vi "REPORT XLS PEDROLLO 2.vi"(6 "banco":i32=1, 8 "Report collaudo in corso?":bool, 9 "COLLAUDI DI CONFRONTO":string[](array[string]), 10 "COLLAUDO PRINCIPALE":string) -> ()   [LabVIEW 2019]
uses:
  TypeDef/custom plot legend.ctl
  TypeDef/Grafico report.ctl
  TypeDef/Definizione_Grafico_REPORT.ctl
  TypeDef/Definizione_plot.ctl
  <vilib>/Utility/miscctls.llb/LVRowAndColumnTypeDef.ctl
  Global percorso impostazioni.vi
  <vilib>/Utility/file.llb/Read Delimited Spreadsheet (string).vi
  <vilib>/Utility/file.llb/Read From Spreadsheet File (string).vi
  <vilib>/addons/_office/excel.llb/Excel Easy Table (str).vi
  <vilib>/Utility/file.llb/Write Delimited Spreadsheet (string).vi
  <vilib>/Utility/NIReport.llb/Append Image to Report (path wrap).vi
  <vilib>/addons/database/_DB Variant To Data/Database Variant To Data.xnode
  <vilib>/Utility/NIReport.llb/NI_report.lvclass
  <vilib>/addons/_office/NI_ReportGenerationToolkit.lvlib
  <vilib>/Utility/NIReport.llb/Excel/NI_Excel.lvclass
  <vilib>/addons/database/NI_Database_API.lvlib
panel:
  out "Tipo report":bool
  in  "TABELLA RES FREDDO RES METER":i32(listbox) caption="MISURE RESISTENZE A FREDDO"
  out "state":string
  out "Numeric 2":i32
  out "scelta grafico":u16
  out "modifica":bool
  in  "EXCEL":bool=TRUE
  in  "PDF":bool
  in  "salva impostazioni grafici":bool
  out "ID Colleg confronti":i32[](array[numeric])
  in  "AGGIORNA IMM":bool
  out "Numeric":i32
  in  "Slide":dbl(slide) scale=0.0..100.0
  out "Cartella modello":path
  in  "REPORT C2K":bool caption="C2K"
  out "element":string
  in  "stile punto":u16(ring)
  in  "stile linea":u16(ring)
  in  "Larghezza linea":u16(ring)
  in  "input cluster":T1
  out "ProvaT-DT":cluster{"X":dbl[], "Y":dbl[]}[](graph)
  out "ProvaT-TC":cluster{"X":dbl[], "Y":dbl[]}[](graph)
  out "Legenda 2":T2
  in  "PLOT LEGEND T-TC":T3[](array[typedef]) {"Collegamento" items=["TRIFASE"]}
  in  "PLOT LEGEND T-DT":T3[](array[typedef]) {"Collegamento" items=["TRIFASE"]}
  in  "PLOT LEGEND QH-QH 2":T3[](array[typedef]) {"Collegamento" items=["TRIFASE"]}
  out "ETICHETTE":string[](array[string])
  in  "scelta grafico SCORTA 3":u16(ring)
  in  "scelta grafico SCORTA 2":u16(ring)
  in  "scelta grafico SCORTA 1":u16(ring) items=["Termica RESISTOMAT", "TEST TAB RESISTOMAT"]
  in  "scelta grafico GENERICA":u16(ring)
  in  "scelta grafico A CARICO":u16(ring) items=["Test a Carico"]
  in  "scelta grafico A VUOTO":u16(ring) items=["Test a Vuoto", "CosPhi"]
  in  "scelta grafico TERMICA":u16(ring) items=["Termica RESISTOMAT", "T Cassa", "Potenza", "T Cuscinetti"]
  in  "scelta grafico ROTORE BLOCC":u16(ring)
  in  "scelta grafico CMECC":u16(ring)=1 items=["C-RPM", "Caratt.mecc."]
  out "Plots":T4[](array[typedef]) {"PLOT"."GRANDEZZA Y" items=["Banco", "Anno", "Numero", "N° tabella", "Misura", "Tipo prova", "Progressivo Acq", "tempo[h:m:s]", "tempo acq[min]", "f [Hz]", "Uav [V]", "Iav [A]", "Tq [Nm]", "n [rpm]", "P1 [kW]", "P1 n[kW]", "Q [m3/h]", "Q n[m3/h]", "Q [l/min]", "Q n[l/min]", "H1 [m]", "Dislivello [m]", "Hdinamica [m]", "HvAsp [m]", "HvMand [m]", "HvTot [m]", "H2 [m]", "Htot [m]", "Htot n[m]", "P3 (Phyd) [kW]", "P3 (Phyd) n[kW]", "P2 [kW]", "P2 n[kW]", "P2 n ps[kW]", "eta motore [%]", "eta pompa [%]", "eta pompa n[%]", "eta gruppo [%]", "eta gruppo n[%]", "T acqua [°C]", "Densità liquido [kg/m3]", "P barometrica [mbar]", "pf", "Uch1 [V]", "Uch2 [V]", "Uch3 [V]", "Ich1 [A]", "Ich2 [A]", "Ich3 [A]", "Temp.amb[°C]", "Ru-w [ohm]", "DTavvolg. [°C]", "Tamb Freddo [°C]", "Ru-w Freddo [ohm]", "Tc1[°C]", "Tc2[°C]", "Tc3[°C]", "Tc4[°C]", "Tc5", "Tc6", "Tc7", "Tc8", "H1[Bar]", "H2[bar]", "P premist.[Bar]", "Pserb[bar]", "n°NPSH", "NPSH", "Htot Ref[m]", "NPSH_%caduta", "%caduta", "Qref [m3/h]", "MEI"]; "PLOT"."GRANDEZZA X" items=["Banco", "Anno", "Numero", "N° tabella", "Misura", "Tipo prova", "Progressivo Acq", "tempo[h:m:s]", "tempo acq[min]", "f [Hz]", "Uav [V]", "Iav [A]", "Tq [Nm]", "n [rpm]", "P1 [kW]", "P1 n[kW]", "Q [m3/h]", "Q n[m3/h]", "Q [l/min]", "Q n[l/min]", "H1 [m]", "Dislivello [m]", "Hdinamica [m]", "HvAsp [m]", "HvMand [m]", "HvTot [m]", "H2 [m]", "Htot [m]", "Htot n[m]", "P3 (Phyd) [kW]", "P3 (Phyd) n[kW]", "P2 [kW]", "P2 n[kW]", "P2 n ps[kW]", "eta motore [%]", "eta pompa [%]", "eta pompa n[%]", "eta gruppo [%]", "eta gruppo n[%]", "T acqua [°C]", "Densità liquido [kg/m3]", "P barometrica [mbar]", "pf", "Uch1 [V]", "Uch2 [V]", "Uch3 [V]", "Ich1 [A]", "Ich2 [A]", "Ich3 [A]", "Temp.amb[°C]", "Ru-w [ohm]", "DTavvolg. [°C]", "Tamb Freddo [°C]", "Ru-w Freddo [ohm]", "Tc1[°C]", "Tc2[°C]", "Tc3[°C]", "Tc4[°C]", "Tc5", "Tc6", "Tc7", "Tc8", "H1[Bar]", "H2[bar]", "P premist.[Bar]", "Pserb[bar]", "n°NPSH", "NPSH", "Htot Ref[m]", "NPSH_%caduta", "%caduta", "Qref [m3/h]", "MEI"]; "Assi grafico"."ASSE X" items=["X 1", "X 2"]; "Assi grafico"."ASSE Y" items=["Y 1", "Y 2", "Y 3", "Y 4"]}
  out "Grafici":T5[](array[typedef]) {"ASSE Y 5"."Decimali" min=0 max=6; "ASSE Y 4"."Decimali" min=0 max=6; "ASSE Y 3"."Decimali" min=0 max=6; "ASSE Y 2"."Decimali" min=0 max=6; "ASSE Y 1"."Decimali" min=0 max=6; "ASSE X 2"."Decimali" min=0 max=6; "ASSE X 1"."Decimali" min=0 max=6}
  in  "toll Q":dbl format="+/- %#_g %"
  in  "toll H":dbl format="+/- %#_g %"
  in  "toll P2":dbl format="+ %#_g %"
  in  "PLOT LEGEND QH-QH":T3[](array[typedef]) {"Collegamento" items=["TRIFASE"]}
  in  "PLOT LEGEND QH-QRPM":T3[](array[typedef]) {"Collegamento" items=["TRIFASE"]}
  in  "PLOT LEGEND QH-QP2":T3[](array[typedef]) {"Collegamento" items=["TRIFASE"]}
  out "ProvaQH-QH":cluster{"X":dbl[], "Y":dbl[]}[](graph)
  out "Legenda":T2
  out "Array 3":picture[](array[picture])
  in  "TABELLA SCORTA 2":i32(listbox)
  in  "TABELLA SCORTA 3":i32(listbox)
  out "ID COLLEGAMENTO":i32
  out "cambia taratura":bool=TRUE
  in  "VISUALIZZA TABELLA":i8=1 caption="VISUALIZZA TABELLA:" min=1 max=10
  in  "REPORT EXCEL":bool caption="REPORT"
  in  "Percorso report di DEFAULT":path=path "C:/Lavori_in_corso_Tecnico4/C2017010 Pedrollo sala prove/Codice/Report"
  in  "grafica tutte":bool
  in  "TABELLA 2NPSH":i32(listbox)
  in  "TABELLA 3 NPSH":i32(listbox)
  out "carica grafici":bool=TRUE
  out "Case carica grafici":string
  out "Legenda dt":T2
  out "picture T tc":picture
  out "picture T Dt":picture
  out "picture QH QP2Etap":picture
  out "picture QH Qrpm":picture
  out "picture QH QH":picture
  out "picture legenda":picture
  in  "VISUALIZZA TABELLA 0":T6(radio) caption="VISUALIZZA TABELLA"
  out "tipo prova":string
  out "trifase?":bool
  out "update annotation":bool=TRUE
  out "Nomi colonne":string[](array[string])
  in  "GRAFICA":bool
  in  "exit":bool
  in  "carica collaudi di confronto":bool
  in  "Tab Control":T7(tab)
  in  "Descrizione princ":string caption="Descrizione"
  in  "Descrizione":string[](array[string])
  out "Dati collaudo principale":i32[](listbox)
  in  "CERCA COLLAUDO DI CONFRONTO":bool
  in  "CERCA COLLAUDO":bool
  in  "CARICA COLLAUDI":bool
  in  "SCELTA MODELLO XLS":i32(listbox)
  out "Boolean":bool=TRUE
  in  "TABELLA A VUOTO":i16=1 min=1 max=10
  in  "TABELLA A VUOTO":i32(listbox)
  in  "Res FINE prova VUOTO":i32(listbox)
  in  "Res INIZIO prova VUOTO":i32(listbox)
  in  "Array Grafici A VUOTO":T8[](array[typedef]) {"Esporta xls"."Zoom" min=0 max=1; "scelta grafico A VUOTO 2" items=["Test a Vuoto", "CosPhi"]}
  in  "Array Grafici A CARICO":T8[](array[typedef]) {"Esporta xls"."Zoom" min=0 max=1; "scelta grafico A VUOTO 2" items=["Test a Carico"]}
  in  "TABELLA A CARICO":i16=1 min=1 max=10
  in  "TABELLA A CARICO":i32(listbox)
  in  "Res FINE prova CARICO":i32(listbox)
  in  "Res INIZIO prova CARICO":i32(listbox)
  in  "TABELLA TERMICA":i16=1 min=1 max=10
  in  "TABELLA TERMICA":i32(listbox) caption="ACQUISIZIONI RISCALDAMENTO"
  in  "TABELLA EQ TERMICO":i32(listbox) caption="MISURE RESISTENZE A FREDDO"
  in  "TABELLA RES FREDDO RESISTOMAT":i32(listbox) caption="MISURE RESISTENZE A FREDDO"
  in  "Array Grafici TERMICA":T8[](array[typedef]) {"Esporta xls"."Zoom" min=0 max=1; "scelta grafico A VUOTO 2" items=["Termica RESISTOMAT", "T Cassa", "Potenza", "T Cuscinetti"]}
  in  "TABELLA RES TERMICA":i32(listbox) caption="TABELLA RESISTENZE TERMICA"
  in  "TABELLA CMECC":i16=1 min=1 max=10
  in  "TABELLA C MECC":i32(listbox) caption="TABELLA CARATTERISTICA MECCANICA"
  in  "Array Grafici CMECC":T8[](array[typedef]) {"Esporta xls"."Zoom" min=0 max=1; "scelta grafico A VUOTO 2" items=["C-RPM", "Caratt.mecc."]}
  in  "TABELLA COPPIA MAX":i32(listbox)
  in  "TABELLA A ROT BLOCC":i16=1 min=1 max=10
  in  "TABELLA ROT BLOCC":i32(listbox) caption="TABELLA ROTORE BLOCCATO"
  in  "TABELLA I SPUNTO":i32(listbox)
  in  "Array Grafici ROTBLOCC":T8[](array[typedef]) {"Esporta xls"."Zoom" min=0 max=1; "scelta grafico A VUOTO 2" items=["Termocoppie", "DeltaT", "Time-Power", "Time-Power-current"]}
  in  "TABELLA GENERICA":i16=1 min=1 max=10
  in  "TABELLA GENERICA":i32(listbox)
  in  "Array Grafici GENERICA":T8[](array[typedef]) {"Esporta xls"."Zoom" min=0 max=1; "scelta grafico A VUOTO 2" items=["PROVA A VUOTO"]}
  out "Coefficiente di correlazione":dbl
  out "DETERMINAZIONE DEL RENDIMENTO":i32[](listbox)=[1] caption="DETERMINAZIONE DEL RENDIMENTO secondo IEC EN 60034-1"
  in  "Tab Control 2":T9(tab)
  in  "Foglio attivo pdf eng":i16
  in  "Foglio attivo pdf ita":i16
  in  "Foglio attivo xls":i16
  in  "PDF INGL 2":bool
  in  "PDF ITA 2":bool
  in  "EXCEL 2":bool
  in  "Modifica percorso default":bool
  in  "Percorso e nome di DEFAULT":i32(listbox)
  in  "Elimina criterio":bool
  in  "Aggiungi criterio":bool
  in  "Criteri di salvataggio report":i32(listbox)
  in  "Percorso modelli xls":path=path "C:/Lavori_in_corso_Tecnico4/C2017010 Pedrollo sala prove/Codice/Report"
  in  "sep. decimale numeri esportati":enum16{"Virgola", "Punto"}(ring)=enum."Punto"
  in  "SALVA COME DEFAULT":bool
  in  "IMPOSTAZIONI GRAFICI":bool
  in  "Stili grafico":T10={"Stile grafici Tabella 1"={"Larghezza linea"=2, "stile linea"=0, "stile punto"=2}, "Stile grafici Tabella 2"={"Larghezza linea"=2, "stile linea"=0, "stile punto"=5}, "Stile grafici Tabella 3"={"Larghezza linea"=2, "stile linea"=0, "stile punto"=13}, "Colore collaudo report"=0, "Colore collaudo confronto 1"=16860, "Colore collaudo confronto 2"=1985280, "Colore collaudo confronto 3"=16730368, "Colore collaudo confronto 4"=6062714, "Colore collaudo confronto 5"=13107389, "Stile croci"={"Larghezza linea"=3, "stile linea"=0, "stile punto"=0, "colore"=16711680}}
  in  "colori grafici":T11={"Griglie maggiori"=13224393, "Griglie minori"=13816530, "sfondo"=16448250}
  in  "Carica impostazioni modello":bool
  in  "SCEGLI MODELLO":string(combo)
  in  "Nome fogli GENERICHE":T12(array[cluster])
  in  "Nome fogli":T13(array[cluster])=[{"Nome prova"=enum."DATI BOLLETTINO", "Nome foglio nascosto xls"="DT_Res_RB", "Cella iniziale"={"row"=0, "column"=0}}, {"Nome prova"=enum."RESISTENZE FREDDO", "Nome foglio nascosto xls"="DT_Res_RB", "Cella iniziale"={"row"=6, "column"=0}}, {"Nome prova"=enum."RIGA DATI I SPUNTO", "Nome foglio nascosto xls"="DT_Res_RB", "Cella iniziale"={"row"=10, "column"=0}}, {"Nome prova"=enum."DATI ROTORE BLOCCATO", "Nome foglio nascosto xls"="DT_Res_RB", "Cella iniziale"={"row"=15, "column"=0}}, {"Nome prova"=enum."RES INIZIO PROVA VUOTO", "Nome foglio nascosto xls"="Vuoto", "Cella iniziale"={"row"=0, "column"=0}}, {"Nome prova"=enum."RES FINE PROVA VUOTO", "Nome foglio nascosto xls"="Vuoto", "Cella iniziale"={"row"=6, "column"=0}}, {"Nome prova"=enum."DATI PROVA A VUOTO", "Nome foglio nascosto xls"="Vuoto", "Cella iniziale"={"row"=11, "column"=0}}, {"Nome prova"=enum."RES INIZIO PROVA A CARICO", "Nome foglio nascosto xls"="Carico", "Cella iniziale"={"row"=0, "column"=0}}, {"Nome prova"=enum."RES FINE PROVA A CARICO", "Nome foglio nascosto xls"="Carico", "Cella iniziale"={"row"=6, "column"=0}}, {"Nome prova"=enum."DATI PROVA A CARICO", "Nome foglio nascosto xls"="Carico", "Cella iniziale"={"row"=11, "column"=0}}, {"Nome prova"=enum."RIGA DATI I SPUNTO", "Nome foglio nascosto xls"="CMecc", "Cella iniziale"={"row"=0, "column"=0}}, {"Nome prova"=enum."RIGA DATI CMAX", "Nome foglio nascosto xls"="CMecc", "Cella iniziale"={"row"=6, "column"=0}}] caption="CRITERI DI ESPORTAZIONE PROVE"
  in  "SALVA IMPOSTAZIONI ESP MODELLO":bool
  in  "carica collaudo in corso":bool
  # "CONTROLLI IMMAGINI DI SUPPORTO"
  # "TOLLERANZE CROCI"
  # "CREAZIONE\nREPORT IN\nCORSO..."
  # "Stile linea"
  # "Stile punto"
  # "PLOT"
  # "GESTIONE PLOT"
  # "COLLEGAMENTO"
  # "ASSI GRAFICO"
  # "PLOT"
  # "GESTIONE PLOT"
  # "COLLEGAMENTO"
  # "ASSI GRAFICO"
  # "PLOT"
  # "GESTIONE PLOT"
  # "COLLEGAMENTO"
  # "ASSI GRAFICO"
  # "PLOT"
  # "GESTIONE PLOT"
  # "COLLEGAMENTO"
  # "ASSI GRAFICO"
  # "PLOT"
  # "GESTIONE PLOT"
  # "COLLEGAMENTO"
  # "ASSI GRAFICO"
  # "PLOT"
  # "GESTIONE PLOT"
  # "COLLEGAMENTO"
  # "ASSI GRAFICO"
  # "Stile linea"
  # "Stile punto"
  # "Stile linea"
  # "Stile punto"
  # "*NOTA: i modelli che contengono\nnel proprio nome la stringa\n\"GESTIONALE\" esportano il report\nnella cartella di condivisione con\nil gestionale"
  # "ESPORTAZIONE DI DEFAULT"
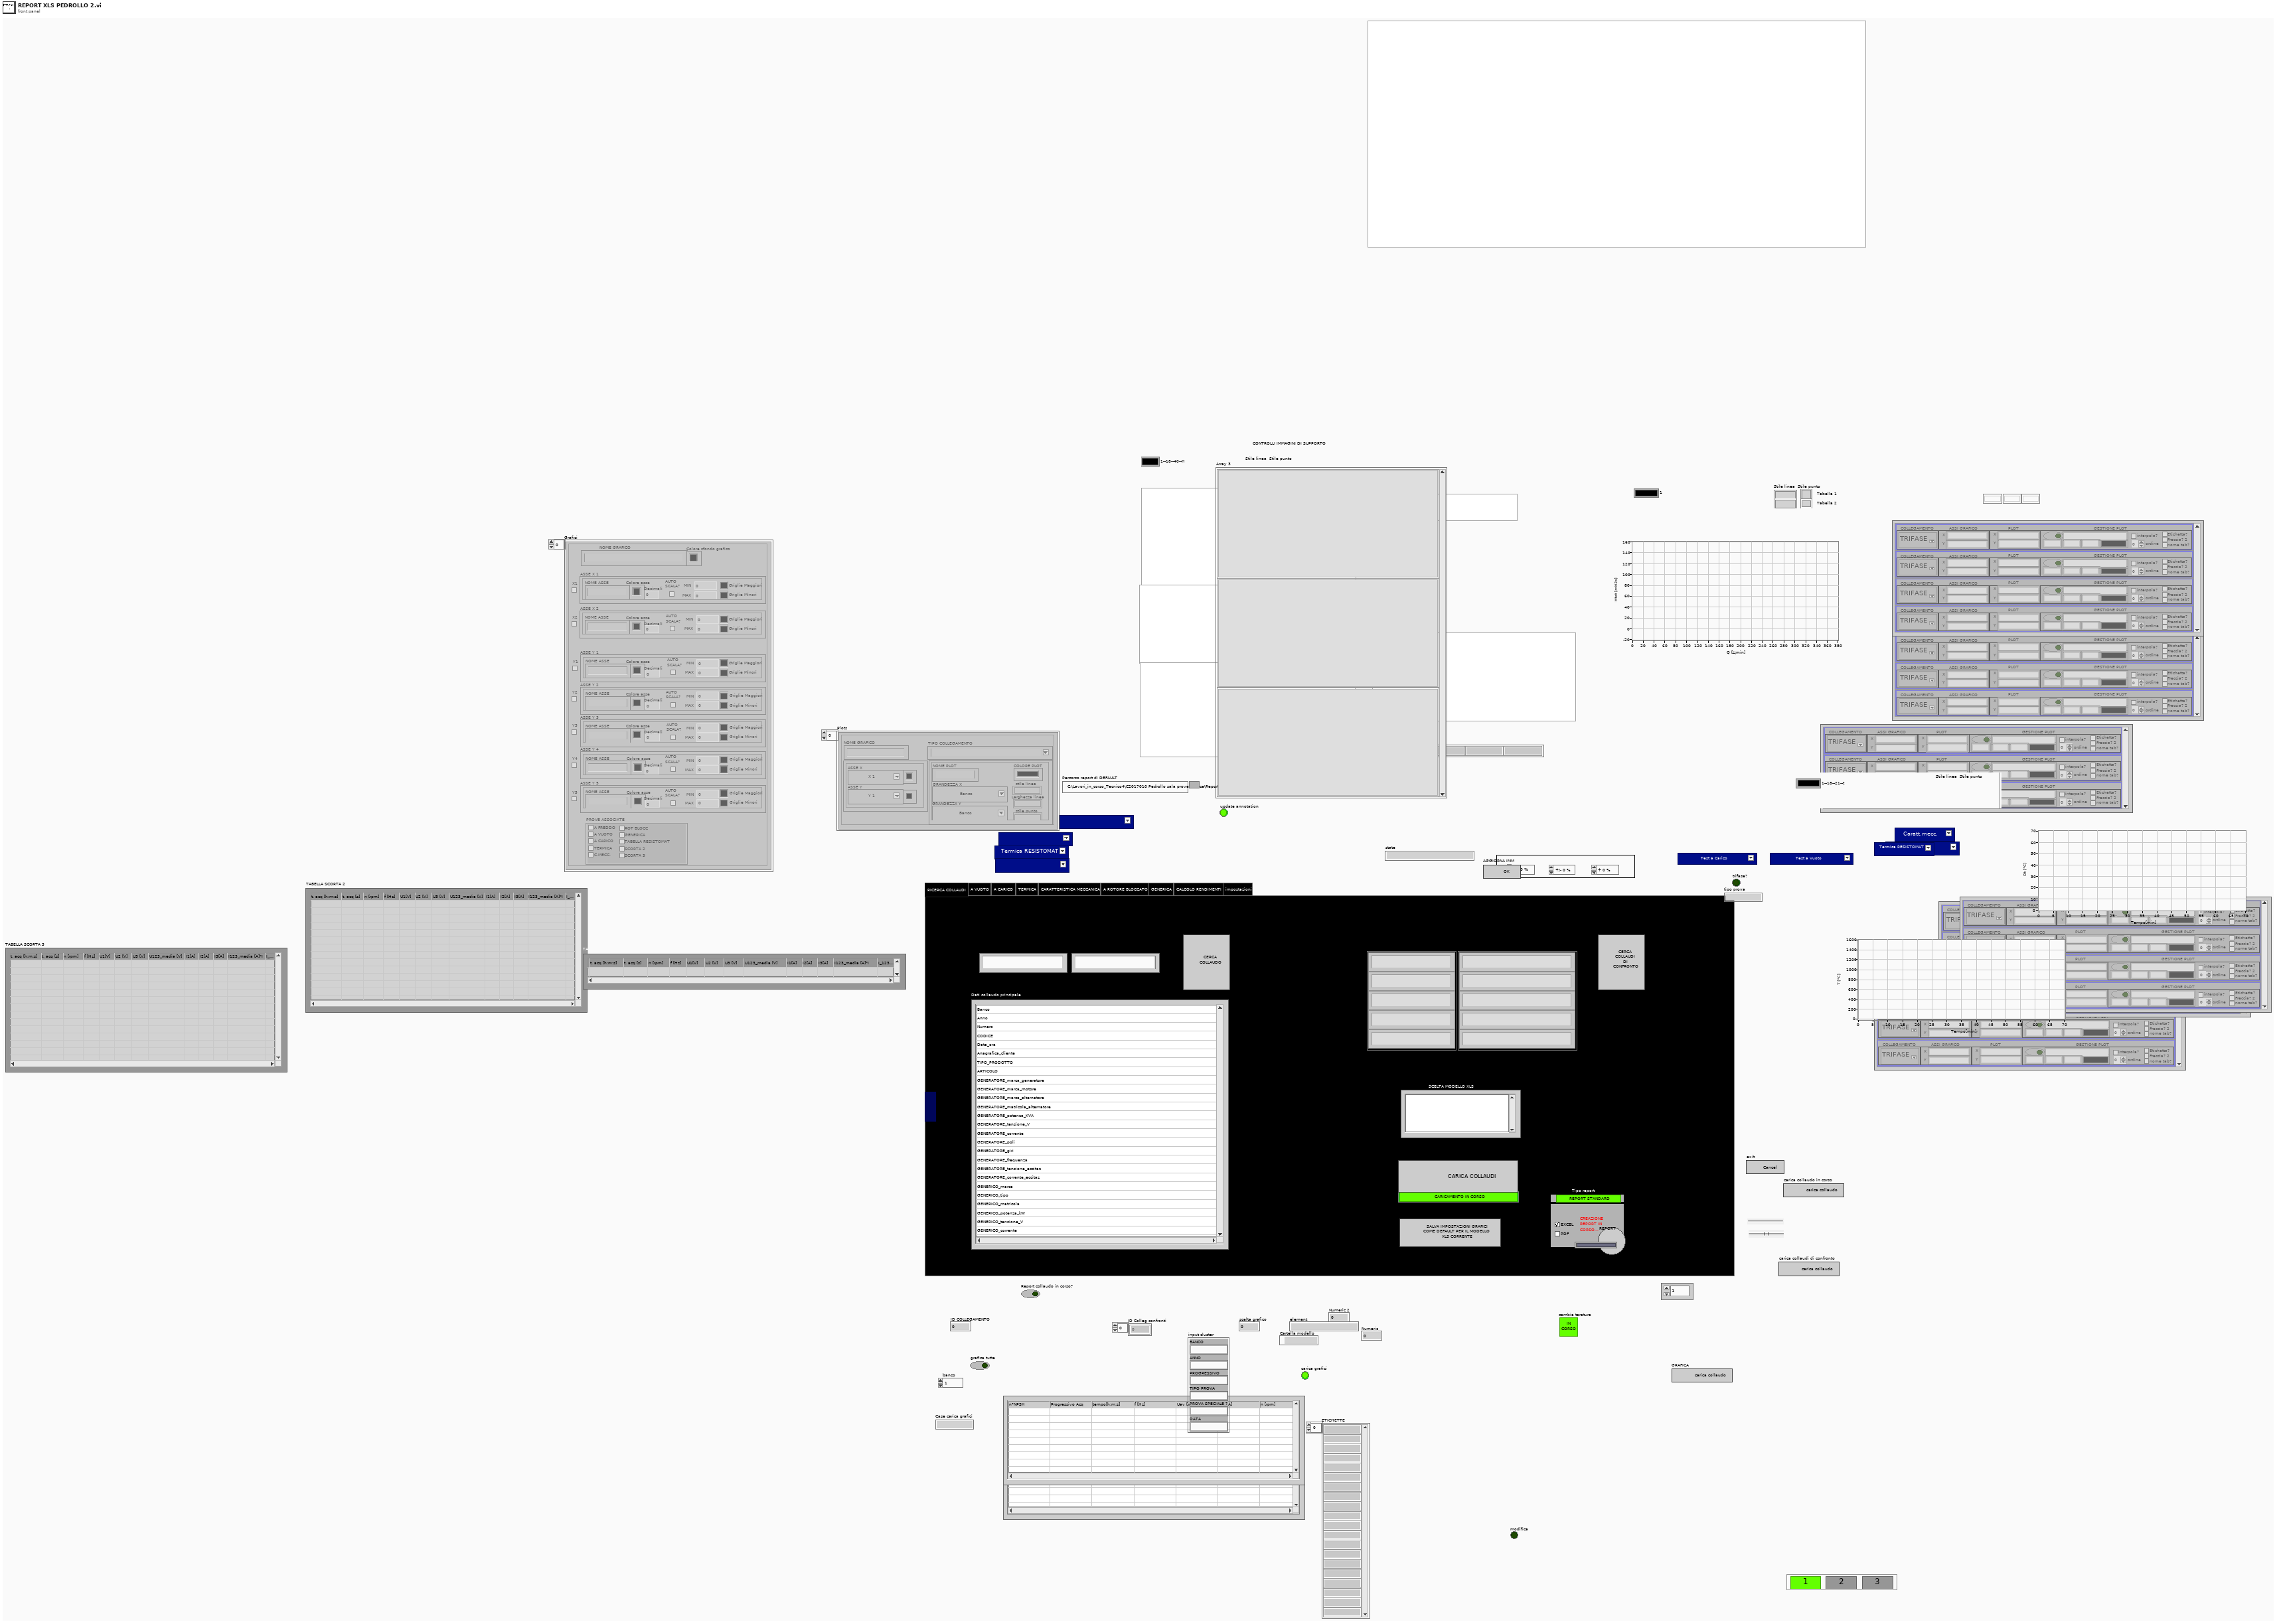
[diagram p1: front panel]
types:
  T1 = cluster{"BANCO":string, "ANNO":string, "PROGRESSIVO":string, "TIPO PROVA":string, "PROVA SPECIALE ?":string, "DATA":string}
  T2 = cluster{"Colore collaudo report 6":u32, "Colore collaudo report":u32, "Colore collaudo report 2":u32, "Colore collaudo report 3":u32, "Colore collaudo report 4":u32, "Colore collaudo report 5":u32, "Tabella 1":cluster{"stile linea":u16, "stile punto":u16}, "Tabella 2":cluster{"stile linea":u16, "stile punto":u16}, "Tabella 3":cluster{"stile linea":u16, "stile punto":u16}}
  T3 = typedef "custom plot legend.ctl" = cluster{"nome plot":string, "colore":u32, "Larghezza linea":u16, "stile linea":u16, "stile punto":u16, "Visibile?":bool, "interpola?":bool, "ordine":dbl, "ScalaY":dbl, "Etichetta?":bool, "Freccia? 2":bool, "nome tab?":bool, "Asse Y grafico":string, "Asse X grafico":string, "Grandezza X":string, "Grandezza Y":string, "Collegamento":u16}
  T4 = typedef "Definizione_plot.ctl" = cluster{"Assi grafico":cluster{"ASSE Y":u16, "ASSE X":u16, "Colore x":u32, "Colore y":u32}, "TIPO COLLEGAMENTO":string, "PLOT":cluster{"GRANDEZZA X":u16, "GRANDEZZA Y":u16, "COLORE PLOT":u32, "NOME PLOT":string, "Larghezza linea":u16, "stile linea":u16, "stile punto":u16}, "NOME GRAFICO":string}
  T5 = typedef "Definizione_Grafico_REPORT.ctl" = cluster{"ASSE X 1":cluster{"NOME ASSE":string, "AUTO\nSCALA?":bool, "MIN":dbl, "MAX":dbl, "Colore asse":u32, "Griglie Maggiori":u32, "Griglie Minori":u32, "Decimali":i8}, "ASSE X 2":cluster{"NOME ASSE":string, "AUTO\nSCALA?":bool, "MIN":dbl, "MAX":dbl, "Colore asse":u32, "Griglie Maggiori":u32, "Griglie Minori":u32, "Decimali":i8}, "ASSE Y 1":cluster{"NOME ASSE":string, "AUTO\nSCALA?":bool, "MIN":dbl, "MAX":dbl, "Colore asse":u32, "Griglie Maggiori":u32, "Griglie Minori":u32, "Decimali":i8}, "ASSE Y 2":cluster{"NOME ASSE":string, "AUTO\nSCALA?":bool, "MIN":dbl, "MAX":dbl, "Colore asse":u32, "Griglie Maggiori":u32, "Griglie Minori":u32, "Decimali":i8}, "ASSE Y 3":cluster{"NOME ASSE":string, "AUTO\nSCALA?":bool, "MIN":dbl, "MAX":dbl, "Colore asse":u32, "Griglie Maggiori":u32, "Griglie Minori":u32, "Decimali":i8}, "ASSE Y 4":cluster{"NOME ASSE":string, "AUTO\nSCALA?":bool, "MIN":dbl, "MAX":dbl, "Colore asse":u32, "Griglie Maggiori":u32, "Griglie Minori":u32, "Decimali":i8}, "X1":bool, "X2":bool, "Y1":bool, "Y2":bool, "Y3":bool, "Y4":bool, "NOME GRAFICO":string, "PROVE ASSOCIATE":cluster{"A FREDDO":bool, "A VUOTO":bool, "A CARICO":bool, "TERMICA":bool, "C.MECC.":bool, "ROT BLOCC":bool, "GENERICA":bool, "TABELLA RESISTOMAT":bool, "SCORTA 2":bool, "SCORTA 3":bool}, "ASSE Y 5":cluster{"NOME ASSE":string, "AUTO\nSCALA?":bool, "MIN":dbl, "MAX":dbl, "Colore asse":u32, "Griglie Maggiori":u32, "Griglie Minori":u32, "Decimali":i8}, "Y5":bool, "Colore sfondo grafico":u32}
  T6 = enum32{"Radio Selection 1", "Radio Selection 2", "Radio Selection 3"}
  T7 = enum32{"RICERCA COLLAUDI", "A VUOTO", "A CARICO", "TERMICA", "CARATTERISTICA MECCANICA", "A ROTORE BLOCCATO", "GENERICA", "CALCOLO RENDIMENTI", "impostazioni"}
  T8 = typedef "Grafico report.ctl" = cluster{"2D Picture":picture, "Aggiungi grafico":bool, "Settings grafico":bool, "Elimina grafico":bool, "scelta grafico A VUOTO 2":u16, "Esporta xls":cluster{"Esporta?":bool, "Impostazioni esport.":cluster{"position (Excel)":cluster{"row":i32, "column":i32}, "Nome foglio (Excel)":string, "bookmark (Word)":string}, "Zoom ":sgl, "Ruota immagine":enum16{"miror", "rotate 0°", "rotate 90°", "rotate 180°", "rotate 270°"}}}
  T9 = enum32{"GENERALI", "GRAFICI ", "CRITERI DI ESPORTAZIONE NEI FOGLI NASCOSTI"}
  T10 = cluster{"Stile grafici Tabella 1":cluster{"Larghezza linea":u16, "stile linea":u16, "stile punto":u16}, "Stile grafici Tabella 2":cluster{"Larghezza linea":u16, "stile linea":u16, "stile punto":u16}, "Stile grafici Tabella 3":cluster{"Larghezza linea":u16, "stile linea":u16, "stile punto":u16}, "Colore collaudo report":u32, "Colore collaudo confronto 1":u32, "Colore collaudo confronto 2":u32, "Colore collaudo confronto 3":u32, "Colore collaudo confronto 4":u32, "Colore collaudo confronto 5":u32, "Stile croci":cluster{"Larghezza linea":u16, "stile linea":u16, "stile punto":u16, "colore":u32}}
  T11 = cluster{"Griglie maggiori":u32, "Griglie minori":u32, "sfondo":u32}
  T12 = cluster{"Nome prova":string, "Nome foglio nascosto xls":string, "Cella iniziale":cluster{"row":i32, "column":i32}}[]
  T13 = cluster{"Nome prova":enum16{"DATI BOLLETTINO", "RESISTENZE FREDDO", "RIGA DATI I SPUNTO", "DATI ROTORE BLOCCATO", "RES INIZIO PROVA VUOTO", "RES FINE PROVA VUOTO", "DATI PROVA A VUOTO", "RES INIZIO PROVA A CARICO", "RES FINE PROVA A CARICO", "DATI PROVA A CARICO", "DATI EQUILIBRIO TERMICO", "DATI PROVA TERMICA", "RESISTENZE PROVA TERMICA", "RIGA DATI CMAX", "DATI CMECCANICA", "LEGENDA COLLAUDI CONFRONTO", "CALCOLI RENDIMENTO"}, "Nome foglio nascosto xls":string, "Cella iniziale":cluster{"row":i32, "column":i32}}[]
  T14 = enum16{"open", "replace", "create", "open or create", "replace or create", "replace or create with confirmation"}
  T15 = cluster{"NPSH-H":cluster{"X":dbl[], "Y":dbl[]}[], "Q-NPSH":cluster{"X":dbl[], "Y":dbl[]}[]}
  T16 = cluster{"DT":cluster{"X":dbl[], "Y":dbl[]}[], "TC":cluster{"X":dbl[], "Y":dbl[]}[]}
  T17 = cluster{"QH":cluster{"X":dbl[], "Y":dbl[]}[], "QRPM":cluster{"X":dbl[], "Y":dbl[]}[], "QP2":cluster{"X":dbl[], "Y":dbl[]}[]}
  T18 = enum32{"Invalid", "Standard", "Closed", "Hidden", "Minimized", "Maximized"}
  T19 = typedef "Indici.ctl" = cluster{"Q":i32, "Htot":i32, "NPSH":i32, "P3":i32, "etap":i32, "temperature":cluster{"DT":i32, "DTmarcia":i32, "DTaux":i32, "TC1":i32, "TC2":i32, "TC3":i32, "TC4":i32}, "tempo":i32, "P2":i32, "P1":i32, "etaGr":i32, "RPM":i32}
  T20 = cluster{"Nome fogli":cluster{"Nome prova":enum16{"DATI BOLLETTINO", "RESISTENZE FREDDO", "RIGA DATI I SPUNTO", "DATI ROTORE BLOCCATO", "RES INIZIO PROVA VUOTO", "RES FINE PROVA VUOTO", "DATI PROVA A VUOTO", "RES INIZIO PROVA A CARICO", "RES FINE PROVA A CARICO", "DATI PROVA A CARICO", "DATI EQUILIBRIO TERMICO", "DATI PROVA TERMICA", "RESISTENZE PROVA TERMICA", "RIGA DATI CMAX", "DATI CMECCANICA", "LEGENDA COLLAUDI CONFRONTO", "CALCOLI RENDIMENTO"}, "Nome foglio nascosto xls":string, "Cella iniziale":cluster{"row":i32, "column":i32}}[], "Nome fogli GENERICHE":cluster{"Nome prova":string, "Nome foglio nascosto xls":string, "Cella iniziale":cluster{"row":i32, "column":i32}}[]}
  T21 = cluster{"Array Grafici A VUOTO":T8[], "Array Grafici A CARICO":T8[], "Array Grafici TERMICA":T8[], "Array Grafici CMECC":T8[], "Array Grafici ROTBLOCC":T8[], "Array Grafici GENERICA":T8[]}
  T22 = typedef "LVRowAndColumnTypeDef.ctl" = cluster{"Row":i32, "Column":i32}
  T23 = enum16{"maximized", "minimized", "normal", "no change"}
  T24 = enum16{"Standard Report", "HTML", "Word", "Excel"}
  T25 = cluster{"position (Excel)":cluster{"row":i32, "column":i32}, "name (Excel)":string, "bookmark (Word)":string}
  T26 = typedef "NI_Database_API.lvlib/Conn ObjectReference.ctl" = refnum<k1>
  T27 = typedef "Dati collaudo.ctl" = cluster{"nome collaudo":string, "Res freddo res meter":string[][], "Res freddo resistomat":string[][], "A vuoto":string[][], "A carico":string[][], "Termica":string[][], "Cmecc":string[][], "Rbloccato":string[][], "Generica":string[][], "Resistenze termica":string[][], "Scorta2":string[][], "Scorta3":string[][], "Riga eq termico":string[][], "Riga Cmax":string[][], "Riga Ispunto":string[][], "Res ini vuoto":string[][], "Res fin vuoto":string[][], "Res ini carico":string[][], "Res fin carico":string[][], "scorta tipizz 1":string[][], "scorta tipizz 2":string[][], "scorta tipizz 3":string[][]}
  T28 = typedef "imagedata.ctl" = cluster{"image type":i32, "image depth":i32, "image":u8[], "mask":u8[], "colors":u32[], "Rectangle":cluster{"left":i16, "top":i16, "right":i16, "bottom":i16}}
  T29 = typedef "LVBoundsTypeDef.ctl" = cluster{"Width":u32, "Height":u32}
  T30 = cluster{"Larghezza linea":u16, "stile linea":u16, "stile punto":u16}
  T31 = cluster{"Larghezza linea":u16, "stile linea":u16, "stile punto":u16, "colore":u32}
  T32 = cluster{"nomi plot":string[], "plot":cluster{"X":dbl[], "Y":dbl[]}[], "#collaudo":i32}
  T33 = cluster{"Larghezza linea":u16, "stile linea":u16, "stile punto":u16}[]
  T34 = cluster{"nomi plot":string[], "plot":cluster{"X":dbl[], "Y":dbl[]}[], "#collaudo":i32}[]
  T35 = enum16{"miror", "rotate 0°", "rotate 90°", "rotate 180°", "rotate 270°"}
  T36 = cluster{"position (Excel)":cluster{"row":i32, "column":i32}, "Nome foglio (Excel)":string, "bookmark (Word)":string}
  T37 = cluster{"path":path, "Impostazioni esport.":cluster{"position (Excel)":cluster{"row":i32, "column":i32}, "Nome foglio (Excel)":string, "bookmark (Word)":string}}
  T38 = enum16{"DATI BOLLETTINO", "RESISTENZE FREDDO", "RIGA DATI I SPUNTO", "DATI ROTORE BLOCCATO", "RES INIZIO PROVA VUOTO", "RES FINE PROVA VUOTO", "DATI PROVA A VUOTO", "RES INIZIO PROVA A CARICO", "RES FINE PROVA A CARICO", "DATI PROVA A CARICO", "DATI EQUILIBRIO TERMICO", "DATI PROVA TERMICA", "RESISTENZE PROVA TERMICA", "RIGA DATI CMAX", "DATI CMECCANICA", "LEGENDA COLLAUDI CONFRONTO", "CALCOLI RENDIMENTO"}
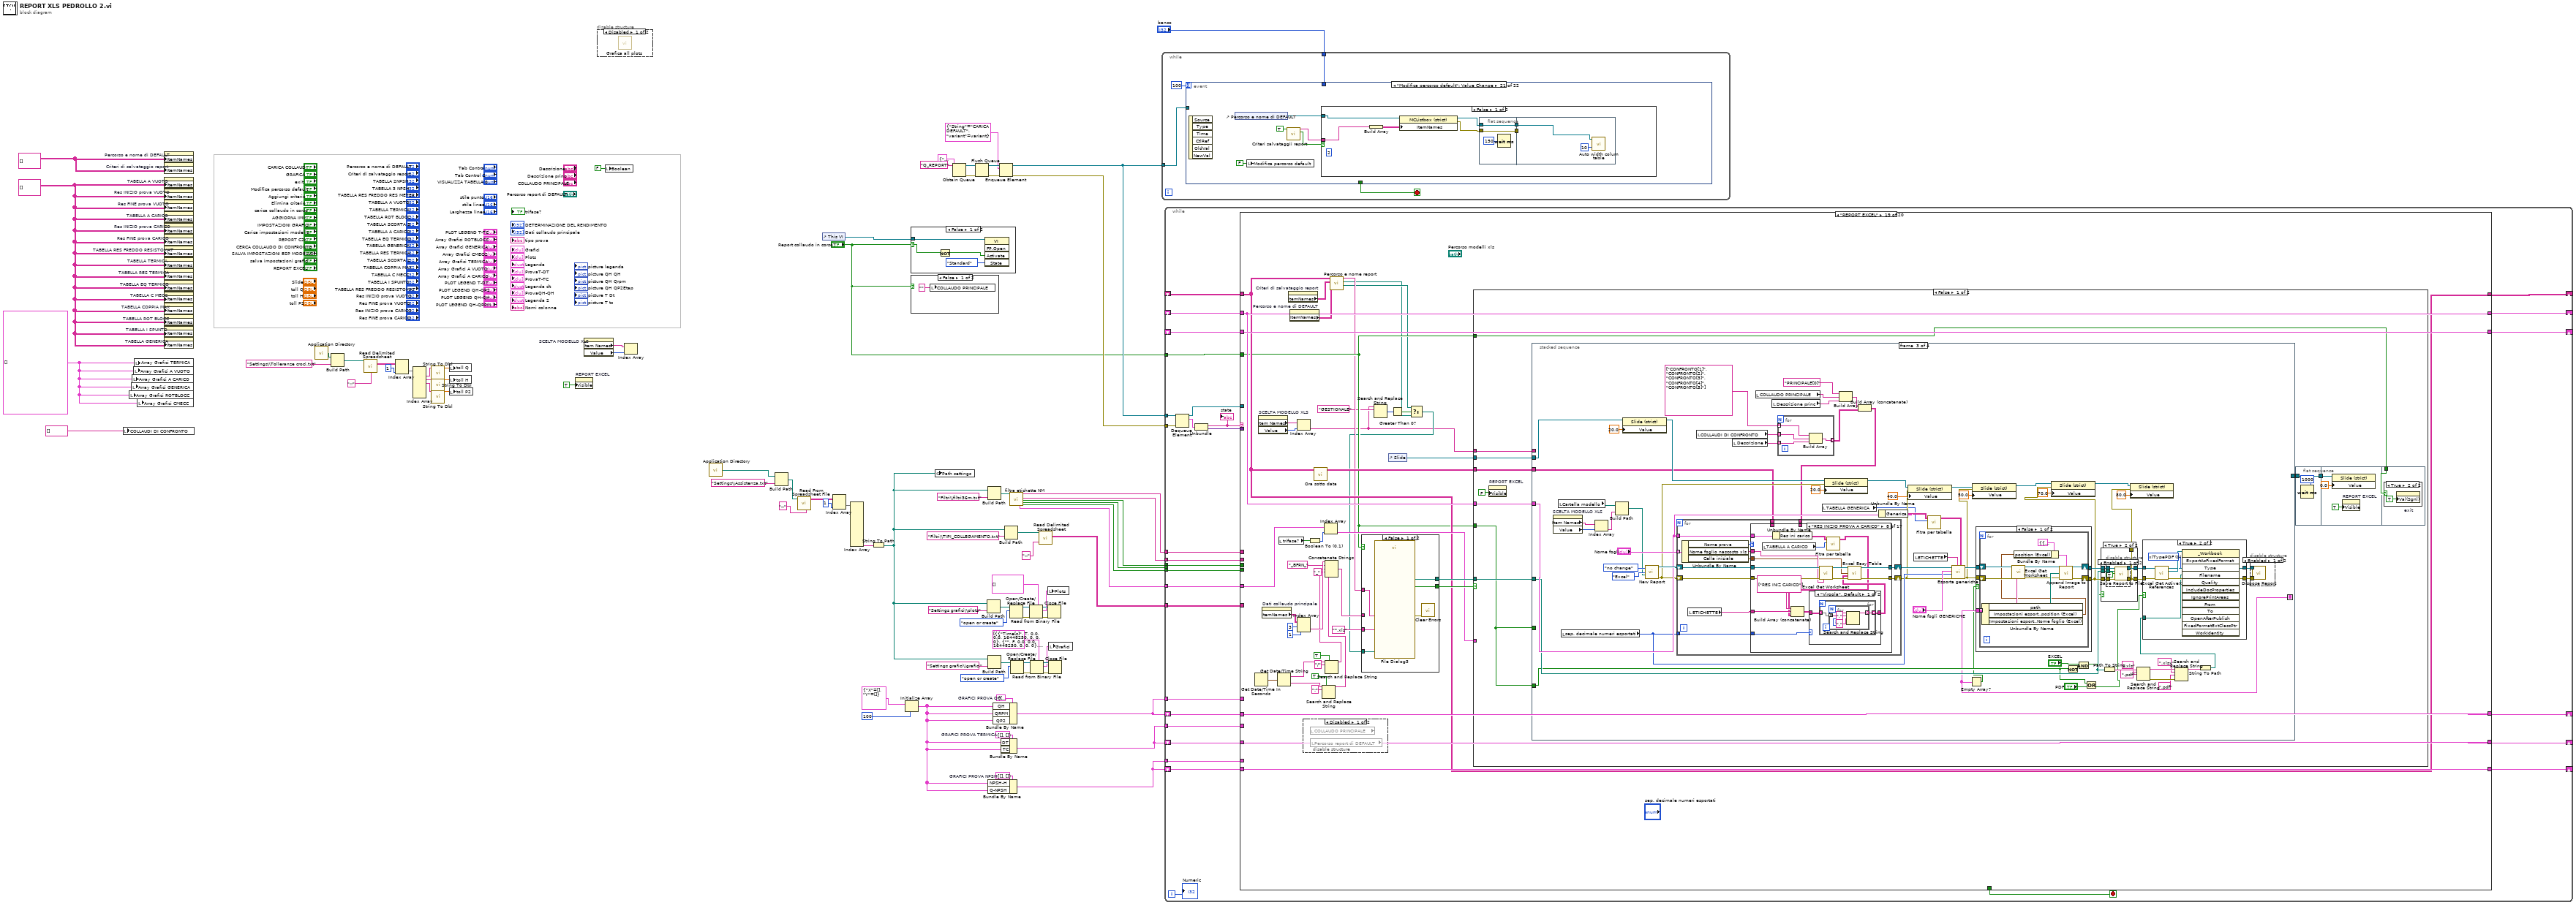
[diagram p0: block diagram]
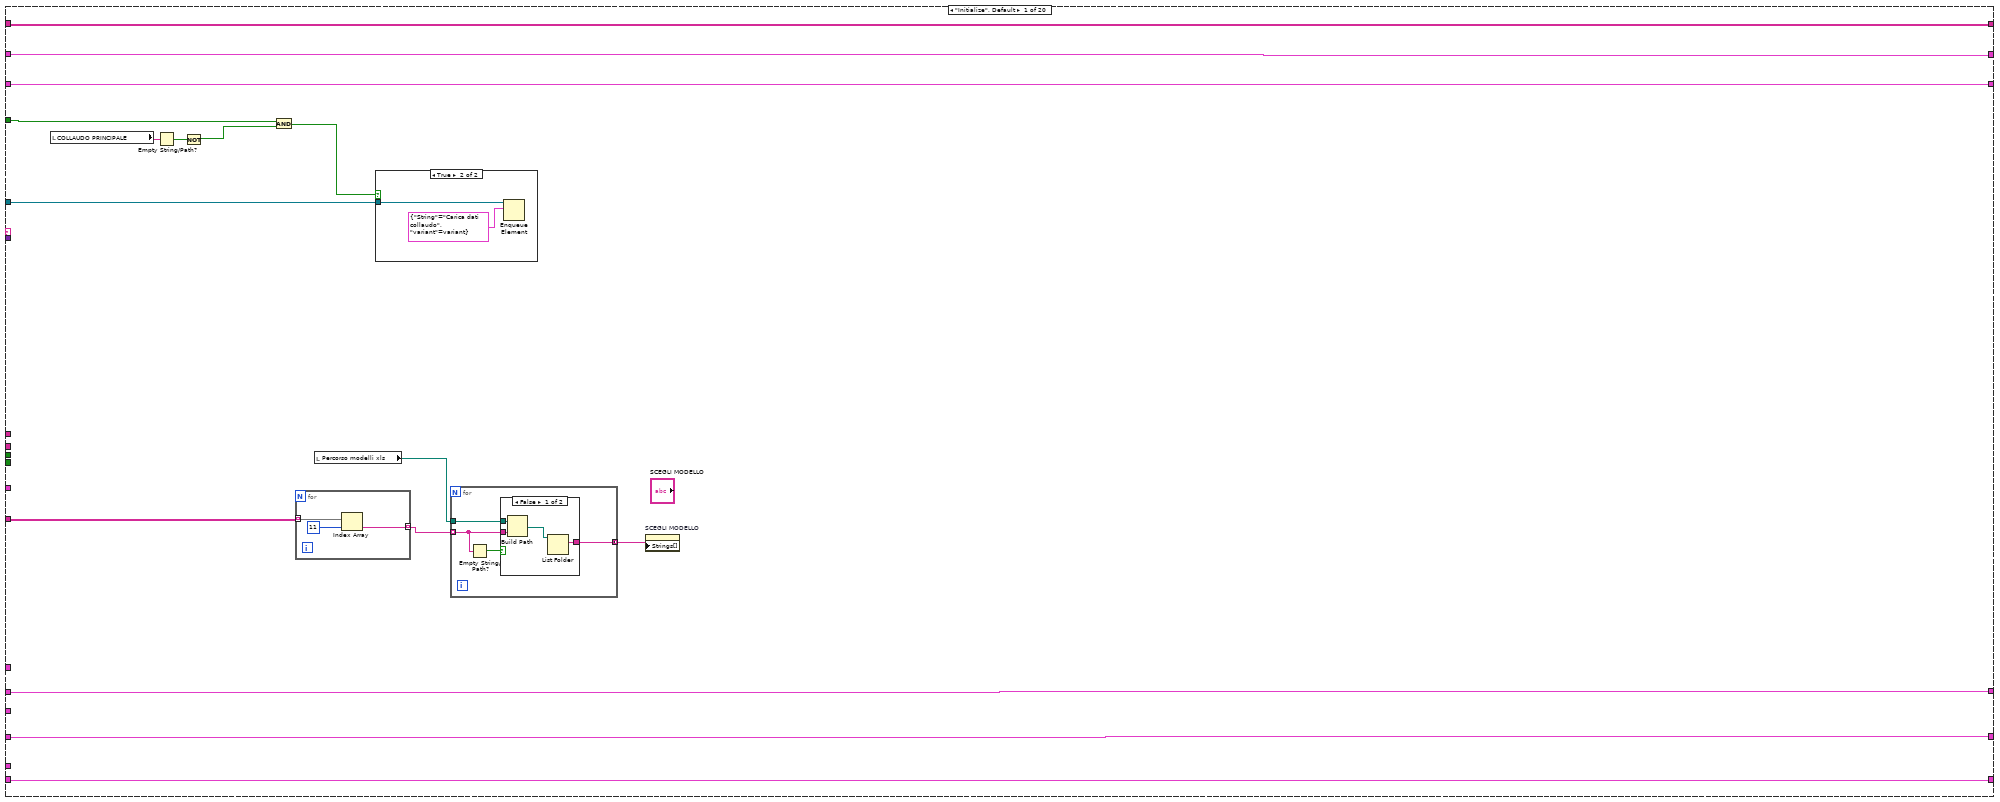
[diagram p5: hidden frame]
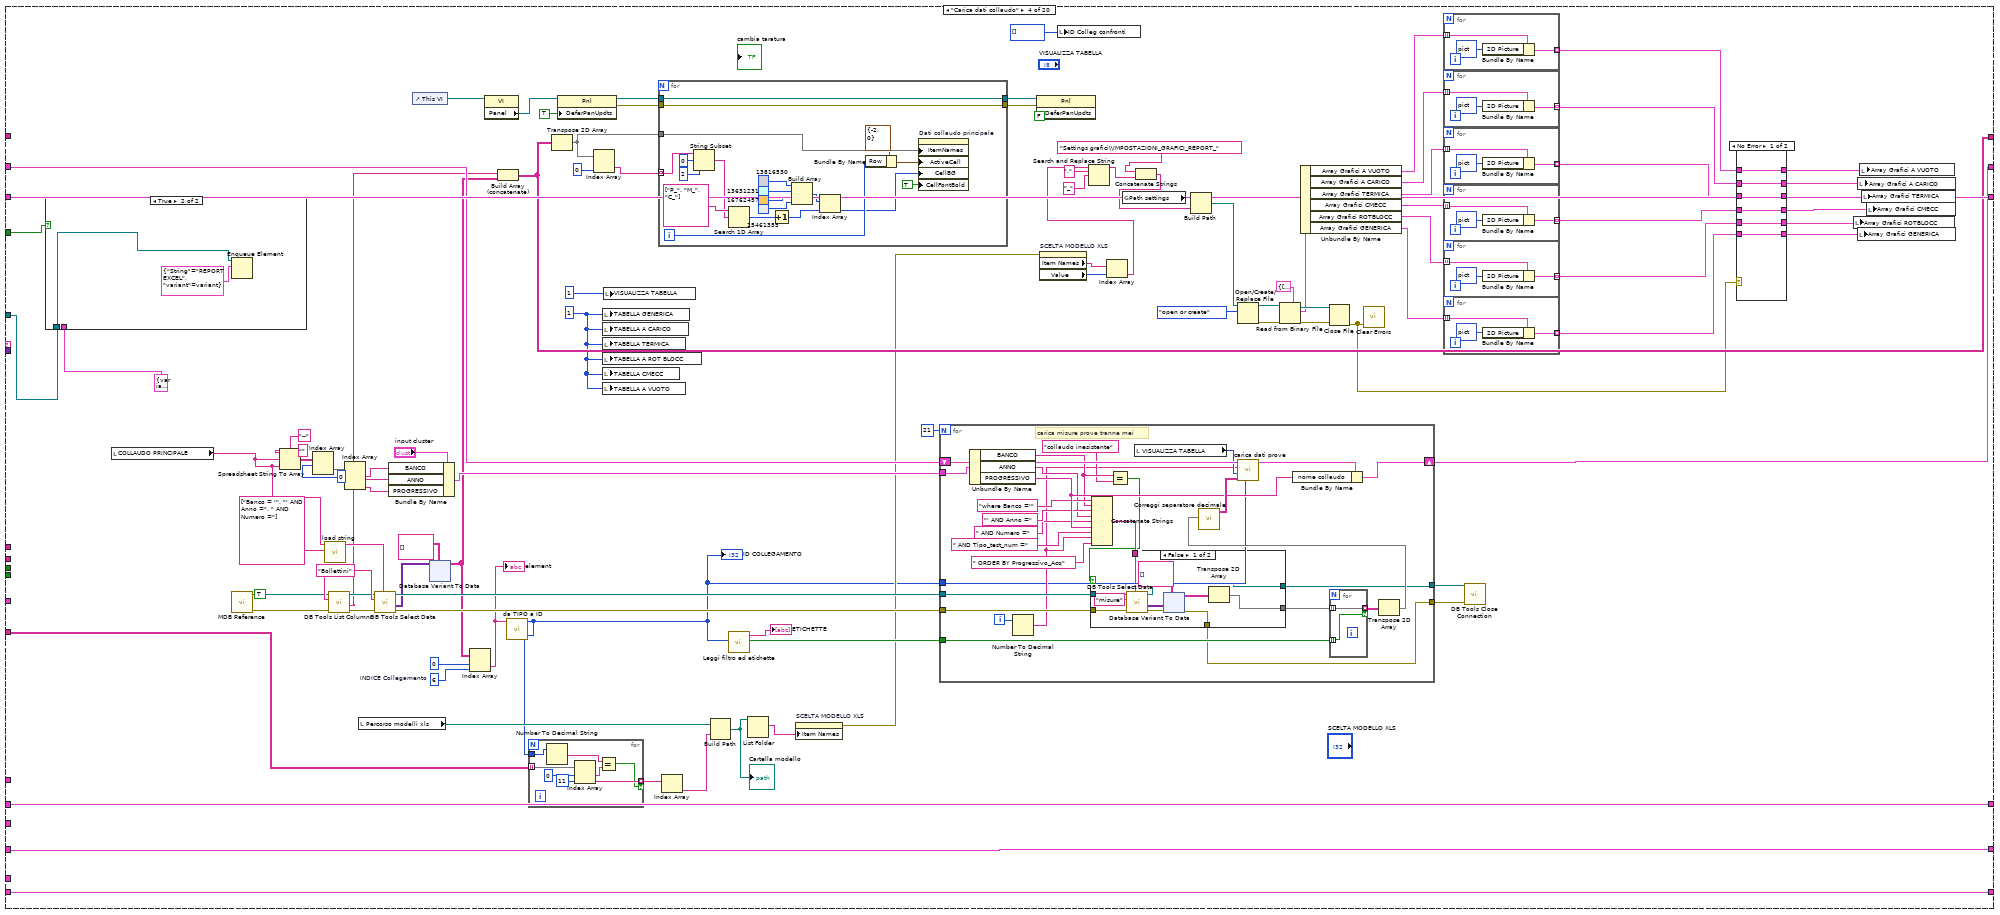
[diagram p10: hidden frame]
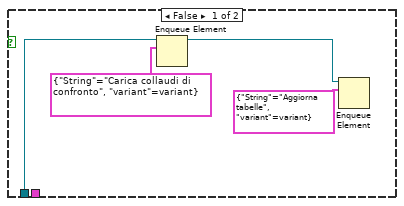
[diagram p11: hidden frame]
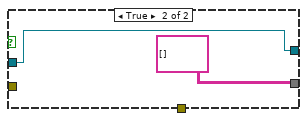
[diagram p13: hidden frame]
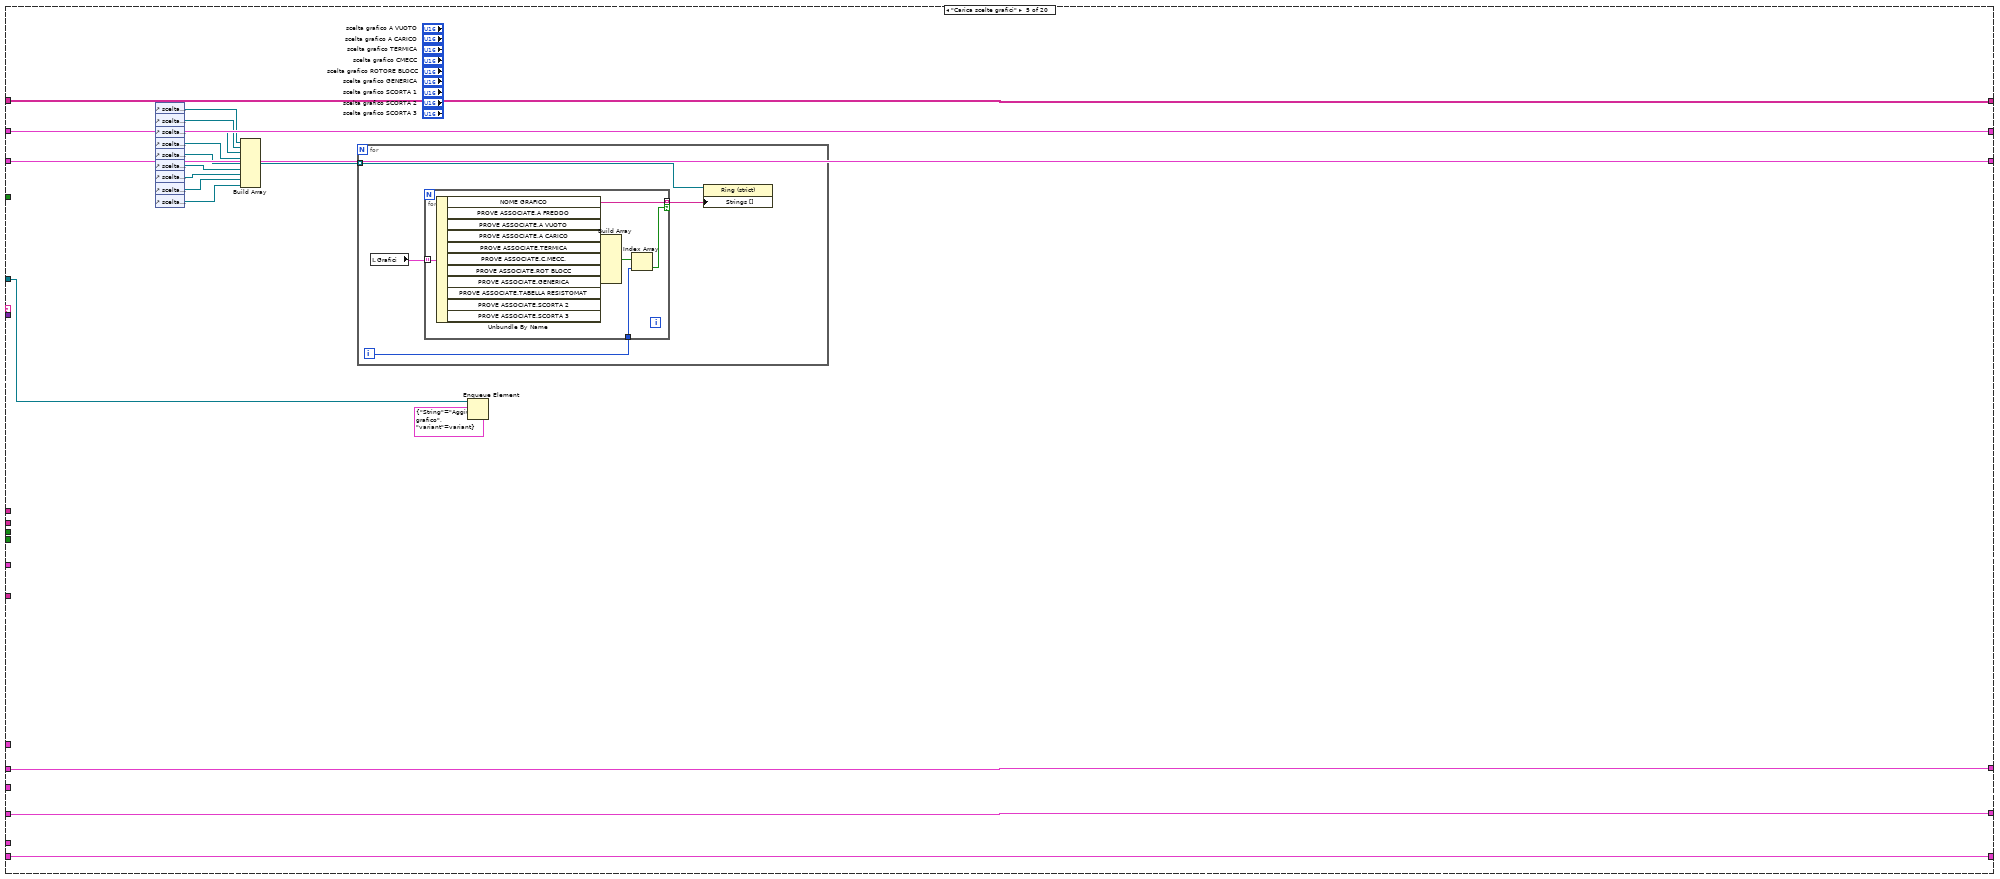
[diagram p14: hidden frame]
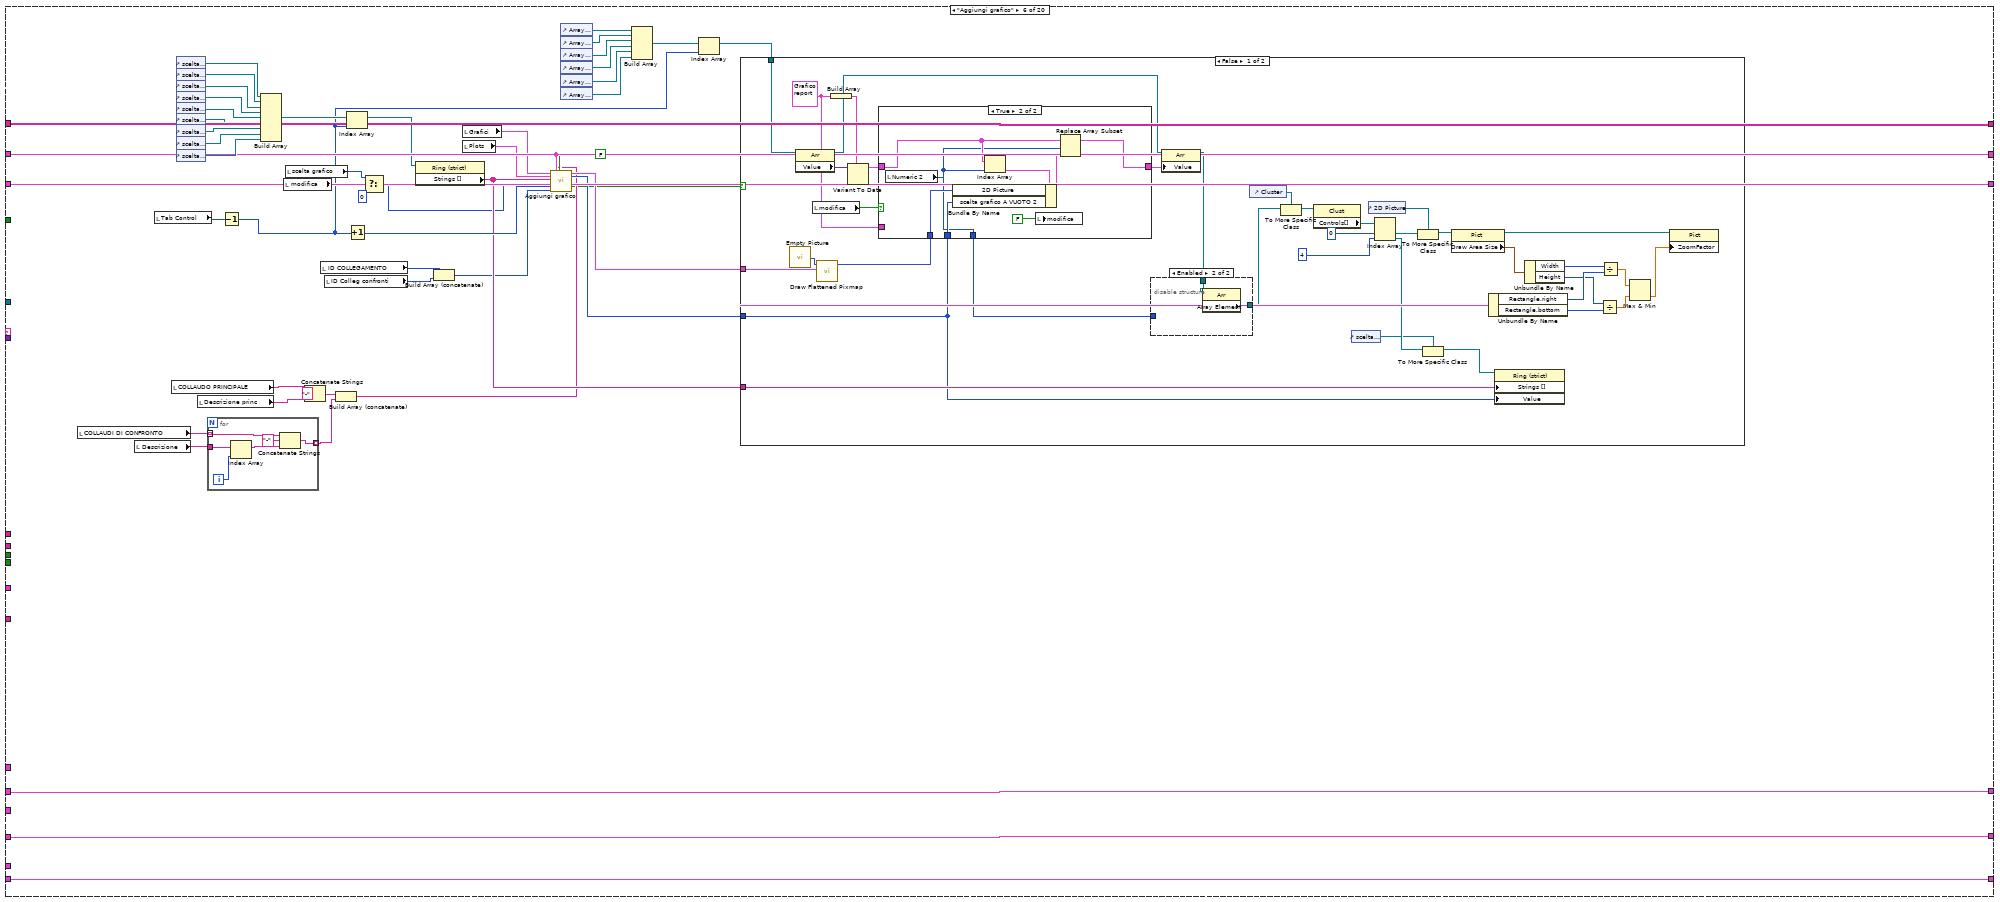
[diagram p15: hidden frame]
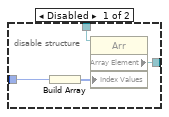
[diagram p16: hidden frame]
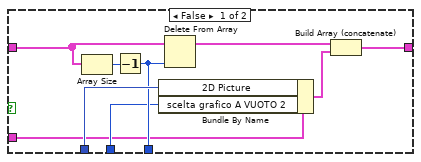
[diagram p17: hidden frame]
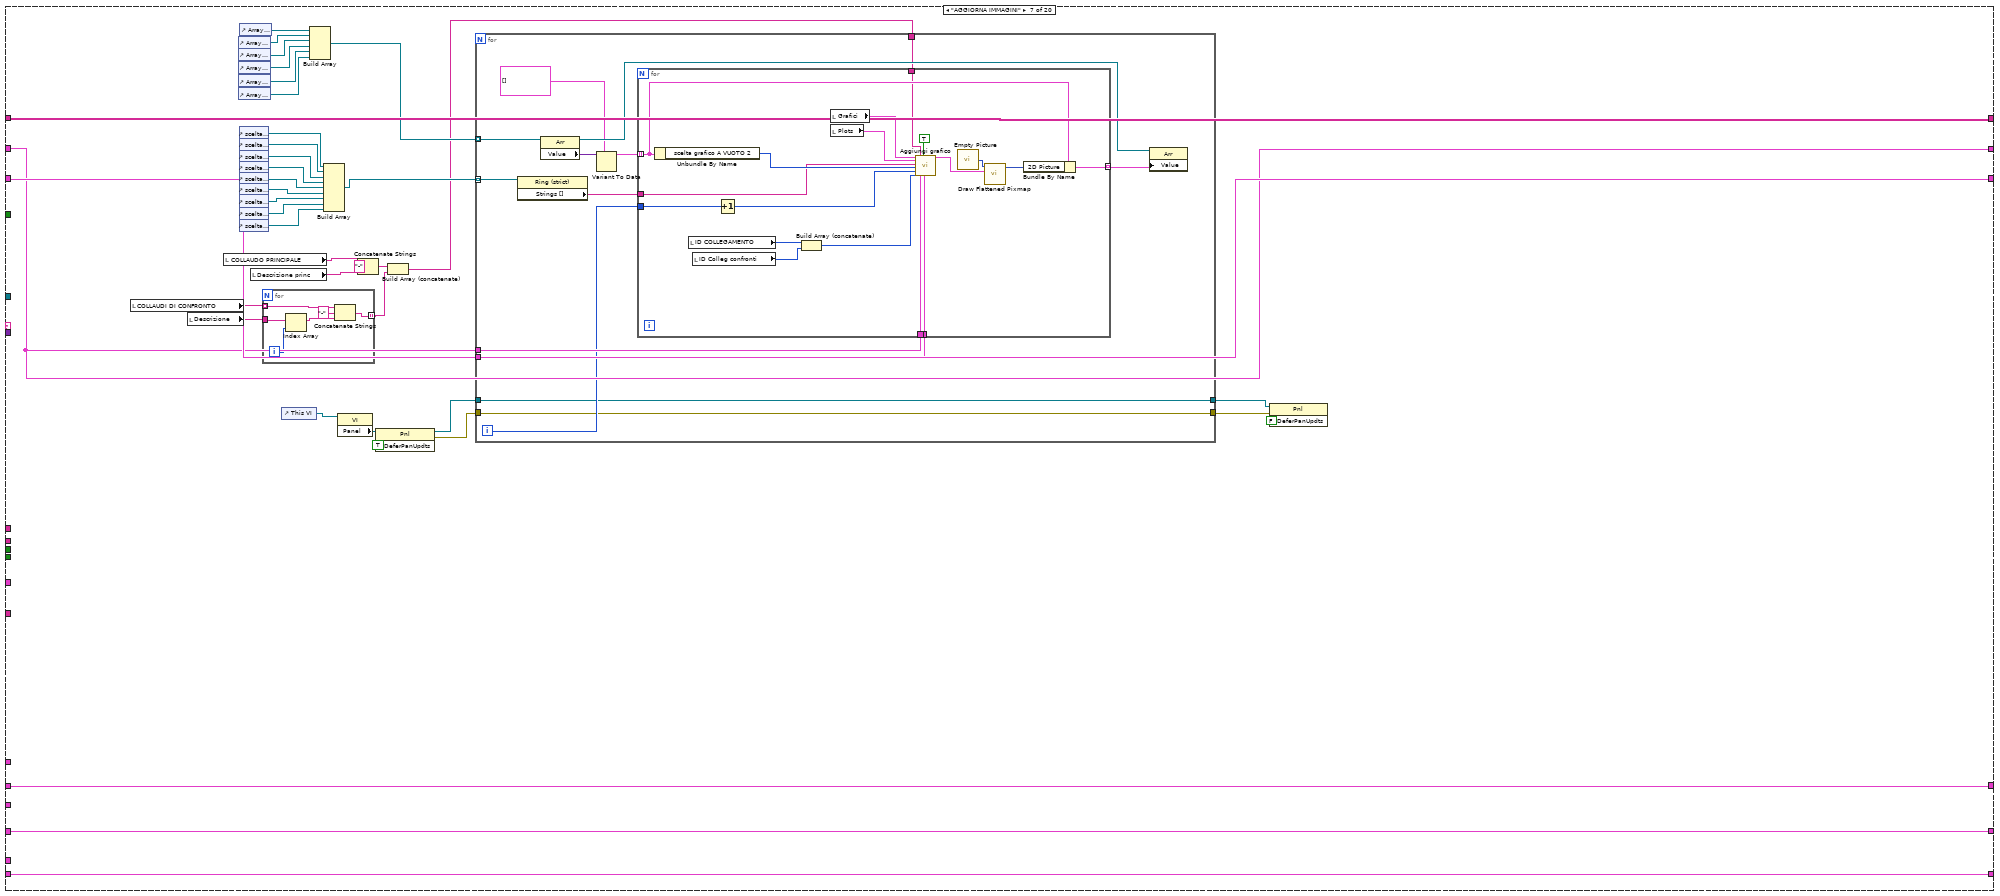
[diagram p19: hidden frame]
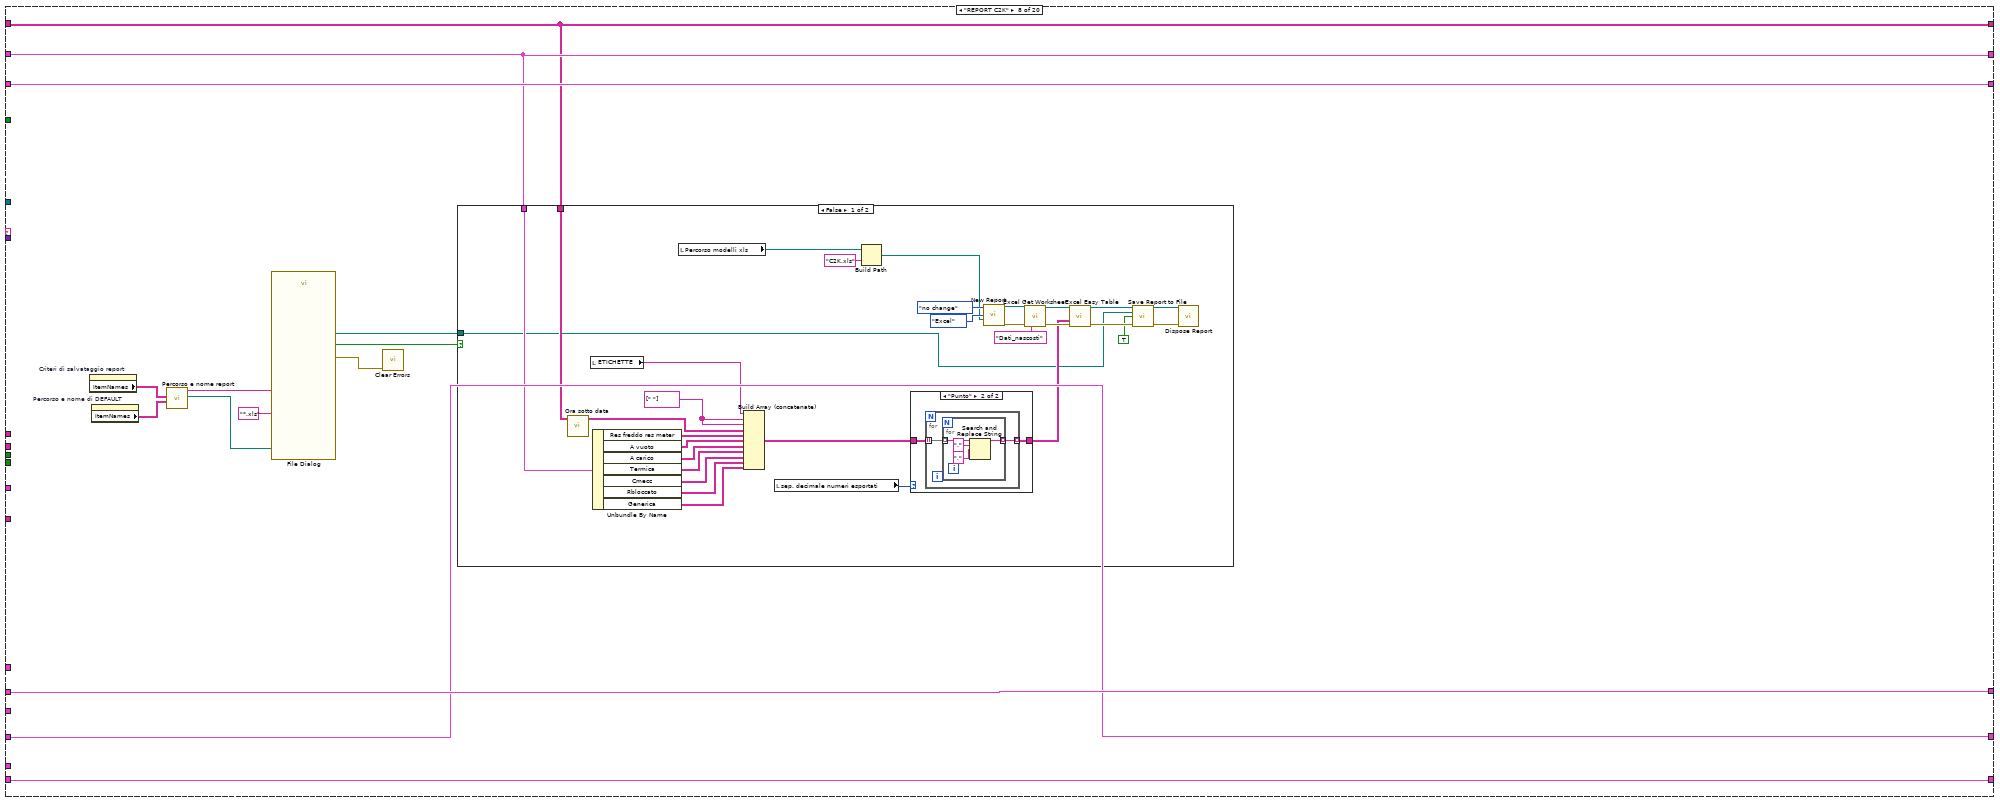
[diagram p20: hidden frame]
diagram:
  w1 = string[][] [] ("Item Names")
  w2 = T8[] [] ("Array Grafici TERMICA")
  w39 = string[][] [] ("Item Names")
  w42 = T15 {"NPSH-H"=[], "Q-NPSH"=[]}  # GRAFICI PROVA NPSH
  w51 = T16 {"DT"=[], "TC"=[]}  # GRAFICI PROVA TERMICA
  w72 = T17 {"QH"=[], "QRPM"=[], "QP2"=[]}  # GRAFICI PROVA QH
  n1 = local write "COLLAUDI DI CONFRONTO"(string[] [] ("COLLAUDI DI CONFRONTO")) -> ()
  n2 = local write "Array Grafici ROTBLOCC"(w2) -> ()
  n3 = local write "Array Grafici GENERICA"(w2) -> ()
  n4 = local write "Array Grafici A CARICO"(w2) -> ()
  n5 = local write "Array Grafici A VUOTO"(w2) -> ()
  n6 = local write "Array Grafici TERMICA"(w2) -> ()
  n7 = local write "Array Grafici CMECC"(w2) -> ()
  n8 = property on="Percorso e nome di DEFAULT" class="MCListbox (strict)"("ItemNames"=w39) -> ()  [unwired: 2 in, 2 out]
  n9 = property on="Criteri di salvataggio report" class="MCListbox (strict)"("ItemNames"=w39) -> ()  [unwired: 2 in, 2 out]
  n10 = property on="TABELLA A VUOTO" class="MCListbox (strict)"("ItemNames"=w1) -> ()  [unwired: 2 in, 2 out]
  n11 = property on="Res INIZIO prova VUOTO" class="MCListbox (strict)"("ItemNames"=w1) -> ()  [unwired: 2 in, 2 out]
  n12 = property on="Res FINE prova VUOTO" class="MCListbox (strict)"("ItemNames"=w1) -> ()  [unwired: 2 in, 2 out]
  n13 = property on="TABELLA A CARICO" class="MCListbox (strict)"("ItemNames"=w1) -> ()  [unwired: 2 in, 2 out]
  n14 = property on="Res INIZIO prova CARICO" class="MCListbox (strict)"("ItemNames"=w1) -> ()  [unwired: 2 in, 2 out]
  n15 = property on="Res FINE prova CARICO" class="MCListbox (strict)"("ItemNames"=w1) -> ()  [unwired: 2 in, 2 out]
  n16 = property on="TABELLA RES FREDDO RESISTOMAT" class="MCListbox (strict)"("ItemNames"=w1) -> ()  [unwired: 2 in, 2 out]
  n17 = property on="TABELLA TERMICA" class="MCListbox (strict)"("ItemNames"=w1) -> ()  [unwired: 2 in, 2 out]
  n18 = property on="TABELLA RES TERMICA" class="MCListbox (strict)"("ItemNames"=w1) -> ()  [unwired: 2 in, 2 out]
  n19 = property on="TABELLA EQ TERMICO" class="MCListbox (strict)"("ItemNames"=w1) -> ()  [unwired: 2 in, 2 out]
  n20 = property on="TABELLA C MECC" class="MCListbox (strict)"("ItemNames"=w1) -> ()  [unwired: 2 in, 2 out]
  n21 = property on="TABELLA COPPIA MAX" class="MCListbox (strict)"("ItemNames"=w1) -> ()  [unwired: 2 in, 2 out]
  n22 = property on="TABELLA ROT BLOCC" class="MCListbox (strict)"("ItemNames"=w1) -> ()  [unwired: 2 in, 2 out]
  n23 = property on="TABELLA I SPUNTO" class="MCListbox (strict)"("ItemNames"=w1) -> ()  [unwired: 2 in, 2 out]
  n24 = property on="TABELLA GENERICA" class="MCListbox (strict)"("ItemNames"=w1) -> ()  [unwired: 2 in, 2 out]
  n25 = call <vilib>:"Application Directory.vi"() -> ("Application Directory"=w61:path)
  n26 = Build Path(base path=w61, name or relative path="Settings\\Tolleranze croci.txt") -> (appended path=w59:path)
  n27 = call-poly <vilib>:"Read Delimited Spreadsheet.vi"("file path (dialog if empty)"=w59, "delimiter (\\t)"="::" ("delimiter (\\t)")) -> ("all rows"=w57:string[][])  [unwired: 8 in, 5 out]
  n28 = Index Array(array=w57, index (col)=1 ("disabled index (col)")) -> (element=w55:string[])  [unwired: 1 in]
  n29 = Index Array(array=w55) -> (element #1=w54:string, element #2=w53:string, element #3=w52:string)  [unwired: 7 in, 4 out]
  n30 = call "String To Dbl.vi"("String"=w54) -> ("Numeric"=w44:dbl)  [unwired: 10 in]
  n31 = call "String To Dbl.vi"("String"=w53) -> ("Numeric"=w45:dbl)  [unwired: 10 in]
  n32 = call "String To Dbl.vi"("String"=w52) -> ("Numeric"=w46:dbl)  [unwired: 10 in]
  n33 = local write "toll Q"(w44) -> ()
  n34 = local write "toll H"(w45) -> ()
  n35 = local write "toll P2"(w46) -> ()
  n36 = property on="REPORT EXCEL" class="Bool (strict)"("Visible"=TRUE) -> ()  [unwired: 2 in, 2 out]
  n37 = property on="SCELTA MODELLO XLS" class="LstBox (strict)"() -> ("Item Names"=w12:string[], "Value"=w11:i32)  [unwired: 2 in, 2 out]
  n38 = disable-structure shown="Disabled" {
    frame Disabled {
      n39 = call "Grafica all plots.vi"() -> ()  [unwired: 20 in]
    }
    frame Enabled {
    }
  }
  n40 = local write "Boolean"(FALSE ("Boolean")) -> ()
  n41 = Index Array(array=w12, index=w11) -> ()  [unwired: 1 out]
  n42 = call <vilib>:"Application Directory.vi"() -> ("Application Directory"=w38:path)
  n43 = Build Path(base path=w38, name or relative path="Settings\\Assistenza.txt") -> (appended path=w36:path)
  n44 = call-poly <vilib>:"Read From Spreadsheet File.vi"("delimiter (\\t)"="::" ("delimiter (\\t)"), "file path (dialog if empty)"=w36) -> ("all rows"=w35:string[][])  [unwired: 5 in, 4 out]
  n45 = control-ref of="This VI"() -> (w9:refnum<vi>)
  n46 = Index Array(array=w35, index (col)=1 ("disabled index (col)")) -> (element=w33:string[])  [unwired: 1 in]
  n47 = Index Array(array=w33) -> (element #11=w31:string)  [unwired: 11 in, 10 out]
  n48 = String To Path(string=w31) -> (path=w4:path)
  n49 = Initialize Array(cluster{"X":dbl[], "Y":dbl[]} {"X"=[], "Y"=[]} ("QP"), 100 ("dimension size")) -> (w41:cluster{"X":dbl[], "Y":dbl[]}[])
  n50 = case shown="False" "Report collaudo in corso?" {
    selector: "Report collaudo in corso?" -> [w82 _]
    tunnel: w9 -> [w85 _]
    frame False {
      n51 = Not(x=w82) -> (.not. x?=w84:bool)
      n52 = invoke class="VI" method="FP.Open"(reference=w85, "Activate"=w84, "State"=T18."Standard") -> ()  [unwired: 2 in, 5 out]
    }
    frame True {
    }
  }
  n53 = case shown="False" "Report collaudo in corso?" {
    frame False {
      n54 = local write "COLLAUDO PRINCIPALE"("" ("COLLAUDO PRINCIPALE")) -> ()
    }
    frame True {
    }
  }
  n55 = global write "Global percorso impostazioni.vi" "Path settings"(w4) -> ()
  n56 = Obtain Queue(name (unnamed)="Q_REPORT", element data type=cluster{"String":string, "variant":variant} {"String"="", "variant"=variant} ("element")) -> (queue out=w78:refnum<queue>, error out=w79:errorcluster)  [unwired: 3 in, 1 out]
  n57 = Flush Queue(queue=w78, error in (no error)=w79) -> (queue out=w80:refnum<queue>, error out=w81:errorcluster)  [unwired: 1 out]
  n58 = Build Path(base path=w4, name or relative path="Settings grafici\\plots") -> (appended path=w15:path)
  n59 = Build Path(base path=w4, name or relative path="Filtri\\filtri36m.txt") -> (appended path=w69:path)
  n60 = Build Path(base path=w4, name or relative path="Settings grafici\\grafici") -> (appended path=w14:path)
  n61 = Bundle By Name(cluster=w42, "NPSH-H"=w41, "Q-NPSH"=w41) -> (w40:T15)
  n62 = Bundle By Name(cluster=w72, "QH"=w41, "QRPM"=w41, "QP2"=w41) -> (w48:T17)
  n63 = Enqueue Element(queue=w80, element=cluster{"String":string, "variant":variant} {"String"="CARICA DEFAULT", "variant"=variant}, error in (no error)=w81) -> (queue out=w73:refnum<queue>, error out=w76:errorcluster)  [unwired: 1 in, 1 out]
  n64 = Bundle By Name(cluster=w51, "DT"=w41, "TC"=w41) -> (w47:T16)
  n65 = Build Path(base path=w4, name or relative path="Filtri\\TIPI_COLLEGAMENTO.txt") -> (appended path=w5:path)
  n66 = call "filtra etichette NM.vi"("File filtri path"=w69) -> ("indici grafici m,3,6"=w67:T19[], "Array 3ph3ch"=w63:string[], "Array 1ph"=w62:string[], "Filtro 3ph3ch"=w66:bool[], "Filtro 3ph6ch"=w65:bool[], "Filtro 1ph"=w64:bool[])  [unwired: 11 in, 2 out]
  n67 = Open/Create/Replace File(file path (use dialog)=w15, operation (0:open)=T14."open or create") -> (refnum out=w19:refnum<file>, error out=w18:errorcluster)  [unwired: 4 in, 1 out]
  n68 = Open/Create/Replace File(file path (use dialog)=w14, operation (0:open)=T14."open or create") -> (refnum out=w26:refnum<file>, error out=w27:errorcluster)  [unwired: 4 in, 1 out]
  n69 = Read from Binary File(5:T4[] [], 8:w18, 11:w19) -> (0:w28:errorcluster, 2:w16:T4[], 3:w29:refnum<file>)  [unwired: 3 in, 1 out]
  n70 = Read from Binary File(5:T5[] [{"ASSE X 1"={"NOME ASSE"="Time[s]", "AUTO\nSCALA?"=TRUE, "MIN"=0.0, "MAX"=0.0, "Colore asse"=16448250, "Griglie Maggiori"=0, "Griglie Minori"=0, "Decimali"=0}, "ASSE X 2"={"NOME ASSE"="", "AUTO\nSCALA?"=FALSE, "MIN"=0.0, "MAX"=0.0, "Colore asse"=16448250, "Griglie Maggiori"=0, "Griglie Minori"=0, "Decimali"=0}, "ASSE Y 1"={"NOME ASSE"="Voltage[V]", "AUTO\nSCALA?"=TRUE, "MIN"=0.0, "MAX"=0.0, "Colore asse"=16448250, "Griglie Maggiori"=0, "Griglie Minori"=0, "Decimali"=0}, "ASSE Y 2"={"NOME ASSE"="C[Nm]", "AUTO\nSCALA?"=FALSE, "MIN"=0.0, "MAX"=1.0, "Colore asse"=16448250, "Griglie Maggiori"=0, "Griglie Minori"=0, "Decimali"=0}, "ASSE Y 3"={"NOME ASSE"="Pot[kW]", "AUTO\nSCALA?"=FALSE, "MIN"=0.0, "MAX"=0.0, "Colore asse"=16448250, "Griglie Maggiori"=0, "Griglie Minori"=0, "Decimali"=0}, "ASSE Y 4"={"NOME ASSE"="eff[%]", "AUTO\nSCALA?"=FALSE, "MIN"=0.0, "MAX"=0.0, "Colore asse"=16448250, "Griglie Maggiori"=0, "Griglie Minori"=0, "Decimali"=0}, "X1"=TRUE, "X2"=FALSE, "Y1"=TRUE, "Y2"=FALSE, "Y3"=FALSE, "Y4"=FALSE, "NOME GRAFICO"="Voltage-Time", "PROVE ASSOCIATE"={"A FREDDO"=FALSE, "A VUOTO"=TRUE, "A CARICO"=FALSE, "TERMICA"=FALSE, "C.MECC."=FALSE, "ROT BLOCC"=FALSE, "GENERICA"=FALSE, "TABELLA RESISTOMAT"=FALSE, "SCORTA 2"=FALSE, "SCORTA 3"=FALSE}, "ASSE Y 5"={"NOME ASSE"="", "AUTO\nSCALA?"=FALSE, "MIN"=0.0, "MAX"=0.0, "Colore asse"=16448250, "Griglie Maggiori"=0, "Griglie Minori"=0, "Decimali"=0}, "Y5"=FALSE, "Colore sfondo grafico"=0}, {"ASSE X 1"={"NOME ASSE"="Voltage[V]", "AUTO\nSCALA?"=TRUE, "MIN"=0.0, "MAX"=0.0, "Colore asse"=16448250, "Griglie Maggiori"=0, "Griglie Minori"=0, "Decimali"=0}, "ASSE X 2"={"NOME ASSE"="", "AUTO\nSCALA?"=FALSE, "MIN"=0.0, "MAX"=0.0, "Colore asse"=16448250, "Griglie Maggiori"=0, "Griglie Minori"=0, "Decimali"=0}, "ASSE Y 1"={"NOME ASSE"="Current[A]", "AUTO\nSCALA?"=TRUE, "MIN"=0.0, "MAX"=0.0, "Colore asse"=16448250, "Griglie Maggiori"=0, "Griglie Minori"=0, "Decimali"=0}, "ASSE Y 2"={"NOME ASSE"="CosFi", "AUTO\nSCALA?"=FALSE, "MIN"=0.0, "MAX"=1.0, "Colore asse"=16860, "Griglie Maggiori"=0, "Griglie Minori"=0, "Decimali"=0}, "ASSE Y 3"={"NOME ASSE"="Pot[kW]", "AUTO\nSCALA?"=FALSE, "MIN"=0.0, "MAX"=0.0, "Colore asse"=16448250, "Griglie Maggiori"=0, "Griglie Minori"=0, "Decimali"=0}, "ASSE Y 4"={"NOME ASSE"="eff[%]", "AUTO\nSCALA?"=FALSE, "MIN"=0.0, "MAX"=0.0, "Colore asse"=16448250, "Griglie Maggiori"=0, "Griglie Minori"=0, "Decimali"=0}, "X1"=TRUE, "X2"=FALSE, "Y1"=TRUE, "Y2"=TRUE, "Y3"=FALSE, "Y4"=FALSE, "NOME GRAFICO"="I[A]-CosFi-Voltage", "PROVE ASSOCIATE"={"A FREDDO"=FALSE, "A VUOTO"=TRUE, "A CARICO"=FALSE, "TERMICA"=FALSE, "C.MECC."=FALSE, "ROT BLOCC"=FALSE, "GENERICA"=FALSE, "TABELLA RESISTOMAT"=FALSE, "SCORTA 2"=FALSE, "SCORTA 3"=FALSE}, "ASSE Y 5"={"NOME ASSE"="", "AUTO\nSCALA?"=FALSE, "MIN"=0.0, "MAX"=0.0, "Colore asse"=16448250, "Griglie Maggiori"=0, "Griglie Minori"=0, "Decimali"=0}, "Y5"=FALSE, "Colore sfondo grafico"=0}, {"ASSE X 1"={"NOME ASSE"="RPM", "AUTO\nSCALA?"=TRUE, "MIN"=0.0, "MAX"=0.0, "Colore asse"=16448250, "Griglie Maggiori"=0, "Griglie Minori"=0, "Decimali"=0}, "ASSE X 2"={"NOME ASSE"="", "AUTO\nSCALA?"=FALSE, "MIN"=0.0, "MAX"=0.0, "Colore asse"=0, "Griglie Maggiori"=0, "Griglie Minori"=0, "Decimali"=0}, "ASSE Y 1"={"NOME ASSE"="Coppia[Nm]", "AUTO\nSCALA?"=TRUE, "MIN"=0.0, "MAX"=0.0, "Colore asse"=16448250, "Griglie Maggiori"=0, "Griglie Minori"=0, "Decimali"=0}, "ASSE Y 2"={"NOME ASSE"="", "AUTO\nSCALA?"=FALSE, "MIN"=0.0, "MAX"=0.0, "Colore asse"=0, "Griglie Maggiori"=0, "Griglie Minori"=0, "Decimali"=0}, "ASSE Y 3"={"NOME ASSE"="", "AUTO\nSCALA?"=FALSE, "MIN"=0.0, "MAX"=0.0, "Colore asse"=0, "Griglie Maggiori"=0, "Griglie Minori"=0, "Decimali"=0}, "ASSE Y 4"={"NOME ASSE"="", "AUTO\nSCALA?"=FALSE, "MIN"=0.0, "MAX"=0.0, "Colore asse"=0, "Griglie Maggiori"=0, "Griglie Minori"=0, "Decimali"=0}, "X1"=TRUE, "X2"=FALSE, "Y1"=TRUE, "Y2"=FALSE, "Y3"=FALSE, "Y4"=FALSE, "NOME GRAFICO"="C-RPM", "PROVE ASSOCIATE"={"A FREDDO"=FALSE, "A VUOTO"=FALSE, "A CARICO"=FALSE, "TERMICA"=FALSE, "C.MECC."=TRUE, "ROT BLOCC"=FALSE, "GENERICA"=FALSE, "TABELLA RESISTOMAT"=FALSE, "SCORTA 2"=FALSE, "SCORTA 3"=FALSE}, "ASSE Y 5"={"NOME ASSE"="", "AUTO\nSCALA?"=FALSE, "MIN"=0.0, "MAX"=0.0, "Colore asse"=0, "Griglie Maggiori"=0, "Griglie Minori"=0, "Decimali"=0}, "Y5"=FALSE, "Colore sfondo grafico"=0}, {"ASSE X 1"={"NOME ASSE"="RPM", "AUTO\nSCALA?"=TRUE, "MIN"=0.0, "MAX"=0.0, "Colore asse"=16448250, "Griglie Maggiori"=0, "Griglie Minori"=0, "Decimali"=0}, "ASSE X 2"={"NOME ASSE"="", "AUTO\nSCALA?"=FALSE, "MIN"=0.0, "MAX"=0.0, "Colore asse"=0, "Griglie Maggiori"=0, "Griglie Minori"=0, "Decimali"=0}, "ASSE Y 1"={"NOME ASSE"="Coppia[Nm]", "AUTO\nSCALA?"=TRUE, "MIN"=0.0, "MAX"=0.0, "Colore asse"=16448250, "Griglie Maggiori"=0, "Griglie Minori"=0, "Decimali"=0}, "ASSE Y 2"={"NOME ASSE"="Corrente[A]", "AUTO\nSCALA?"=TRUE, "MIN"=0.0, "MAX"=0.0, "Colore asse"=16711680, "Griglie Maggiori"=0, "Griglie Minori"=0, "Decimali"=0}, "ASSE Y 3"={"NOME ASSE"="Potenza[kW]", "AUTO\nSCALA?"=TRUE, "MIN"=0.0, "MAX"=0.0, "Colore asse"=6618880, "Griglie Maggiori"=0, "Griglie Minori"=0, "Decimali"=0}, "ASSE Y 4"={"NOME ASSE"="eff[%]", "AUTO\nSCALA?"=TRUE, "MIN"=0.0, "MAX"=0.0, "Colore asse"=9567230, "Griglie Maggiori"=0, "Griglie Minori"=0, "Decimali"=0}, "X1"=TRUE, "X2"=FALSE, "Y1"=TRUE, "Y2"=TRUE, "Y3"=TRUE, "Y4"=TRUE, "NOME GRAFICO"="Cmecc", "PROVE ASSOCIATE"={"A FREDDO"=FALSE, "A VUOTO"=FALSE, "A CARICO"=FALSE, "TERMICA"=FALSE, "C.MECC."=TRUE, "ROT BLOCC"=FALSE, "GENERICA"=FALSE, "TABELLA RESISTOMAT"=FALSE, "SCORTA 2"=FALSE, "SCORTA 3"=FALSE}, "ASSE Y 5"={"NOME ASSE"="", "AUTO\nSCALA?"=FALSE, "MIN"=0.0, "MAX"=0.0, "Colore asse"=0, "Griglie Maggiori"=0, "Griglie Minori"=0, "Decimali"=0}, "Y5"=FALSE, "Colore sfondo grafico"=0}, {"ASSE X 1"={"NOME ASSE"="Tempo[s]", "AUTO\nSCALA?"=TRUE, "MIN"=0.0, "MAX"=0.0, "Colore asse"=16448250, "Griglie Maggiori"=0, "Griglie Minori"=0, "Decimali"=0}, "ASSE X 2"={"NOME ASSE"="", "AUTO\nSCALA?"=FALSE, "MIN"=0.0, "MAX"=0.0, "Colore asse"=0, "Griglie Maggiori"=0, "Griglie Minori"=0, "Decimali"=0}, "ASSE Y 1"={"NOME ASSE"="Temperatura[°C]", "AUTO\nSCALA?"=TRUE, "MIN"=0.0, "MAX"=0.0, "Colore asse"=16448250, "Griglie Maggiori"=0, "Griglie Minori"=0, "Decimali"=0}, "ASSE Y 2"={"NOME ASSE"="Corrente[A]", "AUTO\nSCALA?"=TRUE, "MIN"=0.0, "MAX"=0.0, "Colore asse"=16711680, "Griglie Maggiori"=0, "Griglie Minori"=0, "Decimali"=0}, "ASSE Y 3"={"NOME ASSE"="Potenza[kW]", "AUTO\nSCALA?"=TRUE, "MIN"=0.0, "MAX"=0.0, "Colore asse"=6618880, "Griglie Maggiori"=0, "Griglie Minori"=0, "Decimali"=0}, "ASSE Y 4"={"NOME ASSE"="eff[%]", "AUTO\nSCALA?"=TRUE, "MIN"=0.0, "MAX"=0.0, "Colore asse"=9567230, "Griglie Maggiori"=0, "Griglie Minori"=0, "Decimali"=0}, "X1"=TRUE, "X2"=FALSE, "Y1"=TRUE, "Y2"=FALSE, "Y3"=FALSE, "Y4"=FALSE, "NOME GRAFICO"="Temperature", "PROVE ASSOCIATE"={"A FREDDO"=FALSE, "A VUOTO"=FALSE, "A CARICO"=FALSE, "TERMICA"=TRUE, "C.MECC."=FALSE, "ROT BLOCC"=FALSE, "GENERICA"=FALSE, "TABELLA RESISTOMAT"=FALSE, "SCORTA 2"=FALSE, "SCORTA 3"=FALSE}, "ASSE Y 5"={"NOME ASSE"="", "AUTO\nSCALA?"=FALSE, "MIN"=0.0, "MAX"=0.0, "Colore asse"=0, "Griglie Maggiori"=0, "Griglie Minori"=0, "Decimali"=0}, "Y5"=FALSE, "Colore sfondo grafico"=0}, {"ASSE X 1"={"NOME ASSE"="Tempo[s]", "AUTO\nSCALA?"=TRUE, "MIN"=0.0, "MAX"=0.0, "Colore asse"=16448250, "Griglie Maggiori"=0, "Griglie Minori"=0, "Decimali"=0}, "ASSE X 2"={"NOME ASSE"="", "AUTO\nSCALA?"=FALSE, "MIN"=0.0, "MAX"=0.0, "Colore asse"=0, "Griglie Maggiori"=0, "Griglie Minori"=0, "Decimali"=0}, "ASSE Y 1"={"NOME ASSE"="Potenza[W]", "AUTO\nSCALA?"=TRUE, "MIN"=0.0, "MAX"=0.0, "Colore asse"=16448250, "Griglie Maggiori"=0, "Griglie Minori"=0, "Decimali"=0}, "ASSE Y 2"={"NOME ASSE"="Corrente[A]", "AUTO\nSCALA?"=TRUE, "MIN"=0.0, "MAX"=0.0, "Colore asse"=16711680, "Griglie Maggiori"=0, "Griglie Minori"=0, "Decimali"=0}, "ASSE Y 3"={"NOME ASSE"="Potenza[kW]", "AUTO\nSCALA?"=TRUE, "MIN"=0.0, "MAX"=0.0, "Colore asse"=6618880, "Griglie Maggiori"=0, "Griglie Minori"=0, "Decimali"=0}, "ASSE Y 4"={"NOME ASSE"="eff[%]", "AUTO\nSCALA?"=TRUE, "MIN"=0.0, "MAX"=0.0, "Colore asse"=9567230, "Griglie Maggiori"=0, "Griglie Minori"=0, "Decimali"=0}, "X1"=TRUE, "X2"=FALSE, "Y1"=TRUE, "Y2"=TRUE, "Y3"=FALSE, "Y4"=FALSE, "NOME GRAFICO"="Power-Time", "PROVE ASSOCIATE"={"A FREDDO"=FALSE, "A VUOTO"=FALSE, "A CARICO"=TRUE, "TERMICA"=TRUE, "C.MECC."=FALSE, "ROT BLOCC"=FALSE, "GENERICA"=FALSE, "TABELLA RESISTOMAT"=FALSE, "SCORTA 2"=FALSE, "SCORTA 3"=FALSE}, "ASSE Y 5"={"NOME ASSE"="", "AUTO\nSCALA?"=FALSE, "MIN"=0.0, "MAX"=0.0, "Colore asse"=0, "Griglie Maggiori"=0, "Griglie Minori"=0, "Decimali"=0}, "Y5"=FALSE, "Colore sfondo grafico"=0}] ("Grafici"), 8:w27, 11:w26) -> (0:w24:errorcluster, 2:w17:T5[], 3:w23:refnum<file>)  [unwired: 3 in, 1 out]
  n71 = call-poly <vilib>:"Read Delimited Spreadsheet.vi"("file path (dialog if empty)"=w5, "delimiter (\\t)"="::") -> ("all rows"=w3:string[][])  [unwired: 8 in, 5 out]
  n72 = local write "Plots"(w16) -> ()
  n73 = Close File(refnum=w29, error in=w28) -> ()  [unwired: 2 out]
  n74 = local write "Grafici"(w17) -> ()
  n75 = Close File(refnum=w23, error in=w24) -> ()  [unwired: 2 out]
  n76 = while {
    tunnel: w73 -> [w90]
    tunnel: "banco" -> [w88]
    stop <- w89 stop-if-true
    n77 = event shown="[20] \"Modifica percorso default\": Value Change" {
      selector: _ -> [_ _ _ _ _ _ _ _ _ _ _ _ _ _ _ _ _ _ _ _ _ _]
      dyn-events: _ -> [_ _ _ _ _ _ _ _ _ _ _ _ _ _ _ _ _ _ _ _ _ _]
      timeout: 100 -> [_ _ _ _ _ _ _ _ _ _ _ _ _ _ _ _ _ _ _ _ _ _]
      tunnel: w90 -> [_ w101 w103 w111 w113 w116 w130 _ _ w200 w202 _ w223 _ w245 w249 w255 _ _ _ _ w321]
      tunnel: [_ _ _ _ _ _ _ _ _ _ _ _ _ _ _ _ _ _ _ _ _ TRUE] -> w89
      tunnel: w88 -> [_ _ _ _ _ _ _ _ _ _ _ w204 _ w228 _ _ _ _ _ _ _ _]
      event Timeout {
        n78 = event-data() -> ()  [unwired: 1 in, 3 out]
        n79 = property on="SCELTA MODELLO XLS" class="LstBox (strict)"() -> ("Item Names"=w95:string[], "Value"=w94:i32)  [unwired: 2 in, 2 out]
        n80 = Index Array(array=w95, index=w94) -> (element=w98:string)
        n81 = Search and Replace String(input string=w98, search string="GESTIONALE") -> (number of replacements=w97:i32)  [unwired: 6 in, 3 out]
        n82 = Greater Than 0?(x=w97) -> (x > 0?=w91:bool)
        "Tipo report" <- w91
        n83 = feedback-in #1(w91) -> ()
        n84 = feedback #1() -> (w93:bool)  [unwired: 1 in]
        n85 = Not Equal?(x=w91, y=w93) -> (x != y?=w92:bool)
        n86 = case shown="True" w92 {
          tunnel: w91 -> [_ w100]
          frame False {
          }
          frame True {
            n87 = Not(x=w100) -> (.not. x?=w99:bool)
            n88 = local write "EXCEL"(w99) -> ()
            n89 = local write "PDF"(w100) -> ()
          }
        }
      }
      event "carica collaudo in corso": Value Change {
        n90 = event-data() -> ()  [unwired: 1 in, 6 out]
        n91 = Enqueue Element(queue=w101, element=cluster{"String":string, "variant":variant} {"String"="Carica collaudo in corso", "variant"=variant}) -> ()  [unwired: 2 in, 3 out]
      }
      event "carica collaudi di confronto": Value Change {
        n92 = event-data() -> ()  [unwired: 1 in, 6 out]
        n93 = Enqueue Element(queue=w103, element=cluster{"String":string, "variant":variant} {"String"="Carica collaudi di confronto", "variant"=variant}) -> ()  [unwired: 2 in, 3 out]
      }
      event "GRAFICA": Value Change {
        w110 = cluster{"String":string, "variant":variant} {"String"="Carica grafici", "variant"=variant} ("element")
        n94 = event-data() -> ()  [unwired: 1 in, 6 out]
        n95 = local read "tipo prova"() -> (w108:string)
        n96 = Unbundle By Name(w110) -> ("String"=w109:string)
        n97 = Concatenate Strings(w109, " " ("string"), w108) -> (w107:string)
        n98 = Bundle By Name(cluster=w110, "String"=w107) -> (w106:cluster{"String":string, "variant":variant})
        n99 = Enqueue Element(queue=w111, element=w106) -> ()  [unwired: 2 in, 3 out]
      }
      event "TABELLA A CARICO", "TABELLA A CARICO", "TABELLA A ROT BLOCC", "TABELLA CMECC", "TABELLA GENERICA", "TABELLA TERMICA", "TABELLA A VUOTO": Value Change {
        n100 = event-data() -> ()  [unwired: 1 in, 6 out]
        n101 = local write "CARICA COLLAUDI"(FALSE ("CARICA COLLAUDI")) -> ()
        n102 = Enqueue Element(queue=w113, element=cluster{"String":string, "variant":variant} {"String"="Aggiorna tabelle", "variant"=variant}) -> ()  [unwired: 2 in, 3 out]
      }
      event "CARICA COLLAUDI": Value Change {
        n103 = event-data() -> ()  [unwired: 1 in, 6 out]
        n104 = local write "CARICA COLLAUDI"(FALSE ("CARICA COLLAUDI")) -> ()
        n105 = Enqueue Element(queue=w116, element=cluster{"String":string, "variant":variant} {"String"="Carica dati collaudo", "variant"=variant}) -> ()  [unwired: 2 in, 3 out]
      }
      event "Array Grafici A VUOTO", "Array Grafici A CARICO", "Array Grafici TERMICA", "Array Grafici CMECC", "Array Grafici ROTBLOCC", "Array Grafici GENERICA": Value Change {
        n106 = event-data() -> ("CtlRef"=w128:refnum<vi>, "OldVal"=w118:T8[], "NewVal"=w119:T8[])  [unwired: 1 in, 3 out]
        n107 = Array Size(array=w118) -> (size(s)=w120:i32)
        n108 = Array Size(array=w119) -> (size(s)=w121:i32)
        n109 = for {
          tunnel: w119 -> [w151] mode=indexing
          tunnel: [w148] -> w127
          tunnel: [w146] -> w129
          tunnel: [w145] -> w126
          i -> [w148]
          stop <- w149 stop-if-true
          n110 = Unbundle By Name(w151) -> ("Aggiungi grafico"=w145:bool, "Settings grafico"=w150:bool, "Elimina grafico"=w146:bool, "scelta grafico A VUOTO 2"=→"scelta grafico":u16)
          n111 = Build Array(w145, w150, w146) -> (w147:bool[])
          n112 = Or Array Elements(Boolean array=w147) -> (logical OR=w149:bool)
        }
        "Numeric 2" <- w127
        n113 = Equal?(x=w120, y=w121) -> (x = y?=→"modifica":bool)
        n114 = case shown="True" w126 {
          tunnel: w130 -> [_ w143]
          frame False {
          }
          frame True {
            n115 = Enqueue Element(queue=w143, element=cluster{"String":string, "variant":variant} {"String"="Carica scelte grafici", "variant"=variant}) -> ()  [unwired: 2 in, 3 out]
          }
        }
        n116 = case shown="True" w129 {
          tunnel: w119 -> [w134 w141]
          tunnel: w128 -> [w135 w140]
          tunnel: w127 -> [_ w139]
          tunnel: [w135 w137] -> w123
          tunnel: [w134 w136] -> w125
          frame False {
          }
          frame True {
            n117 = Delete From Array(array=w141, length=1, index=w139) -> (array with subset deleted=w136:T8[])  [unwired: 1 out]
            n118 = property class="Arr"(reference=w140, "Value"=w136) -> (reference out=w137:refnum<vi>)  [unwired: 1 in, 1 out]
          }
        }
        n119 = for {
          tunnel: w125 -> [w133] mode=indexing
          tunnel: [w131] -> w124 mode=indexing
          w132 = FALSE ("Aggiungi grafico")
          n120 = Bundle By Name(cluster=w133, "Aggiungi grafico"=w132, "Settings grafico"=w132, "Elimina grafico"=w132) -> (w131:T8)
        }
        n121 = property class="Arr"(reference=w123, "Value"=w124) -> ()  [unwired: 1 in, 2 out]
      }
      event "salva impostazioni grafici": Value Change {
        n122 = event-data() -> ()  [unwired: 1 in, 6 out]
        n123 = property on="SCELTA MODELLO XLS" class="LstBox (strict)"() -> ("Item Names"=w158:string[], "Value"=w157:i32)  [unwired: 2 in, 2 out]
        n124 = Index Array(array=w158, index=w157) -> (element=w152:string)
        n125 = Concatenate Strings("Salvare la configurazione dei\ngrafici per il modello \"" ("string"), w152, "\" ?" ("string")) -> (w154:string)
        n126 = Two Button Dialog(message=w154) -> (T button?=w153:bool)  [unwired: 2 in]
        n127 = case shown="True" w153 {
          tunnel: w152 -> [_ w163]
          frame False {
          }
          frame True {
            n128 = Search and Replace String(input string=w163, search string=".", replace string="_" ("replace string (\"\")")) -> (result string=w160:string)  [unwired: 5 in, 3 out]
            n129 = global read "Global percorso impostazioni.vi" "Path settings"() -> (w177:path)
            n130 = Concatenate Strings("Settings grafici\\IMPOSTAZIONI_GRAFICI_REPORT_" ("name or relative path"), w160) -> (w164:string)
            n131 = Build Path(base path=w177, name or relative path=w164) -> (appended path=w178:path)
            n132 = Open/Create/Replace File(file path (use dialog)=w178, operation (0:open)=T14."replace or create with confirmation") -> (refnum out=w170:refnum<file>, error out=w168:errorcluster)  [unwired: 4 in, 1 out]
            n133 = local read "Array Grafici ROTBLOCC"() -> (w172:T8[])
            n134 = local read "Array Grafici GENERICA"() -> (w171:T8[])
            n135 = local read "Array Grafici A CARICO"() -> (w175:T8[])
            n136 = local read "Array Grafici A VUOTO"() -> (w176:T8[])
            n137 = local read "Array Grafici TERMICA"() -> (w174:T8[])
            n138 = local read "Array Grafici CMECC"() -> (w173:T8[])
            n139 = Bundle("Array Grafici A VUOTO"=w176, "Array Grafici A CARICO"=w175, "Array Grafici TERMICA"=w174, "Array Grafici CMECC"=w173, "Array Grafici ROTBLOCC"=w172, "Array Grafici GENERICA"=w171) -> (w169:T21)  [unwired: 1 in]
            n140 = Write to Binary File(file (use dialog)=w170, data=w169, error in=w168) -> (refnum out=w166:refnum<file>, error out=w167:errorcluster)  [unwired: 3 in, 1 out]
            n141 = Close File(refnum=w166, error in=w167) -> ()  [unwired: 2 out]
          }
        }
        n142 = local write "salva impostazioni grafici"(FALSE ("salva impostazioni grafici")) -> ()
      }
      event "IMPOSTAZIONI GRAFICI": Value Change {
        n143 = event-data() -> ()  [unwired: 1 in, 6 out]
        n144 = flat-sequence {
          frame #0 {
            n145 = disable-structure shown="Enabled" {
              frame Disabled {
                n146 = call "Grafici MANAGER REPORT.vi"() -> ()  [unwired: 12 in]
              }
              frame Enabled {
                n147 = call "Grafici MANAGER.vi"() -> ()  [unwired: 12 in]
              }
            }
          }
          frame #1 {
            n148 = global read "Global percorso impostazioni.vi" "Path settings"() -> (w190:path)
            n149 = global read "Global percorso impostazioni.vi" "Path settings"() -> (w183:path)
            n150 = Build Path(base path=w190, name or relative path="Settings grafici\\plots") -> (appended path=w184:path)
            n151 = Build Path(base path=w183, name or relative path="Settings grafici\\grafici") -> (appended path=w181:path)
            n152 = Open/Create/Replace File(file path (use dialog)=w184, operation (0:open)=T14."open or create") -> (refnum out=w188:refnum<file>, error out=w187:errorcluster)  [unwired: 4 in, 1 out]
            n153 = Open/Create/Replace File(file path (use dialog)=w181, operation (0:open)=T14."open or create") -> (refnum out=w195:refnum<file>, error out=w196:errorcluster)  [unwired: 4 in, 1 out]
            n154 = Read from Binary File(5:T5[] [{"ASSE X 1"={"NOME ASSE"="Time[s]", "AUTO\nSCALA?"=TRUE, "MIN"=0.0, "MAX"=0.0, "Colore asse"=16448250, "Griglie Maggiori"=0, "Griglie Minori"=0, "Decimali"=0}, "ASSE X 2"={"NOME ASSE"="", "AUTO\nSCALA?"=FALSE, "MIN"=0.0, "MAX"=0.0, "Colore asse"=16448250, "Griglie Maggiori"=0, "Griglie Minori"=0, "Decimali"=0}, "ASSE Y 1"={"NOME ASSE"="Voltage[V]", "AUTO\nSCALA?"=TRUE, "MIN"=0.0, "MAX"=0.0, "Colore asse"=16448250, "Griglie Maggiori"=0, "Griglie Minori"=0, "Decimali"=0}, "ASSE Y 2"={"NOME ASSE"="C[Nm]", "AUTO\nSCALA?"=FALSE, "MIN"=0.0, "MAX"=1.0, "Colore asse"=16448250, "Griglie Maggiori"=0, "Griglie Minori"=0, "Decimali"=0}, "ASSE Y 3"={"NOME ASSE"="Pot[kW]", "AUTO\nSCALA?"=FALSE, "MIN"=0.0, "MAX"=0.0, "Colore asse"=16448250, "Griglie Maggiori"=0, "Griglie Minori"=0, "Decimali"=0}, "ASSE Y 4"={"NOME ASSE"="eff[%]", "AUTO\nSCALA?"=FALSE, "MIN"=0.0, "MAX"=0.0, "Colore asse"=16448250, "Griglie Maggiori"=0, "Griglie Minori"=0, "Decimali"=0}, "X1"=TRUE, "X2"=FALSE, "Y1"=TRUE, "Y2"=FALSE, "Y3"=FALSE, "Y4"=FALSE, "NOME GRAFICO"="Voltage-Time", "PROVE ASSOCIATE"={"A FREDDO"=FALSE, "A VUOTO"=TRUE, "A CARICO"=FALSE, "TERMICA"=FALSE, "C.MECC."=FALSE, "ROT BLOCC"=FALSE, "GENERICA"=FALSE, "TABELLA RESISTOMAT"=FALSE, "SCORTA 2"=FALSE, "SCORTA 3"=FALSE}, "ASSE Y 5"={"NOME ASSE"="", "AUTO\nSCALA?"=FALSE, "MIN"=0.0, "MAX"=0.0, "Colore asse"=16448250, "Griglie Maggiori"=0, "Griglie Minori"=0, "Decimali"=0}, "Y5"=FALSE, "Colore sfondo grafico"=0}, {"ASSE X 1"={"NOME ASSE"="Voltage[V]", "AUTO\nSCALA?"=TRUE, "MIN"=0.0, "MAX"=0.0, "Colore asse"=16448250, "Griglie Maggiori"=0, "Griglie Minori"=0, "Decimali"=0}, "ASSE X 2"={"NOME ASSE"="", "AUTO\nSCALA?"=FALSE, "MIN"=0.0, "MAX"=0.0, "Colore asse"=16448250, "Griglie Maggiori"=0, "Griglie Minori"=0, "Decimali"=0}, "ASSE Y 1"={"NOME ASSE"="Current[A]", "AUTO\nSCALA?"=TRUE, "MIN"=0.0, "MAX"=0.0, "Colore asse"=16448250, "Griglie Maggiori"=0, "Griglie Minori"=0, "Decimali"=0}, "ASSE Y 2"={"NOME ASSE"="CosFi", "AUTO\nSCALA?"=FALSE, "MIN"=0.0, "MAX"=1.0, "Colore asse"=16860, "Griglie Maggiori"=0, "Griglie Minori"=0, "Decimali"=0}, "ASSE Y 3"={"NOME ASSE"="Pot[kW]", "AUTO\nSCALA?"=FALSE, "MIN"=0.0, "MAX"=0.0, "Colore asse"=16448250, "Griglie Maggiori"=0, "Griglie Minori"=0, "Decimali"=0}, "ASSE Y 4"={"NOME ASSE"="eff[%]", "AUTO\nSCALA?"=FALSE, "MIN"=0.0, "MAX"=0.0, "Colore asse"=16448250, "Griglie Maggiori"=0, "Griglie Minori"=0, "Decimali"=0}, "X1"=TRUE, "X2"=FALSE, "Y1"=TRUE, "Y2"=TRUE, "Y3"=FALSE, "Y4"=FALSE, "NOME GRAFICO"="I[A]-CosFi-Voltage", "PROVE ASSOCIATE"={"A FREDDO"=FALSE, "A VUOTO"=TRUE, "A CARICO"=FALSE, "TERMICA"=FALSE, "C.MECC."=FALSE, "ROT BLOCC"=FALSE, "GENERICA"=FALSE, "TABELLA RESISTOMAT"=FALSE, "SCORTA 2"=FALSE, "SCORTA 3"=FALSE}, "ASSE Y 5"={"NOME ASSE"="", "AUTO\nSCALA?"=FALSE, "MIN"=0.0, "MAX"=0.0, "Colore asse"=16448250, "Griglie Maggiori"=0, "Griglie Minori"=0, "Decimali"=0}, "Y5"=FALSE, "Colore sfondo grafico"=0}, {"ASSE X 1"={"NOME ASSE"="RPM", "AUTO\nSCALA?"=TRUE, "MIN"=0.0, "MAX"=0.0, "Colore asse"=16448250, "Griglie Maggiori"=0, "Griglie Minori"=0, "Decimali"=0}, "ASSE X 2"={"NOME ASSE"="", "AUTO\nSCALA?"=FALSE, "MIN"=0.0, "MAX"=0.0, "Colore asse"=0, "Griglie Maggiori"=0, "Griglie Minori"=0, "Decimali"=0}, "ASSE Y 1"={"NOME ASSE"="Coppia[Nm]", "AUTO\nSCALA?"=TRUE, "MIN"=0.0, "MAX"=0.0, "Colore asse"=16448250, "Griglie Maggiori"=0, "Griglie Minori"=0, "Decimali"=0}, "ASSE Y 2"={"NOME ASSE"="", "AUTO\nSCALA?"=FALSE, "MIN"=0.0, "MAX"=0.0, "Colore asse"=0, "Griglie Maggiori"=0, "Griglie Minori"=0, "Decimali"=0}, "ASSE Y 3"={"NOME ASSE"="", "AUTO\nSCALA?"=FALSE, "MIN"=0.0, "MAX"=0.0, "Colore asse"=0, "Griglie Maggiori"=0, "Griglie Minori"=0, "Decimali"=0}, "ASSE Y 4"={"NOME ASSE"="", "AUTO\nSCALA?"=FALSE, "MIN"=0.0, "MAX"=0.0, "Colore asse"=0, "Griglie Maggiori"=0, "Griglie Minori"=0, "Decimali"=0}, "X1"=TRUE, "X2"=FALSE, "Y1"=TRUE, "Y2"=FALSE, "Y3"=FALSE, "Y4"=FALSE, "NOME GRAFICO"="C-RPM", "PROVE ASSOCIATE"={"A FREDDO"=FALSE, "A VUOTO"=FALSE, "A CARICO"=FALSE, "TERMICA"=FALSE, "C.MECC."=TRUE, "ROT BLOCC"=FALSE, "GENERICA"=FALSE, "TABELLA RESISTOMAT"=FALSE, "SCORTA 2"=FALSE, "SCORTA 3"=FALSE}, "ASSE Y 5"={"NOME ASSE"="", "AUTO\nSCALA?"=FALSE, "MIN"=0.0, "MAX"=0.0, "Colore asse"=0, "Griglie Maggiori"=0, "Griglie Minori"=0, "Decimali"=0}, "Y5"=FALSE, "Colore sfondo grafico"=0}, {"ASSE X 1"={"NOME ASSE"="RPM", "AUTO\nSCALA?"=TRUE, "MIN"=0.0, "MAX"=0.0, "Colore asse"=16448250, "Griglie Maggiori"=0, "Griglie Minori"=0, "Decimali"=0}, "ASSE X 2"={"NOME ASSE"="", "AUTO\nSCALA?"=FALSE, "MIN"=0.0, "MAX"=0.0, "Colore asse"=0, "Griglie Maggiori"=0, "Griglie Minori"=0, "Decimali"=0}, "ASSE Y 1"={"NOME ASSE"="Coppia[Nm]", "AUTO\nSCALA?"=TRUE, "MIN"=0.0, "MAX"=0.0, "Colore asse"=16448250, "Griglie Maggiori"=0, "Griglie Minori"=0, "Decimali"=0}, "ASSE Y 2"={"NOME ASSE"="Corrente[A]", "AUTO\nSCALA?"=TRUE, "MIN"=0.0, "MAX"=0.0, "Colore asse"=16711680, "Griglie Maggiori"=0, "Griglie Minori"=0, "Decimali"=0}, "ASSE Y 3"={"NOME ASSE"="Potenza[kW]", "AUTO\nSCALA?"=TRUE, "MIN"=0.0, "MAX"=0.0, "Colore asse"=6618880, "Griglie Maggiori"=0, "Griglie Minori"=0, "Decimali"=0}, "ASSE Y 4"={"NOME ASSE"="eff[%]", "AUTO\nSCALA?"=TRUE, "MIN"=0.0, "MAX"=0.0, "Colore asse"=9567230, "Griglie Maggiori"=0, "Griglie Minori"=0, "Decimali"=0}, "X1"=TRUE, "X2"=FALSE, "Y1"=TRUE, "Y2"=TRUE, "Y3"=TRUE, "Y4"=TRUE, "NOME GRAFICO"="Cmecc", "PROVE ASSOCIATE"={"A FREDDO"=FALSE, "A VUOTO"=FALSE, "A CARICO"=FALSE, "TERMICA"=FALSE, "C.MECC."=TRUE, "ROT BLOCC"=FALSE, "GENERICA"=FALSE, "TABELLA RESISTOMAT"=FALSE, "SCORTA 2"=FALSE, "SCORTA 3"=FALSE}, "ASSE Y 5"={"NOME ASSE"="", "AUTO\nSCALA?"=FALSE, "MIN"=0.0, "MAX"=0.0, "Colore asse"=0, "Griglie Maggiori"=0, "Griglie Minori"=0, "Decimali"=0}, "Y5"=FALSE, "Colore sfondo grafico"=0}, {"ASSE X 1"={"NOME ASSE"="Tempo[s]", "AUTO\nSCALA?"=TRUE, "MIN"=0.0, "MAX"=0.0, "Colore asse"=16448250, "Griglie Maggiori"=0, "Griglie Minori"=0, "Decimali"=0}, "ASSE X 2"={"NOME ASSE"="", "AUTO\nSCALA?"=FALSE, "MIN"=0.0, "MAX"=0.0, "Colore asse"=0, "Griglie Maggiori"=0, "Griglie Minori"=0, "Decimali"=0}, "ASSE Y 1"={"NOME ASSE"="Temperatura[°C]", "AUTO\nSCALA?"=TRUE, "MIN"=0.0, "MAX"=0.0, "Colore asse"=16448250, "Griglie Maggiori"=0, "Griglie Minori"=0, "Decimali"=0}, "ASSE Y 2"={"NOME ASSE"="Corrente[A]", "AUTO\nSCALA?"=TRUE, "MIN"=0.0, "MAX"=0.0, "Colore asse"=16711680, "Griglie Maggiori"=0, "Griglie Minori"=0, "Decimali"=0}, "ASSE Y 3"={"NOME ASSE"="Potenza[kW]", "AUTO\nSCALA?"=TRUE, "MIN"=0.0, "MAX"=0.0, "Colore asse"=6618880, "Griglie Maggiori"=0, "Griglie Minori"=0, "Decimali"=0}, "ASSE Y 4"={"NOME ASSE"="eff[%]", "AUTO\nSCALA?"=TRUE, "MIN"=0.0, "MAX"=0.0, "Colore asse"=9567230, "Griglie Maggiori"=0, "Griglie Minori"=0, "Decimali"=0}, "X1"=TRUE, "X2"=FALSE, "Y1"=TRUE, "Y2"=FALSE, "Y3"=FALSE, "Y4"=FALSE, "NOME GRAFICO"="Temperature", "PROVE ASSOCIATE"={"A FREDDO"=FALSE, "A VUOTO"=FALSE, "A CARICO"=FALSE, "TERMICA"=TRUE, "C.MECC."=FALSE, "ROT BLOCC"=FALSE, "GENERICA"=FALSE, "TABELLA RESISTOMAT"=FALSE, "SCORTA 2"=FALSE, "SCORTA 3"=FALSE}, "ASSE Y 5"={"NOME ASSE"="", "AUTO\nSCALA?"=FALSE, "MIN"=0.0, "MAX"=0.0, "Colore asse"=0, "Griglie Maggiori"=0, "Griglie Minori"=0, "Decimali"=0}, "Y5"=FALSE, "Colore sfondo grafico"=0}, {"ASSE X 1"={"NOME ASSE"="Tempo[s]", "AUTO\nSCALA?"=TRUE, "MIN"=0.0, "MAX"=0.0, "Colore asse"=16448250, "Griglie Maggiori"=0, "Griglie Minori"=0, "Decimali"=0}, "ASSE X 2"={"NOME ASSE"="", "AUTO\nSCALA?"=FALSE, "MIN"=0.0, "MAX"=0.0, "Colore asse"=0, "Griglie Maggiori"=0, "Griglie Minori"=0, "Decimali"=0}, "ASSE Y 1"={"NOME ASSE"="Potenza[W]", "AUTO\nSCALA?"=TRUE, "MIN"=0.0, "MAX"=0.0, "Colore asse"=16448250, "Griglie Maggiori"=0, "Griglie Minori"=0, "Decimali"=0}, "ASSE Y 2"={"NOME ASSE"="Corrente[A]", "AUTO\nSCALA?"=TRUE, "MIN"=0.0, "MAX"=0.0, "Colore asse"=16711680, "Griglie Maggiori"=0, "Griglie Minori"=0, "Decimali"=0}, "ASSE Y 3"={"NOME ASSE"="Potenza[kW]", "AUTO\nSCALA?"=TRUE, "MIN"=0.0, "MAX"=0.0, "Colore asse"=6618880, "Griglie Maggiori"=0, "Griglie Minori"=0, "Decimali"=0}, "ASSE Y 4"={"NOME ASSE"="eff[%]", "AUTO\nSCALA?"=TRUE, "MIN"=0.0, "MAX"=0.0, "Colore asse"=9567230, "Griglie Maggiori"=0, "Griglie Minori"=0, "Decimali"=0}, "X1"=TRUE, "X2"=FALSE, "Y1"=TRUE, "Y2"=TRUE, "Y3"=FALSE, "Y4"=FALSE, "NOME GRAFICO"="Power-Time", "PROVE ASSOCIATE"={"A FREDDO"=FALSE, "A VUOTO"=FALSE, "A CARICO"=TRUE, "TERMICA"=TRUE, "C.MECC."=FALSE, "ROT BLOCC"=FALSE, "GENERICA"=FALSE, "TABELLA RESISTOMAT"=FALSE, "SCORTA 2"=FALSE, "SCORTA 3"=FALSE}, "ASSE Y 5"={"NOME ASSE"="", "AUTO\nSCALA?"=FALSE, "MIN"=0.0, "MAX"=0.0, "Colore asse"=0, "Griglie Maggiori"=0, "Griglie Minori"=0, "Decimali"=0}, "Y5"=FALSE, "Colore sfondo grafico"=0}] ("Grafici"), 8:w196, 11:w195) -> (0:w193:errorcluster, 2:w186:T5[], 3:w192:refnum<file>)  [unwired: 3 in, 1 out]
            n155 = Read from Binary File(5:T4[] [], 8:w187, 11:w188) -> (0:w197:errorcluster, 2:w185:T4[], 3:w198:refnum<file>)  [unwired: 3 in, 1 out]
            n156 = Close File(refnum=w192, error in=w193) -> ()  [unwired: 2 out]
            n157 = Close File(refnum=w198, error in=w197) -> ()  [unwired: 2 out]
            n158 = local write "Plots"(w185) -> ()
            n159 = local write "Grafici"(w186) -> ()
          }
        }
      }
      event "AGGIORNA IMM": Value Change {
        n160 = event-data() -> ()  [unwired: 1 in, 6 out]
        n161 = Enqueue Element(queue=w200, element=cluster{"String":string, "variant":variant} {"String"="AGGIORNA IMMAGINI", "variant"=variant}) -> ()  [unwired: 2 in, 3 out]
      }
      event "REPORT C2K": Value Change {
        n162 = event-data() -> ()  [unwired: 1 in, 6 out]
        n163 = Enqueue Element(queue=w202, element=cluster{"String":string, "variant":variant} {"String"="REPORT C2K", "variant"=variant}) -> ()  [unwired: 2 in, 3 out]
      }
      event "CERCA COLLAUDO": Value Change {
        n164 = event-data() -> ("NewVal"=w206:bool)  [unwired: 1 in, 5 out]
        n165 = case shown="True" w206 {
          tunnel: w204 -> [_ w207]
          frame False {
          }
          frame True {
            n166 = flat-sequence {
              tunnel: [w212] -> w209
              tunnel: w207 -> [w211]
              tunnel: w209 -> [w217]
              tunnel: [w217] -> w208
              tunnel: w208 -> [w218]
              frame #0 {
                n167 = call "CRITERI RICERCA.vi"("banco"=w211, "String 2"="RICERCA COLLAUDI", "Confronti?"=FALSE) -> ("ANNULLA"=w212:bool, "Collaudo selezionato"=w213:string, "Campo descrittivo collaudo"=w210:string)  [unwired: 2 in, 4 out]
                n168 = local write "COLLAUDO PRINCIPALE"(w213) -> ()
                n169 = local write "Descrizione princ"(w210) -> ()
              }
              frame #1 {
                n170 = Wait (ms)(milliseconds to wait=u32 200) -> ()  [unwired: 1 out]
              }
              frame #2 {
                n171 = case shown="False" w218 {
                  frame False {
                    n172 = property on="CARICA COLLAUDI" class="Bool (strict)"("Val(Sgnl)"=TRUE ("Value (Signaling)")) -> ()  [unwired: 2 in, 2 out]
                  }
                  frame True {
                  }
                }
              }
            }
          }
        }
        n173 = local write "CERCA COLLAUDO"(FALSE ("CERCA COLLAUDO")) -> ()
      }
      event "toll Q", "toll H", "toll P2": Value Change {
        n174 = event-data() -> ()  [unwired: 1 in, 6 out]
        n175 = local read "Case carica grafici"() -> (w220:string)
        n176 = Bundle By Name(cluster=cluster{"String":string, "variant":variant} {"String"="Grafica", "variant"=variant} ("element"), "String"=w220) -> (w221:cluster{"String":string, "variant":variant})
        n177 = Enqueue Element(queue=w223, element=w221) -> ()  [unwired: 2 in, 3 out]
      }
      event "CERCA COLLAUDO DI CONFRONTO": Value Change {
        n178 = event-data() -> ("NewVal"=w225:bool)  [unwired: 1 in, 5 out]
        n179 = local read "COLLAUDO PRINCIPALE"() -> (w227:string)
        n180 = Not Equal?(x=w227, y="") -> (x != y?=w224:bool)
        n181 = case shown="True" w224 {
          tunnel: w228 -> [_ w232]
          tunnel: w225 -> [_ w231]
          frame False {
            n182 = One Button Dialog(message="Caricare prima il collaudo principale") -> ()  [unwired: 1 in, 1 out]
          }
          frame True {
            n183 = case shown="True" w231 {
              tunnel: w232 -> [_ w233]
              frame False {
              }
              frame True {
                n184 = flat-sequence {
                  tunnel: [w238] -> w234
                  tunnel: w233 -> [w237]
                  tunnel: w234 -> [w242]
                  frame #0 {
                    n185 = local read "COLLAUDI DI CONFRONTO"() -> (w236:string[])
                    n186 = call "CRITERI RICERCA.vi"("banco"=w237, "collaudi di confronto in"=w236, "String 2"="COLLAUDI DI CONFRONTO", "Confronti?"=TRUE) -> ("ANNULLA"=w238:bool, "collaudi di confronto"=w239:string[], "Campi descrittivi confronto"=w235:string[])  [unwired: 1 in, 4 out]
                    n187 = local write "COLLAUDI DI CONFRONTO"(w239) -> ()
                    n188 = local write "Descrizione"(w235) -> ()
                  }
                  frame #1 {
                    n189 = case shown="False" w242 {
                      frame False {
                        n190 = property on="CARICA COLLAUDI" class="Bool (strict)"("Val(Sgnl)"=TRUE ("Value (Signaling)")) -> ()  [unwired: 2 in, 2 out]
                      }
                      frame True {
                      }
                    }
                  }
                }
              }
            }
          }
        }
        n191 = local write "CERCA COLLAUDO DI CONFRONTO"(FALSE ("CERCA COLLAUDO")) -> ()
      }
      event "REPORT EXCEL": Value Change {
        n192 = event-data() -> ("NewVal"=w244:bool)  [unwired: 1 in, 5 out]
        n193 = case shown="True" w244 {
          tunnel: w245 -> [_ w246]
          frame False {
          }
          frame True {
            n194 = Enqueue Element(queue=w246, element=cluster{"String":string, "variant":variant} {"String"="REPORT EXCEL", "variant"=variant}) -> ()  [unwired: 2 in, 3 out]
          }
        }
      }
      event "SALVA COME DEFAULT": Value Change {
        n195 = event-data() -> ("NewVal"=w250:bool)  [unwired: 1 in, 5 out]
        n196 = case shown="True" w250 {
          tunnel: w249 -> [_ w251]
          frame False {
          }
          frame True {
            n197 = Enqueue Element(queue=w251, element=cluster{"String":string, "variant":variant} {"String"="SALVA COME DEFAULT", "variant"=variant}) -> ()  [unwired: 2 in, 3 out]
          }
        }
        n198 = local write "SALVA COME DEFAULT"(FALSE ("SALVA COME DEFAULT")) -> ()
      }
      event "SALVA IMPOSTAZIONI ESP MODELLO": Value Change {
        n199 = event-data() -> ("NewVal"=w254:bool)  [unwired: 1 in, 5 out]
        n200 = case shown="True" w254 {
          tunnel: w255 -> [_ w256]
          frame False {
          }
          frame True {
            n201 = Enqueue Element(queue=w256, element=cluster{"String":string, "variant":variant} {"String"="SALVA IMP ESPORTAZIONE", "variant"=variant}) -> ()  [unwired: 2 in, 3 out]
          }
        }
        n202 = local write "SALVA IMPOSTAZIONI ESP MODELLO"(FALSE ("SALVA IMPOSTAZIONI ESP MODELLO")) -> ()
      }
      event "Carica impostazioni modello": Value Change {
        n203 = event-data() -> ()  [unwired: 1 in, 6 out]
        n204 = global read "Global percorso impostazioni.vi" "Path settings"() -> (w260:path)
        n205 = property on="SCEGLI MODELLO" class="CmbBox"() -> ("Text.Text"=w264:string)  [unwired: 2 in, 2 out]
        n206 = Search and Replace String(input string=w264, search string=".", replace string="_" ("replace string (\"\")")) -> (result string=w263:string)  [unwired: 5 in, 3 out]
        n207 = Build Path(base path=w260, name or relative path="Settings grafici") -> (appended path=w268:path)
        n208 = Concatenate Strings("IMPOSTAZIONI_ESPORTAZIONE_", w263) -> (w262:string)
        n209 = Build Path(base path=w268, name or relative path=w262) -> (appended path=w261:path)
        n210 = Open/Create/Replace File(file path (use dialog)=w261, operation (0:open)=T14."open") -> (refnum out=w276:refnum<file>, error out=w274:errorcluster)  [unwired: 4 in, 1 out]
        n211 = Read from Binary File(5:T20 {"Nome fogli"=[], "Nome fogli GENERICHE"=[]} ("output cluster"), 8:w274, 11:w276) -> (0:w273:errorcluster, 2:w272:T20, 3:w275:refnum<file>)  [unwired: 3 in, 1 out]
        n212 = Unbundle By Name(w272) -> ("Nome fogli"=w270:T13, "Nome fogli GENERICHE"=w271:T12)
        n213 = Close File(refnum=w275, error in=w273) -> (error out=w259:errorcluster)  [unwired: 1 out]
        n214 = call <vilib>:"Clear Errors.vi"("error in (no error)"=w259) -> ()  [unwired: 5 in, 2 out]
        n215 = local write "Nome fogli GENERICHE"(w271) -> ()
        n216 = local write "Nome fogli"(w270) -> ()
      }
      event "Aggiungi criterio": Value Change {
        n217 = event-data() -> ()  [unwired: 1 in, 6 out]
        n218 = control-ref of="Criteri di salvataggio report"() -> (w279:refnum<vi>)
        n219 = local write "Aggiungi criterio"(FALSE ("Aggiungi criterio")) -> ()
        n220 = call "Criteri salvataggii report.vi"("Default?"=FALSE) -> ("ANNULLA?"=w281:bool, "OUT"=w282:string[])  [unwired: 9 in]
        n221 = case shown="False" w281 {
          tunnel: w282 -> [w291 _]
          tunnel: w279 -> [w290 _]
          frame False {
            (unwired) 2 ("index")
            n222 = property class="MCListbox (strict)"(reference=w290) -> (reference out=w289:refnum<vi>, "ItemNames"=w288:string[][])  [unwired: 1 in, 1 out]
            n223 = Build Array (concatenate)(w288, w291) -> (w287:string[][])
            n224 = property class="MCListbox (strict)"(reference=w289, "ItemNames"=w287) -> (reference out=w284:refnum<vi>, error out=w283:errorcluster)  [unwired: 1 in]
            n225 = flat-sequence {
              tunnel: [w293] -> w286
              tunnel: w283 -> [w293]
              tunnel: [w292] -> w285
              tunnel: w284 -> [w292]
              tunnel: w286 -> [_]
              tunnel: w285 -> [w295]
              frame #0 {
                n226 = Wait (ms)(milliseconds to wait=u32 150) -> ()  [unwired: 1 out]
              }
              frame #1 {
                n227 = call "Auto width colum table.vi"("spazi"=i16 10, "Real Time tabella"=w295) -> ()  [unwired: 9 in, 1 out]
              }
            }
          }
          frame True {
          }
        }
      }
      event "Elimina criterio": Value Change {
        n228 = event-data() -> ()  [unwired: 1 in, 6 out]
        n229 = control-ref of="Criteri di salvataggio report"() -> (w301:refnum<vi>)
        n230 = property class="MCListbox (strict)"(reference=w301) -> (reference out=w302:refnum<vi>, "ItemNames"=w300:string[][], "Value"=w299:i32)  [unwired: 1 in, 1 out]
        n231 = Delete From Array(array=w300, length=1, index (row)=w299) -> (array with subset deleted=w297:string[][])  [unwired: 1 in, 1 out]
        n232 = property class="MCListbox (strict)"(reference=w302, "ItemNames"=w297) -> ()  [unwired: 1 in, 2 out]
      }
      event "Modifica percorso default": Value Change {
        n233 = event-data() -> ()  [unwired: 1 in, 6 out]
        n234 = control-ref of="Percorso e nome di DEFAULT"() -> (w304:refnum<vi>)
        n235 = local write "Modifica percorso default"(FALSE ("Modifica percorso default")) -> ()
        n236 = call "Criteri salvataggii report.vi"("Default?"=TRUE) -> ("ANNULLA?"=w306:bool, "OUT"=w307:string[])  [unwired: 9 in]
        n237 = case shown="False" w306 {
          tunnel: w307 -> [w313 _]
          tunnel: w304 -> [w314 _]
          frame False {
            (unwired) 2 ("index")
            n238 = Build Array(w313) -> (w312:string[][])
            n239 = property class="MCListbox (strict)"(reference=w314, "ItemNames"=w312) -> (reference out=w309:refnum<vi>, error out=w308:errorcluster)  [unwired: 1 in]
            n240 = flat-sequence {
              tunnel: [w316] -> w311
              tunnel: w308 -> [w316]
              tunnel: [w315] -> w310
              tunnel: w309 -> [w315]
              tunnel: w311 -> [_]
              tunnel: w310 -> [w318]
              frame #0 {
                n241 = Wait (ms)(milliseconds to wait=u32 150) -> ()  [unwired: 1 out]
              }
              frame #1 {
                n242 = call "Auto width colum table.vi"("spazi"=i16 10, "Real Time tabella"=w318) -> ()  [unwired: 9 in, 1 out]
              }
            }
          }
          frame True {
          }
        }
      }
      event "exit": Value Change; Panel Close {
        n243 = event-data() -> ()  [unwired: 1 in, 3 out]
        n244 = property on="REPORT EXCEL" class="Bool (strict)"() -> ("Visible"=w320:bool)  [unwired: 2 in, 2 out]
        n245 = case shown="True" w320 {
          tunnel: w321 -> [_ w324]
          frame False {
            n246 = One Button Dialog(message="Attendere la fine della\ncreazione del report excel") -> ()  [unwired: 1 in, 1 out]
          }
          frame True {
            n247 = Enqueue Element(queue=w324, element=cluster{"String":string, "variant":variant} {"String"="exit", "variant"=variant}) -> ()  [unwired: 2 in, 3 out]
          }
        }
      }
    }
  }
  n248 = while {
    tunnel: w73 -> [w355]
    tunnel: w76 -> [w354]
    shift-right: [w349] -> _
    shift-left: _ -> [w348]
    shift-right: [w347] -> _
    shift-left: _ -> [w346]
    shift-right: [w345] -> _
    shift-left: _ -> [w344]
    shift-right: [w342] -> _
    shift-left: w48 -> [w343]
    tunnel: w67 -> [w341]
    tunnel: w66 -> [w339]
    tunnel: w65 -> [_]
    tunnel: w64 -> [w340]
    tunnel: w63 -> [w337]
    tunnel: w62 -> [w336]
    shift-right: [w334] -> _
    shift-left: w47 -> [w335]
    tunnel: "Report collaudo in corso?" -> [w333]
    tunnel: w48 -> [w332]
    tunnel: w47 -> [w331]
    shift-right: [w328] -> _
    shift-left: w40 -> [w329]
    tunnel: w40 -> [w330]
    tunnel: w3 -> [w326]
    i -> [w327]
    stop <- w351 stop-if-true
    n249 = Dequeue Element(queue=w355, error in (no error)=w354) -> (queue out=w338:refnum<queue>, element=w353:cluster{"String":string, "variant":variant})  [unwired: 1 in, 2 out]
    n250 = Unbundle(w353) -> ("String"=w352:string, "variant"=w350:variant)
    "state" <- w352
    n251 = case shown="\"REPORT EXCEL\"" w352 {
      selector: w352 -> [_ _ _ _ _ _ _ _ _ _ _ _ _ w1259 w1557 w1771 _ _ _ _]
      tunnel: [_ _ _ _ _ _ _ _ _ _ _ _ _ _ _ _ _ _ _ TRUE] -> w351
      tunnel: w350 -> [_ _ _ _ _ _ _ _ _ _ _ _ _ _ _ _ _ _ _ _]
      tunnel: [w368 w386 w392 w451 w704 w772 w876 w923 w988 w1099 w1121 w1163 w1180 w1265 w1563 w1775 w1993 w2142 w2172 w2993] -> w349
      tunnel: w348 -> [w368 w386 w392 _ w704 w772 w876 w923 w988 w1099 w1121 w1163 w1180 w1265 w1563 w1775 w1993 w2142 w2172 w2993]
      tunnel: [w370 w389 w395 w497 w703 w758 w872 w928 w987 w1098 w1120 w1162 w1183 w1267 w1565 w1777 w1992 w2141 w2186 w2991] -> w347
      tunnel: w346 -> [w370 w389 w395 w497 w703 w758 w872 w928 w987 w1098 w1120 w1162 _ w1267 w1565 w1777 w1992 w2141 w2186 w2991]
      tunnel: [w369 w385 w391 w399 w702 w759 w871 w925 w982 w1097 w1119 w1161 w1181 w1266 w1564 w1776 w1991 w2140 w2184 w2992] -> w345
      tunnel: w344 -> [w369 w385 w391 w491 w702 w759 w871 w925 w983 w1097 w1119 w1161 w1181 w1266 w1564 w1776 w1991 w2140 w2184 w2992]
      tunnel: w343 -> [w371 w390 w396 w496 w701 w771 w875 w927 w986 w1096 w1118 w1160 w1182 _ w1559 w1772 w1988 w2139 w2185 w2990]
      tunnel: [w371 w390 w396 w496 w701 w771 w875 w927 w986 w1096 w1118 w1160 w1182 w1264 w1559 w1772 w1988 w2139 w2185 w2990] -> w342
      tunnel: w341 -> [_ _ _ _ _ _ _ _ _ _ _ _ _ w1263 w1561 w1773 _ _ w2176 _]
      tunnel: w340 -> [_ _ _ _ _ _ _ _ _ _ _ _ w1179 _ _ _ _ _ _ _]
      tunnel: w339 -> [_ _ _ _ _ _ _ _ _ _ _ _ w1178 _ _ _ _ _ _ _]
      tunnel: w338 -> [w365 _ _ w452 w687 _ _ _ w980 _ _ w1158 _ w1260 w1562 w1774 w1990 _ _ _]
      tunnel: w337 -> [_ _ _ _ _ _ _ _ _ _ _ _ _ _ _ _ _ _ _ _]
      tunnel: w336 -> [_ _ _ _ _ _ _ _ _ _ _ _ _ _ _ _ _ _ _ _]
      tunnel: w335 -> [w367 w388 w394 w495 w700 w770 w874 w924 w985 w1095 w1117 w1159 w1177 w1262 _ w1768 w1989 w2138 w2183 w2989]
      tunnel: [w367 w388 w394 w495 w700 w770 w874 w924 w985 w1095 w1117 w1159 w1177 w1262 w1560 w1768 w1989 w2138 w2183 w2989] -> w334
      tunnel: w333 -> [w366 _ _ w406 _ _ _ _ _ _ _ _ _ _ _ _ _ _ w2153 _]
      tunnel: w332 -> [_ _ _ _ _ _ _ _ _ _ _ _ _ w1261 _ _ _ _ _ _]
      tunnel: w331 -> [_ _ _ _ _ _ _ _ _ _ _ _ _ _ w1558 _ _ _ _ _]
      tunnel: w330 -> [_ _ _ _ _ _ _ _ _ _ _ _ _ _ _ w1770 _ _ _ _]
      tunnel: w329 -> [w360 w387 w393 w490 w699 w769 w873 w926 w984 w1094 w1116 w1156 w1174 w1258 w1556 _ w1987 w2132 w2177 w2988]
      tunnel: [w360 w387 w393 w490 w699 w769 w873 w926 w984 w1094 w1116 w1156 w1174 w1258 w1556 w1769 w1987 w2132 w2177 w2988] -> w328
      tunnel: w326 -> [w357 _ _ w403 _ _ _ _ _ _ _ _ _ _ _ _ _ _ _ _]
      frame "Initialize", Default {
        n252 = local read "COLLAUDO PRINCIPALE"() -> (w364:string)
        n253 = Empty String/Path?(string/path=w364) -> (empty?=w363:bool)
        n254 = Not(x=w363) -> (.not. x?=w361:bool)
        n255 = And(x=w366, y=w361) -> (x .and. y?=w362:bool)
        n256 = for {
          tunnel: w357 -> [w373] mode=indexing
          tunnel: [w372] -> w356 mode=indexing
          n257 = Index Array(array=w373, index=11 ("disabled index (col)")) -> (element=w372:string)
        }
        n258 = local read "Percorso modelli xls"() -> (w358:path)
        n259 = case shown="True" w362 {
          tunnel: w365 -> [_ w383]
          frame False {
          }
          frame True {
            n260 = Enqueue Element(queue=w383, element=cluster{"String":string, "variant":variant} {"String"="Carica dati collaudo", "variant"=variant}) -> ()  [unwired: 2 in, 3 out]
          }
        }
        n261 = for {
          tunnel: w358 -> [w378]
          tunnel: w356 -> [w376] mode=indexing
          tunnel: [w377] -> w359 mode=concatenating
          n262 = Empty String/Path?(string/path=w376) -> (empty?=w375:bool)
          n263 = case shown="False" w375 {
            tunnel: w378 -> [w382 _]
            tunnel: [w381 _] -> w377
            tunnel: w376 -> [w379 _]
            frame False {
              n264 = Build Path(base path=w382, name or relative path=w379) -> (appended path=w380:path)
              n265 = List Folder(path=w380) -> (filenames=w381:string[])  [unwired: 3 in, 3 out]
            }
            frame True {
            }
          }
        }
        n266 = property on="SCEGLI MODELLO" class="CmbBox"("Strings[]"=w359) -> ()  [unwired: 2 in, 2 out]
      }
      frame "Carica collaudo in corso" {
      }
      frame "Carica tutte le prove" {
      }
      frame "Carica dati collaudo" {
        w397 = i16 1 ("TABELLA GENERICA")
        w448 = 6  # INDICE Collegamento
        w474 = "Bollettini" ("table")
        n267 = case shown="True" w406 {
          tunnel: w452 -> [w507 w510]
          tunnel: cluster{"variant":variant} {"variant"=variant} ("element") -> [_ _]
          frame False {
            n268 = Enqueue Element(queue=w507, element=cluster{"String":string, "variant":variant} {"String"="Carica collaudi di confronto", "variant"=variant}) -> (queue out=w506:refnum<queue>)  [unwired: 2 in, 2 out]
            n269 = Enqueue Element(queue=w506, element=cluster{"String":string, "variant":variant} {"String"="Aggiorna tabelle", "variant"=variant}) -> ()  [unwired: 2 in, 3 out]
          }
          frame True {
            n270 = Enqueue Element(queue=w510, element=cluster{"String":string, "variant":variant} {"String"="REPORT EXCEL", "variant"=variant}) -> ()  [unwired: 2 in, 3 out]
          }
        }
        n271 = local read "COLLAUDO PRINCIPALE"() -> (w467:string)
        n272 = call "MDB Reference.vi"("Collaudi T/motori F"=TRUE) -> ("error out"=w470:errorcluster, "Refnum out"=w473:T26)  [unwired: 8 in, 1 out]
        n273 = Spreadsheet String To Array(delimiter (Tab)="--", format string="", spreadsheet string=w467, array type (2D Dbl)=w467) -> (array=w484:string[][])
        n274 = Index Array(array=w484, index (row)=0) -> (element=w482:string[])  [unwired: 1 in]
        n275 = call "load string.vi"("Array in"=string[] ["Banco = '", "' AND Anno =", " AND Numero ="], "Codice"=w467) -> ("String command"=w475:string)  [unwired: 7 in, 2 out]
        n276 = call <vilib>:"DB Tools List Columns.vi"("error in (no error)"=w470, "table"=w474, "connection reference"=w473) -> ("error out"=w468:errorcluster, "columns"=w453:string[], "connection reference out"=w471:T26)  [unwired: 1 in, 1 out]
        n277 = Index Array(array=w482) -> (element #1=w481:string, element #2=w477:string, element #3=w478:string)  [unwired: 3 in]
        n278 = local read "Percorso modelli xls"() -> (w447:path)
        n279 = call <vilib>:"DB Tools Select Data.vi"("condition"=w475, "error in (no error)"=w468, "table"=w474, "connection reference"=w471) -> ("error out"=w469:errorcluster, "data"=w465:variant[][], "connection reference out"=w472:T26)  [unwired: 2 in]
        n280 = Bundle By Name(cluster="input cluster", "BANCO"=w481, "ANNO"=w477, "PROGRESSIVO"=w478) -> (w479:T1)
        n281 = control-ref of="This VI"() -> (w461:refnum<vi>)
        n282 = xnode "Database Variant To Data"("database variant"=w465, "type"=string[][] [] ("Item Names")) -> ("data"=w450:string[][])  [unwired: 1 in, 1 out]
        n283 = Index Array(array=w450, index (row)=0, index (col)=w448) -> (element=w404:string)
        "element" <- w404
        n284 = property class="VI"(reference=w461) -> ("Panel"=w460:refnum<vi>)  [unwired: 1 in, 2 out]
        n285 = Build Array (concatenate)(w453, w450) -> (w451:string[][])
        n286 = call "da TIPO a ID.vi"("TIPO"=w404) -> ("ID"=w402:i32)  [unwired: 10 in]
        "ID COLLEGAMENTO" <- w402
        n287 = for {
          tunnel: w403 -> [w501] mode=indexing
          tunnel: w402 -> [w504]
          tunnel: [w499] -> w401 mode=indexing if=w498
          n288 = Number To Decimal String(number=w504) -> (decimal integer string=w502:string)  [unwired: 1 in]
          n289 = Index Array(array=w501, index #1=0 ("disabled index (col)"), index #2=11 ("index")) -> (element #1=w503:string, element #2=w499:string)
          n290 = Equal?(x=w502, y=w503) -> (x = y?=w498:bool)
        }
        n291 = Transpose 2D Array(2D array=w451) -> (transposed array=w463:string[][])
        n292 = property class="Pnl"(reference=w460, "DeferPanUpdts"=TRUE ("Defer Panel Updates")) -> (reference out=w458:refnum<vi>, error out=w459:errorcluster)  [unwired: 1 in]
        n293 = Index Array(array=w463, index (col)=0 ("disabled index (col)")) -> (element=w462:string[])  [unwired: 1 in]
        n294 = local write "TABELLA GENERICA"(w397) -> ()
        n295 = local write "TABELLA A CARICO"(w397) -> ()
        n296 = local write "TABELLA TERMICA"(w397) -> ()
        n297 = local write "TABELLA A ROT BLOCC"(w397) -> ()
        n298 = local write "TABELLA CMECC"(w397) -> ()
        n299 = local write "TABELLA A VUOTO"(w397) -> ()
        n300 = local write "VISUALIZZA TABELLA"(i8 1 ("VISUALIZZA TABELLA")) -> ()
        n301 = for {
          tunnel: w463 -> [w554]
          tunnel: w462 -> [w541] mode=indexing
          tunnel: w459 -> [w537]
          tunnel: [w537] -> w456
          tunnel: [w536] -> w457
          tunnel: w458 -> [w536]
          i -> [w544]
          n302 = String Subset(string=w541, offset (0)=0, length (rest)=2 ("length (rest)")) -> (substring=w538:string)
          n303 = Search 1D Array(1D array=string[] ["P_", "M_", "C_"], element=w538) -> (index of element=w552:i32)  [unwired: 1 in]
          n304 = Increment(x=w552) -> (x+1=w546:i32)
          n305 = Build Array(u32 13816530, u32 13631231, u32 16762457, u32 15461355) -> (w547:u32[])
          n306 = Index Array(array=w547, index=w546) -> (element=w542:u32)
          n307 = Bundle By Name(cluster=T22 {"Row"=-2, "Column"=0} ("Active Cell:Active Cell"), "Row"=w544) -> (w543:T22)
          n308 = property on="Dati collaudo principale" class="MCListbox (strict)"("ItemNames"=w554, "ActiveCell"=w543, "CellBG"=w542, "CellFontBold"=TRUE ("Active Cell:Cell Font:Bold")) -> ()  [unwired: 2 in, 2 out]
        }
        n309 = Index Array(array=w401) -> (element=w400:string)  [unwired: 1 in]
        n310 = Build Path(base path=w447, name or relative path=w400) -> (appended path=w446:path)
        "Cartella modello" <- w446
        n311 = call "Leggi filtro ed etichette.vi"("ID COLLEGAMENTO"=w402) -> ("FILTRO"=w494:bool[], "ETICHETTE"=→"ETICHETTE":string[])  [unwired: 5 in, 4 out]
        n312 = List Folder(path=w446) -> (filenames=w445:string[])  [unwired: 3 in, 3 out]
        n313 = property on="SCELTA MODELLO XLS" class="LstBox (strict)"("Item Names"=w445) -> (error out=w420:errorcluster)  [unwired: 2 in, 1 out]
        n314 = for {
          N: 21 -> [_]
          tunnel: w472 -> [w627]
          tunnel: w469 -> [w626]
          tunnel: w494 -> [w624]
          shift-right: [w616] -> w399
          shift-left: w491 -> [w620]
          tunnel: w402 -> [w603]
          tunnel: [w602] -> w489
          tunnel: [w601] -> w488
          tunnel: w479 -> [w600]
          i -> [w615]
          # "carica misure prove tranne mei"
          n315 = Unbundle By Name(w600) -> ("BANCO"=w608:string, "ANNO"=w611:string, "PROGRESSIVO"=w614:string)
          n316 = Number To Decimal String(number=w615) -> (decimal integer string=w604:string)  [unwired: 1 in]
          n317 = Concatenate Strings("where Banco ='" ("string"), w608, "' AND Anno =" ("string"), w611, " AND Numero =" ("string"), w614, " AND Tipo_test_num =" ("string"), w604, " ORDER BY Progressivo_Acq" ("string")) -> (w625:string)
          n318 = Equal?(x=w608, y="collaudo inesistente") -> (x = y?=w606:bool)
          n319 = case shown="False" w606 {
            tunnel: w627 -> [w635 w683]
            tunnel: w626 -> [w634 _]
            tunnel: w625 -> [w633 _]
            tunnel: [w631 string[][] []] -> w623
            tunnel: [w629 w683] -> w602
            tunnel: [w628 _] -> w601
            frame False {
              n320 = call <vilib>:"DB Tools Select Data.vi"("condition"=w633, "error in (no error)"=w634, "table"="misure", "connection reference"=w635) -> ("error out"=w637:errorcluster, "data"=w638:variant[][], "connection reference out"=w629:T26)  [unwired: 2 in]
              n321 = xnode "Database Variant To Data"("database variant"=w638, "error in (no error)"=w637, "type"=string[][] []) -> ("data"=w630:string[][], "error out"=w628:errorcluster)
              n322 = Transpose 2D Array(2D array=w630) -> (transposed array=w631:string[][])
            }
            frame True {
            }
          }
          n323 = local read "VISUALIZZA TABELLA"() -> (w619:i8)
          n324 = for {
            tunnel: w624 -> [w685] mode=indexing
            tunnel: w623 -> [w686] mode=indexing
            tunnel: [w686] -> w622 mode=indexing if=w685
          }
          n325 = Transpose 2D Array(2D array=w622) -> (transposed array=w618:string[][])
          n326 = call "Correggi separatore decimale.vi"("Array in"=w618) -> ("Array out"=w621:string[][])  [unwired: 10 in]
          n327 = call "carica dati prove.vi"("TIPO COLLEGAMENTO"=w603, "Dati in"=w621, "Tabella"=w619, "prova"=w604, "Dati prove in"=w620) -> ("Dati prove out"=w617:T27)  [unwired: 4 in, 2 out]
          n328 = Bundle By Name(cluster=w617, "nome collaudo"=w614) -> (w616:T27)
        }
        n329 = property class="Pnl"(reference=w457, error in=w456, "DeferPanUpdts"=FALSE ("Defer Panel Updates")) -> ()  [unwired: 2 out]
        n330 = property on="SCELTA MODELLO XLS" class="LstBox (strict)"(error in=w420) -> ("Item Names"=w443:string[], "Value"=w442:i32)  [unwired: 1 in, 2 out]
        n331 = local write "ID Colleg confronti"(i32[] [] ("ID Colleg confronti")) -> ()
        n332 = Index Array(array=w443, index=w442) -> (element=w422:string)
        n333 = Search and Replace String(input string=w422, search string=".", replace string="_" ("replace string (\"\")")) -> (result string=w428:string)  [unwired: 5 in, 3 out]
        n334 = global read "Global percorso impostazioni.vi" "Path settings"() -> (w423:path)
        n335 = Concatenate Strings("Settings grafici\\IMPOSTAZIONI_GRAFICI_REPORT_" ("name or relative path"), w428) -> (w425:string)
        n336 = Build Path(base path=w423, name or relative path=w425) -> (appended path=w421:path)
        n337 = Open/Create/Replace File(file path (use dialog)=w421, operation (0:open)=T14."open or create") -> (refnum out=w431:refnum<file>, error out=w430:errorcluster)  [unwired: 4 in, 1 out]
        n338 = Read from Binary File(5:T21 {"Array Grafici A VUOTO"=[], "Array Grafici A CARICO"=[], "Array Grafici TERMICA"=[], "Array Grafici CMECC"=[], "Array Grafici ROTBLOCC"=[], "Array Grafici GENERICA"=[]} ("output cluster"), 8:w430, 11:w431) -> (0:w434:errorcluster, 2:w433:T21, 3:w435:refnum<file>)  [unwired: 3 in, 1 out]
        n339 = Unbundle By Name(w433) -> ("Array Grafici A VUOTO"=w436:T8[], "Array Grafici A CARICO"=w437:T8[], "Array Grafici TERMICA"=w438:T8[], "Array Grafici CMECC"=w439:T8[], "Array Grafici ROTBLOCC"=w440:T8[], "Array Grafici GENERICA"=w441:T8[])
        n340 = Close File(refnum=w435, error in=w434) -> (error out=w419:errorcluster)  [unwired: 1 out]
        n341 = call <vilib>:"Clear Errors.vi"("error in (no error)"=w419) -> ()  [unwired: 5 in, 2 out]
        n342 = for {
          tunnel: w436 -> [w535] mode=indexing
          tunnel: [w533] -> w407 mode=indexing
          n343 = Bundle By Name(cluster=w535, "2D Picture"=picture data[5B]) -> (w533:T8)
        }
        n344 = for {
          tunnel: w437 -> [w532] mode=indexing
          tunnel: [w530] -> w409 mode=indexing
          n345 = Bundle By Name(cluster=w532, "2D Picture"=picture data[5B]) -> (w530:T8)
        }
        n346 = for {
          tunnel: w438 -> [w529] mode=indexing
          tunnel: [w527] -> w411 mode=indexing
          n347 = Bundle By Name(cluster=w529, "2D Picture"=picture data[5B]) -> (w527:T8)
        }
        n348 = for {
          tunnel: w439 -> [w526] mode=indexing
          tunnel: [w524] -> w413 mode=indexing
          n349 = Bundle By Name(cluster=w526, "2D Picture"=picture data[5B]) -> (w524:T8)
        }
        n350 = for {
          tunnel: w440 -> [w523] mode=indexing
          tunnel: [w521] -> w415 mode=indexing
          n351 = Bundle By Name(cluster=w523, "2D Picture"=picture data[5B]) -> (w521:T8)
        }
        n352 = for {
          tunnel: w441 -> [w520] mode=indexing
          tunnel: [w518] -> w417 mode=indexing
          n353 = Bundle By Name(cluster=w520, "2D Picture"=picture data[5B]) -> (w518:T8)
        }
        n354 = call <vilib>:"DB Tools Close Connection.vi"("error in (no error)"=w488, "connection reference"=w489) -> ()  [unwired: 5 in, 1 out]
        n355 = case shown="No Error" w419 {
          tunnel: [w517 _] -> w418
          tunnel: w417 -> [w517 _]
          tunnel: [w516 _] -> w416
          tunnel: w415 -> [w516 _]
          tunnel: [w515 _] -> w414
          tunnel: w413 -> [w515 _]
          tunnel: [w514 _] -> w412
          tunnel: w411 -> [w514 _]
          tunnel: [w513 _] -> w410
          tunnel: w409 -> [w513 _]
          tunnel: [w512 _] -> w408
          tunnel: w407 -> [w512 _]
          frame No Error {
          }
          frame Error {
          }
        }
        n356 = local write "Array Grafici ROTBLOCC"(w416) -> ()
        n357 = local write "Array Grafici GENERICA"(w418) -> ()
        n358 = local write "Array Grafici A CARICO"(w410) -> ()
        n359 = local write "Array Grafici A VUOTO"(w408) -> ()
        n360 = local write "Array Grafici TERMICA"(w412) -> ()
        n361 = local write "Array Grafici CMECC"(w414) -> ()
      }
      frame "Carica scelte grafici" {
        n362 = control-ref of="scelta grafico A VUOTO"() -> (w697:refnum<vi>)
        n363 = control-ref of="scelta grafico A CARICO"() -> (w696:refnum<vi>)
        n364 = control-ref of="scelta grafico TERMICA"() -> (w695:refnum<vi>)
        n365 = control-ref of="scelta grafico CMECC"() -> (w694:refnum<vi>)
        n366 = control-ref of="scelta grafico ROTORE BLOCC"() -> (w693:refnum<vi>)
        n367 = control-ref of="scelta grafico GENERICA"() -> (w692:refnum<vi>)
        n368 = control-ref of="scelta grafico SCORTA 1"() -> (w691:refnum<vi>)
        n369 = control-ref of="scelta grafico SCORTA 2"() -> (w690:refnum<vi>)
        n370 = control-ref of="scelta grafico SCORTA 3"() -> (w689:refnum<vi>)
        n371 = Build Array(w697, w696, w695, w694, w693, w692, w691, w690, w689) -> (w698:refnum<vi>[])
        n372 = for {
          tunnel: w698 -> [w706] mode=indexing
          i -> [w705]
          n373 = local read "Grafici"() -> (w707:T5[])
          n374 = for {
            tunnel: w707 -> [w722] mode=indexing
            tunnel: [w711] -> w708 mode=indexing if=w710
            tunnel: w705 -> [w709]
            n375 = Unbundle By Name(w722) -> ("NOME GRAFICO"=w711:string, "PROVE ASSOCIATE.A VUOTO"=w721:bool, "PROVE ASSOCIATE.A CARICO"=w720:bool, "PROVE ASSOCIATE.TERMICA"=w719:bool, "PROVE ASSOCIATE.C.MECC."=w718:bool, "PROVE ASSOCIATE.ROT BLOCC"=w717:bool, "PROVE ASSOCIATE.GENERICA"=w716:bool, "PROVE ASSOCIATE.TABELLA RESISTOMAT"=w715:bool, "PROVE ASSOCIATE.SCORTA 2"=w714:bool, "PROVE ASSOCIATE.SCORTA 3"=w713:bool)  [unwired: 1 out]
            n376 = Build Array(w721, w720, w719, w718, w717, w716, w715, w714, w713) -> (w712:bool[])
            n377 = Index Array(array=w712, index=w709) -> (element=w710:bool)
          }
          n378 = property class="Ring (strict)"(reference=w706, "Strings []"=w708) -> ()  [unwired: 1 in, 2 out]
        }
        n379 = Enqueue Element(queue=w687, element=cluster{"String":string, "variant":variant} {"String"="Aggiungi grafico", "variant"=variant}) -> ()  [unwired: 2 in, 3 out]
      }
      frame "Aggiungi grafico" {
        n380 = local read "COLLAUDI DI CONFRONTO"() -> (w730:string[])
        n381 = local read "Descrizione"() -> (w729:string[])
        n382 = local read "Tab Control"() -> (w743:T7)
        n383 = local read "COLLAUDO PRINCIPALE"() -> (w734:string)
        n384 = control-ref of="scelta grafico A VUOTO"() -> (w760:refnum<vi>)
        n385 = control-ref of="scelta grafico A CARICO"() -> (w768:refnum<vi>)
        n386 = control-ref of="scelta grafico TERMICA"() -> (w767:refnum<vi>)
        n387 = control-ref of="scelta grafico CMECC"() -> (w766:refnum<vi>)
        n388 = control-ref of="scelta grafico ROTORE BLOCC"() -> (w765:refnum<vi>)
        n389 = control-ref of="scelta grafico GENERICA"() -> (w764:refnum<vi>)
        n390 = control-ref of="scelta grafico SCORTA 1"() -> (w763:refnum<vi>)
        n391 = control-ref of="scelta grafico SCORTA 2"() -> (w762:refnum<vi>)
        n392 = control-ref of="scelta grafico SCORTA 3"() -> (w761:refnum<vi>)
        n393 = local read "Descrizione princ"() -> (w733:string)
        n394 = for {
          tunnel: w730 -> [w835] mode=indexing
          tunnel: w729 -> [w837]
          tunnel: [w836] -> w728 mode=indexing
          i -> [w832]
          n395 = Index Array(array=w837, index=w832) -> (element=w833:string)
          n396 = Concatenate Strings(w835, "-" ("string"), w833) -> (w836:string)
        }
        n397 = Decrement(x=w743) -> (x-1=w742:T7)
        n398 = Build Array(w760, w768, w767, w766, w765, w764, w763, w762, w761) -> (w757:refnum<vi>[])
        n399 = local read "modifica"() -> (w726:bool)
        n400 = local read "scelta grafico"() -> (w725:u16)
        n401 = Concatenate Strings(w734, "-" ("string"), w733) -> (w732:string)
        n402 = local read "ID COLLEGAMENTO"() -> (w738:i32)
        n403 = local read "ID Colleg confronti"() -> (w736:i32[])
        n404 = Build Array (concatenate)(w732, w728) -> (w731:string[])
        n405 = Index Array(array=w757, index=w742) -> (element=w754:refnum<vi>)
        n406 = Increment(x=w742) -> (x+1=w753:T7)
        n407 = Select(t=w725, s=w726, f=0) -> (s? t:f=w724:i32)
        n408 = property class="Ring (strict)"(reference=w754) -> ("Strings []"=w740:string[])  [unwired: 1 in, 2 out]
        n409 = Build Array (concatenate)(w738, w736) -> (w737:i32[])
        n410 = local read "Grafici"() -> (w755:T5[])
        n411 = local read "Plots"() -> (w756:T4[])
        n412 = call "Aggiungi grafico.vi"(0:"Grafici"=w755, "Array plot"=w756, 2:"Grafici"=w740, "Grafico default"=w724, "prova"=w753, "ID collegamenti"=w737, "Collaudi"=w731, "Dati collaudo in corso"=w759, "AUTO"=FALSE, "Collaudi di confronto"=w758) -> ("Image Data"=w752:T28, "grafico"=w739:u16, "annulla?"=w723:bool)  [unwired: 5 in, 2 out]
        n413 = control-ref of="Array Grafici A VUOTO"() -> (w741:refnum<vi>)
        n414 = control-ref of="Array Grafici A CARICO"() -> (w749:refnum<vi>)
        n415 = control-ref of="Array Grafici TERMICA"() -> (w748:refnum<vi>)
        n416 = control-ref of="Array Grafici CMECC"() -> (w747:refnum<vi>)
        n417 = control-ref of="Array Grafici ROTBLOCC"() -> (w746:refnum<vi>)
        n418 = control-ref of="Array Grafici GENERICA"() -> (w745:refnum<vi>)
        n419 = Build Array(w741, w749, w748, w747, w746, w745) -> (w750:refnum<vi>[])
        n420 = Index Array(array=w750, index=w742) -> (element=w744:refnum<vi>)
        n421 = case shown="False" w723 {
          tunnel: w752 -> [w805 _]
          tunnel: w744 -> [w783 _]
          tunnel: w740 -> [w778 _]
          tunnel: w739 -> [w777 _]
          frame False {
            w775 = T8 {"2D Picture"=bytes[771184], "Aggiungi grafico"=FALSE, "Settings grafico"=FALSE, "Elimina grafico"=FALSE, "scelta grafico A VUOTO 2"=0, "Esporta xls"={"Esporta?"=TRUE, "Impostazioni esport."={"position (Excel)"={"row"=8, "column"=2}, "Nome foglio (Excel)"="", "bookmark (Word)"=""}, "Zoom "=1.0, "Ruota immagine"=enum."rotate 0°"}} ("Cluster")
            n422 = call "Empty Picture"() -> ("empty picture"=w808:picture)
            n423 = property class="Arr"(reference=w783) -> (reference out=w774:refnum<vi>, "Value"=w807:variant)  [unwired: 1 in, 1 out]
            n424 = local read "modifica"() -> (w773:bool)
            n425 = call <vilib>:"Draw Flattened Pixmap.vi"("image data"=w805, "picture"=w808) -> ("new picture"=w804:picture)  [unwired: 7 in]
            n426 = Build Array(w775) -> (w776:T8[])
            n427 = Variant To Data(type=w776, Variant=w807) -> (data=w785:T8[])  [unwired: 1 in, 1 out]
            n428 = case shown="True" w773 {
              tunnel: w804 -> [w823 w827]
              tunnel: [w821 w828] -> w803
              tunnel: w785 -> [w820 w829]
              tunnel: [w817 w825] -> w784
              tunnel: w777 -> [w816 w826]
              tunnel: w775 -> [w815 _]
              frame False {
                n429 = Array Size(array=w820) -> (size(s)=w818:i32)
                n430 = Decrement(x=w818) -> (x-1=w817:i32)
                n431 = Bundle By Name(cluster=w815, "2D Picture"=w823, "scelta grafico A VUOTO 2"=w816) -> (w822:T8)
                n432 = Delete From Array "Delete From Array"(array=w820, index=w817) -> (array with subset deleted=w819:T8[])  [unwired: 1 in, 1 out]
                n433 = Build Array (concatenate)(w819, w822) -> (w821:T8[])
              }
              frame True {
                n434 = local read "Numeric 2"() -> (w825:i32)
                n435 = Index Array "Index Array"(array=w829, index=w825) -> (element=w830:T8)
                n436 = Bundle By Name(cluster=w830, "2D Picture"=w827, "scelta grafico A VUOTO 2"=w826) -> (w831:T8)
                n437 = local write "modifica"(FALSE) -> ()
                n438 = Replace Array Subset "Replace Array Subset"(array=w829, new element=w831, index=w825) -> (w828:T8[])
              }
            }
            n439 = property class="Arr"(reference=w774, "Value"=w803) -> (reference out=w806:refnum<vi>)  [unwired: 1 in, 1 out]
            n440 = disable-structure shown="Enabled" {
              disable-tunnel: w806 -> [w811 w814]
              disable-tunnel: [w810 w813] -> w795
              disable-tunnel: w784 -> [w809 _]
              frame Disabled {
                n441 = Build Array(w809) -> (w812:i32[])
                n442 = property class="Arr"(reference=w811, "Index Values"=w812) -> ("Array Element"=w810:refnum<vi>)  [unwired: 1 in, 2 out]
              }
              frame Enabled {
                n443 = property class="Arr"(reference=w814) -> ("Array Element"=w813:refnum<vi>)  [unwired: 1 in, 2 out]
              }
            }
            n444 = control-ref of="Cluster"() -> (w802:refnum<vi>)
            n445 = To More Specific Class(target class=w802, reference=w795) -> (specific class reference=w801:refnum<vi>)  [unwired: 1 in, 1 out]
            n446 = property class="Clust"(reference=w801) -> ("Controls[]"=w800:refnum<vi>[])  [unwired: 1 in, 2 out]
            n447 = control-ref of="scelta grafico A VUOTO 2"() -> (w780:refnum<vi>)
            n448 = control-ref of="2D Picture"() -> (w797:refnum<vi>)
            n449 = Index Array(array=w800, index #1=0 ("index"), index #2=4 ("index")) -> (element #1=w798:refnum<vi>, element #2=w781:refnum<vi>)
            n450 = To More Specific Class(target class=w797, reference=w798) -> (specific class reference=w796:refnum<vi>)  [unwired: 1 in, 1 out]
            n451 = To More Specific Class(target class=w780, reference=w781) -> (specific class reference=w779:refnum<vi>)  [unwired: 1 in, 1 out]
            n452 = property class="Pict"(reference=w796) -> (reference out=w787:refnum<vi>, "Draw Area Size"=w794:T29)  [unwired: 1 in, 1 out]
            n453 = Unbundle By Name(w805) -> ("Rectangle.right"=w792:i16, "Rectangle.bottom"=w790:i16)
            n454 = property class="Ring (strict)"(reference=w779, "Strings []"=w778, "Value"=w777) -> ()  [unwired: 1 in, 2 out]
            n455 = Unbundle By Name(w794) -> ("Width"=w793:u32, "Height"=w791:u32)
            n456 = Divide(x=w791, y=w790) -> (x/y=w788:dbl)
            n457 = Divide(x=w793, y=w792) -> (x/y=w789:dbl)
            n458 = Max & Min(x=w789, y=w788) -> (min(x,y)=w786:dbl)  [unwired: 1 out]
            n459 = property class="Pict"(reference=w787, "ZoomFactor"=w786) -> ()  [unwired: 1 in, 2 out]
          }
          frame True {
          }
        }
      }
      frame "AGGIORNA IMMAGINI" {
        n460 = local read "COLLAUDI DI CONFRONTO"() -> (w848:string[])
        n461 = local read "Descrizione"() -> (w847:string[])
        n462 = local read "COLLAUDO PRINCIPALE"() -> (w851:string)
        n463 = control-ref of="Array Grafici A CARICO"() -> (w859:refnum<vi>)
        n464 = control-ref of="Array Grafici TERMICA"() -> (w858:refnum<vi>)
        n465 = control-ref of="Array Grafici CMECC"() -> (w857:refnum<vi>)
        n466 = control-ref of="Array Grafici ROTBLOCC"() -> (w856:refnum<vi>)
        n467 = control-ref of="Array Grafici GENERICA"() -> (w855:refnum<vi>)
        n468 = control-ref of="Array Grafici A VUOTO"() -> (w860:refnum<vi>)
        n469 = control-ref of="scelta grafico A VUOTO"() -> (w862:refnum<vi>)
        n470 = control-ref of="scelta grafico A CARICO"() -> (w870:refnum<vi>)
        n471 = control-ref of="scelta grafico TERMICA"() -> (w869:refnum<vi>)
        n472 = control-ref of="scelta grafico CMECC"() -> (w868:refnum<vi>)
        n473 = control-ref of="scelta grafico ROTORE BLOCC"() -> (w867:refnum<vi>)
        n474 = control-ref of="scelta grafico GENERICA"() -> (w866:refnum<vi>)
        n475 = control-ref of="scelta grafico SCORTA 1"() -> (w865:refnum<vi>)
        n476 = control-ref of="scelta grafico SCORTA 2"() -> (w864:refnum<vi>)
        n477 = control-ref of="scelta grafico SCORTA 3"() -> (w863:refnum<vi>)
        n478 = local read "Descrizione princ"() -> (w852:string)
        n479 = for {
          tunnel: w848 -> [w880] mode=indexing
          tunnel: w847 -> [w882]
          tunnel: [w881] -> w846 mode=indexing
          i -> [w877]
          n480 = Index Array(array=w882, index=w877) -> (element=w878:string)
          n481 = Concatenate Strings(w880, "-" ("string"), w878) -> (w881:string)
        }
        n482 = control-ref of="This VI"() -> (w845:refnum<vi>)
        n483 = Build Array(w860, w859, w858, w857, w856, w855) -> (w854:refnum<vi>[])
        n484 = Build Array(w862, w870, w869, w868, w867, w866, w865, w864, w863) -> (w861:refnum<vi>[])
        n485 = property class="VI"(reference=w845) -> ("Panel"=w844:refnum<vi>)  [unwired: 1 in, 2 out]
        n486 = Concatenate Strings(w851, "-" ("string"), w852) -> (w853:string)
        n487 = property class="Pnl"(reference=w844, "DeferPanUpdts"=TRUE ("Defer Panel Updates")) -> (reference out=w842:refnum<vi>, error out=w841:errorcluster)  [unwired: 1 in]
        n488 = Build Array (concatenate)(w853, w846) -> (w849:string[])
        n489 = for {
          tunnel: w854 -> [w896] mode=indexing
          tunnel: w872 -> [w893]
          tunnel: w871 -> [w892]
          tunnel: w861 -> [w888] mode=indexing
          tunnel: w849 -> [w885]
          tunnel: w842 -> [w884]
          tunnel: [w884] -> w839
          tunnel: w841 -> [w883]
          tunnel: [w883] -> w838
          i -> [w889]
          n490 = property class="Ring (strict)"(reference=w888) -> ("Strings []"=w887:string[])  [unwired: 1 in, 2 out]
          n491 = property class="Arr"(reference=w896) -> (reference out=w890:refnum<vi>, "Value"=w895:variant)  [unwired: 1 in, 1 out]
          n492 = Variant To Data(type=T8[] [] ("Array Grafici A VUOTO"), Variant=w895) -> (data=w894:T8[])  [unwired: 1 in, 1 out]
          n493 = for {
            tunnel: w894 -> [w909] mode=indexing
            tunnel: w893 -> [w911]
            tunnel: w892 -> [w904]
            tunnel: [w905] -> w891 mode=indexing
            tunnel: w889 -> [w902]
            tunnel: w887 -> [w901]
            tunnel: w885 -> [w897]
            n494 = Unbundle By Name(w909) -> ("scelta grafico A VUOTO 2"=w910:u16)
            n495 = local read "ID COLLEGAMENTO"() -> (w900:i32)
            n496 = local read "ID Colleg confronti"() -> (w898:i32[])
            n497 = Increment(x=w902) -> (x+1=w903:i32)
            n498 = Build Array (concatenate)(w900, w898) -> (w899:i32[])
            n499 = local read "Grafici"() -> (w913:T5[])
            n500 = local read "Plots"() -> (w912:T4[])
            n501 = call "Aggiungi grafico.vi"(0:"Grafici"=w913, "Array plot"=w912, 2:"Grafici"=w901, "Grafico default"=w910, "prova"=w903, "ID collegamenti"=w899, "Collaudi"=w897, "Dati collaudo in corso"=w904, "AUTO"=TRUE, "Collaudi di confronto"=w911) -> ("Image Data"=w907:T28)  [unwired: 5 in, 4 out]
            n502 = call "Empty Picture"() -> ("empty picture"=w908:picture)
            n503 = call <vilib>:"Draw Flattened Pixmap.vi"("image data"=w907, "picture"=w908) -> ("new picture"=w906:picture)  [unwired: 7 in]
            n504 = Bundle By Name(cluster=w909, "2D Picture"=w906) -> (w905:T8)
          }
          n505 = property class="Arr"(reference=w890, "Value"=w891) -> ()  [unwired: 1 in, 2 out]
        }
        n506 = property class="Pnl"(reference=w839, error in=w838, "DeferPanUpdts"=FALSE ("Defer Panel Updates")) -> ()  [unwired: 2 out]
      }
      frame "REPORT C2K" {
        n507 = property on="Criteri di salvataggio report" class="MCListbox (strict)"() -> ("ItemNames"=w918:string[][])  [unwired: 2 in, 2 out]
        n508 = property on="Percorso e nome di DEFAULT" class="MCListbox (strict)"() -> ("ItemNames"=w917:string[][])  [unwired: 2 in, 2 out]
        n509 = call "Percorso e nome report.vi"("Default"=w917, "Criteri"=w918) -> ("path Standard"=w921:path, "Nome file"=w922:string)  [unwired: 7 in, 1 out]
        n510 = call "File Dialog"("start path"=w921, "default name"=w922, "pattern (all files)"="*.xls" ("DNL")) -> ("selected path"=w915:path, "cancelled"=w916:bool, "error out"=w919:errorcluster)  [unwired: 4 in, 6 out]
        n511 = call <vilib>:"Clear Errors.vi"("error in (no error)"=w919) -> ()  [unwired: 5 in, 2 out]
        n512 = case shown="False" w916 {
          tunnel: w925 -> [w946 _]
          tunnel: w923 -> [w933 _]
          tunnel: w915 -> [w929 _]
          frame False {
            w945 = string[] [" "] ("element")
            n513 = call "Ora sotto data.vi"("Array in"=w933) -> ("Array out"=w932:string[][])  [unwired: 10 in]
            n514 = local read "ETICHETTE"() -> (w934:string[])
            n515 = Unbundle By Name(w946) -> ("Res freddo res meter"=w944:string[][], "A vuoto"=w943:string[][], "A carico"=w942:string[][], "Termica"=w941:string[][], "Cmecc"=w940:string[][], "Rbloccato"=w939:string[][], "Generica"=w938:string[][])
            n516 = local read "Percorso modelli xls"() -> (w935:path)
            n517 = Build Array (concatenate)(w934, w945, w945, w932, w944, w943, w942, w941, w940, w939, w938) -> (w937:string[][])
            n518 = local read "sep. decimale numeri esportati"() -> (w936:enum16{"Virgola", "Punto"})
            n519 = Build Path(base path=w935, name or relative path="C2K.xls") -> (appended path=w930:path)
            n520 = case shown="\"Punto\"" w936 {
              tunnel: w937 -> [w961 w969]
              tunnel: [w960 w968] -> w947
              frame "Virgola", Default {
                n521 = for {
                  tunnel: w961 -> [w963] mode=indexing
                  tunnel: [w962] -> w960 mode=indexing
                  n522 = for {
                    tunnel: w963 -> [w967] mode=indexing
                    tunnel: [w964] -> w962 mode=indexing
                    n523 = Search and Replace String(input string=w967, search string=",", replace string="." ("search string")) -> (result string=w964:string)  [unwired: 5 in, 3 out]
                  }
                }
              }
              frame "Punto" {
                n524 = for {
                  tunnel: w969 -> [w971] mode=indexing
                  tunnel: [w970] -> w968 mode=indexing
                  n525 = for {
                    tunnel: w971 -> [w975] mode=indexing
                    tunnel: [w972] -> w970 mode=indexing
                    n526 = Search and Replace String(input string=w975, search string=".", replace string="," ("search string")) -> (result string=w972:string)  [unwired: 5 in, 3 out]
                  }
                }
              }
            }
            n527 = call <vilib>:"New Report.vi"("window state (normal)"=T23."no change", "report type"=T24."Excel", "template (empty)"=w930) -> ("report out"=w956:refnum<class "NI_report.lvclass">, "error out"=w957:errorcluster)  [unwired: 11 in]
            n528 = call <vilib>:"Excel Get Worksheet.vi"("report in"=w956, "error in (no error)"=w957, "name (\"\")"="Dati_nascosti" ("name (\"\")")) -> ("report out"=w955:refnum<class "NI_report.lvclass">, "error out"=w953:errorcluster)  [unwired: 11 in]
            n529 = call-poly <vilib>:"Excel Easy Table.vi"("report in"=w955, "text data"=w947, "error in (no error)"=w953) -> ("report out"=w951:refnum<class "NI_report.lvclass">, "error out"=w952:errorcluster)  [unwired: 8 in, 3 out]
            n530 = call-dynamic "Save Report to File.vi"("report in"=w951, "report file path"=w929, "prompt to replace? (F)"=TRUE, "error in (no error)"=w952) -> ("report out"=w948:refnum<class "NI_report.lvclass">, "error out"=w949:errorcluster)  [unwired: 10 in]
            n531 = call-dynamic "Dispose Report.vi"("report in"=w948, "error in (no error)"=w949) -> ()  [unwired: 13 in, 1 out]
          }
          frame True {
          }
        }
      }
      frame "Aggiorna tabelle" {
        n532 = flat-sequence {
          tunnel: w983 -> [w994]
          tunnel: [w994] -> w979
          tunnel: [w989] -> w976
          tunnel: w979 -> [w996]
          tunnel: [w997] -> w978
          tunnel: [w1002] -> w977
          tunnel: w976 -> [w1002]
          tunnel: [w1056] -> w982
          tunnel: w978 -> [w1056]
          tunnel: w977 -> [w1053]
          frame #0 {
            n533 = control-ref of="This VI"() -> (w990:refnum<vi>)
            n534 = property class="VI"(reference=w990) -> ("Panel"=w991:refnum<vi>)  [unwired: 1 in, 2 out]
            n535 = property class="Pnl"(reference=w991, "DeferPanUpdts"=TRUE ("Defer Panel Updates")) -> (reference out=w989:refnum<vi>)  [unwired: 1 in, 1 out]
            "Boolean" <- TRUE
          }
          frame #1 {
            w1006 = i16 1  # TABELLE SCORTA
            n536 = control-ref of="TABELLA RES FREDDO RES METER"() -> (w1012:refnum<vi>)
            n537 = control-ref of="TABELLA RES FREDDO RESISTOMAT"() -> (w1013:refnum<vi>)
            n538 = control-ref of="TABELLA A VUOTO"() -> (w1029:refnum<vi>)
            n539 = control-ref of="TABELLA A CARICO"() -> (w1028:refnum<vi>)
            n540 = control-ref of="TABELLA TERMICA"() -> (w1027:refnum<vi>)
            n541 = control-ref of="TABELLA C MECC"() -> (w1026:refnum<vi>)
            n542 = control-ref of="TABELLA ROT BLOCC"() -> (w1025:refnum<vi>)
            n543 = control-ref of="TABELLA GENERICA"() -> (w1021:refnum<vi>)
            n544 = control-ref of="TABELLA RES TERMICA"() -> (w1024:refnum<vi>)
            n545 = control-ref of="TABELLA SCORTA 2"() -> (w1023:refnum<vi>)
            n546 = control-ref of="TABELLA SCORTA 3"() -> (w1022:refnum<vi>)
            n547 = control-ref of="TABELLA EQ TERMICO"() -> (w1020:refnum<vi>)
            n548 = control-ref of="TABELLA COPPIA MAX"() -> (w1019:refnum<vi>)
            n549 = control-ref of="TABELLA I SPUNTO"() -> (w1018:refnum<vi>)
            n550 = control-ref of="Res INIZIO prova VUOTO"() -> (w1017:refnum<vi>)
            n551 = control-ref of="Res FINE prova VUOTO"() -> (w1016:refnum<vi>)
            n552 = control-ref of="Res INIZIO prova CARICO"() -> (w1015:refnum<vi>)
            n553 = control-ref of="Res FINE prova CARICO"() -> (w1014:refnum<vi>)
            n554 = local read "ID COLLEGAMENTO"() -> (w1003:i32)
            n555 = Build Array(w1012, w1013, w1029, w1028, w1027, w1026, w1025, w1021, w1024, w1023, w1022, w1020, w1019, w1018, w1017, w1016, w1015, w1014) -> (w1004:refnum<vi>[])
            n556 = Build Array("TABELLA TERMICA", "TABELLA TERMICA", "TABELLA A VUOTO", "TABELLA A CARICO", "TABELLA TERMICA", "TABELLA CMECC", "TABELLA A ROT BLOCC", "TABELLA GENERICA", "TABELLA TERMICA", w1006, w1006, "TABELLA TERMICA", "TABELLA CMECC", "TABELLA A ROT BLOCC", "TABELLA A VUOTO", "TABELLA A VUOTO", "TABELLA A CARICO", "TABELLA A CARICO") -> (w998:i16[])
            n557 = Unbundle By Name(w996) -> ()  [unwired: 1 out]
            n558 = disable-structure shown="Enabled" {
              disable-tunnel: [w1032 w1037] -> w1005
              disable-tunnel: w1004 -> [w1031 w1037]
              disable-tunnel: w1003 -> [w1030 _]
              frame Disabled {
                n559 = call "Leggi filtro ed etichette.vi"("ID COLLEGAMENTO"=w1030) -> ("ETICHETTE"=w1033:string[])  [unwired: 5 in, 5 out]
                n560 = for {
                  tunnel: w1031 -> [w1036] mode=indexing
                  tunnel: w1033 -> [w1035]
                  tunnel: [w1034] -> w1032 mode=indexing
                  n561 = property on="Property Node" class="MCListbox (strict)"(reference=w1036, "ColHdrString"=w1035) -> (reference out=w1034:refnum<vi>)  [unwired: 1 in, 1 out]
                }
              }
              frame Enabled {
              }
            }
            n562 = call "Nascondi colonne.vi"("TIPO COLLEGAMENTO"=w1003, "Array"=w1004) -> ()  [unwired: 9 in, 1 out]
            n563 = for {
              tunnel: w1005 -> [w1043] mode=indexing
              shift-right: [w1049] -> w997
              shift-left: w996 -> [w1046]
              tunnel: w998 -> [w1041] mode=indexing
              tunnel: w1003 -> [w1040]
              i -> [w1042]
              n564 = Number To Decimal String(number=w1042) -> (decimal integer string=w1047:string)  [unwired: 1 in]
              n565 = call "carica dati prove.vi"("TIPO COLLEGAMENTO"=w1040, "Carica tabelle?"=TRUE, "Tabella"=w1041, "prova"=w1047, "Dati prove in"=w1046) -> ("Per tabella"=w1039:string[][], "Dati prove out"=w1049:T27)  [unwired: 4 in, 1 out]
              n566 = Empty Array?(array=w1039) -> (empty?=w1038:bool)
              n567 = property class="MCListbox (strict)"(reference=w1043, "ItemNames"=w1039) -> (reference out=w1045:refnum<vi>, error out=w1044:errorcluster)  [unwired: 1 in]
              n568 = case shown="True" w1038 {
                tunnel: w1045 -> [w1052 _]
                tunnel: w1044 -> [w1051 _]
                frame False {
                  n569 = call "Auto width colum table.vi"("error in (no error)"=w1051, "spazi"=i16 10, "Real Time tabella"=w1052) -> ()  [unwired: 8 in, 1 out]
                }
                frame True {
                }
              }
            }
            n570 = call "calcolo rendimento.vi"("DETERMINAZIONE DEL RENDIMENTO Item Names"=string[][] [["Potenza resa nominale corretta", "%", "125%", "115%", "100%", "75%", "50%", "25%"], ["Scorrimento corretto", "p.u.", "", "", "", "", "", ""], ["Potenza assorbita corretta", "W", "", "", "", "", "", ""], ["Perdite nel ferro", "W", "", "", "", "", "", ""], ["Perdite di ventilazione e attrito corrette", "W", "", "", "", "", "", ""], ["Perdite addizionali a carico", "W", "", "", "", "", "", ""], ["Perdite nello statore corrette", "W", "", "", "", "", "", ""], ["Perdite nel rotore corrette", "W", "", "", "", "", "", ""], ["RENDIMENTO", "%", "", "", "", "", "", ""]] ("Item Names"), "Dati prove"=w997, "TABELLE"=w998) -> ("Coeff correlaz"=→"Coefficiente di correlazione":dbl, "DETERMINAZIONE DEL RENDIMENTO"=w1001:string[][])  [unwired: 8 in, 7 out]
            n571 = property on="DETERMINAZIONE DEL RENDIMENTO" class="MCListbox (strict)"("ItemNames"=w1001) -> ()  [unwired: 2 in, 2 out]
          }
          frame #2 {
            n572 = property class="Pnl"(reference=w1053, "DeferPanUpdts"=FALSE ("Defer Panel Updates")) -> ()  [unwired: 1 in, 2 out]
            n573 = local write "Boolean"(FALSE ("Boolean")) -> ()
          }
        }
        n574 = Enqueue Element(queue=w980, element=cluster{"String":string, "variant":variant} {"String"="AGGIORNA IMMAGINI", "variant"=variant}) -> ()  [unwired: 2 in, 3 out]
      }
      frame "SALVA COME DEFAULT" {
        (unwired) "::" ("delimiter (\\t)")
        (unwired) "::" ("delimiter (\\t)")
        n575 = local read "Stili grafico"() -> (w1089:T10)
        n576 = local read "colori grafici"() -> (w1084:T11)
        n577 = Unbundle By Name(w1089) -> ("Stile grafici Tabella 1"=w1088:T30, "Stile grafici Tabella 2"=w1087:T30, "Stile grafici Tabella 3"=w1086:T30, "Stile croci"=w1085:T31)  [unwired: 6 out]
        n578 = Unbundle By Name(w1084) -> ()  [unwired: 3 out]
        n579 = Boolean To (0,1)(Boolean="EXCEL 2") -> (0, 1=w1063:i16)
        n580 = Boolean To (0,1)(Boolean="PDF ITA 2") -> (0, 1=w1061:i16)
        n581 = Boolean To (0,1)(Boolean="PDF INGL 2") -> (0, 1=w1059:i16)
        n582 = local read "sep. decimale numeri esportati"() -> (w1057:enum16{"Virgola", "Punto"})
        n583 = Unbundle By Name(w1085) -> ()  [unwired: 4 out]
        n584 = Unbundle By Name(w1088) -> ()  [unwired: 3 out]
        n585 = Unbundle By Name(w1087) -> ()  [unwired: 3 out]
        n586 = Unbundle By Name(w1086) -> ()  [unwired: 3 out]
        n587 = local read "Percorso report di DEFAULT"() -> (w1081:path)
        n588 = local read "Percorso report di DEFAULT"() -> (w1091:path)
        n589 = local read "Percorso report di DEFAULT"() -> (w1092:path)
        n590 = local read "Percorso modelli xls"() -> (w1082:path)
        n591 = local read "Percorso modelli xls"() -> (w1090:path)
        n592 = local read "Percorso modelli xls"() -> (w1093:path)
        n593 = Path To String(path=w1082) -> (string=w1078:string)
        n594 = Path To String(path=w1090) -> ()  [unwired: 1 out]
        n595 = Path To String(path=w1093) -> ()  [unwired: 1 out]
        n596 = Path To String(path=w1081) -> (string=w1079:string)
        n597 = Path To String(path=w1091) -> ()  [unwired: 1 out]
        n598 = Path To String(path=w1092) -> ()  [unwired: 1 out]
        n599 = Build Array(w1057, w1063, "Foglio attivo xls", w1061, "Foglio attivo pdf ita", w1059, "Foglio attivo pdf eng") -> (w1083:u16[])
        n600 = global read "Global percorso impostazioni.vi" "Path settings"() -> (w1067:path)
        n601 = property on="Percorso e nome di DEFAULT" class="MCListbox (strict)"() -> ("ItemNames"=w1073:string[][])  [unwired: 2 in, 2 out]
        n602 = property on="Criteri di salvataggio report" class="MCListbox (strict)"() -> ("ItemNames"=w1072:string[][])  [unwired: 2 in, 2 out]
        n603 = Number To Fractional String(number=w1083) -> (F-format string=w1080:string[])  [unwired: 3 in]
        n604 = Build Array (concatenate)(w1078, w1079, w1080) -> (w1077:string[])
        n605 = Build Path(base path=w1067, name or relative path="Report\\Settings\\Criteri_Salvataggio.txt") -> (appended path=w1069:path)
        n606 = Build Path(base path=w1067, name or relative path="Report\\Settings\\Default_ReportManager.txt") -> (appended path=w1074:path)
        n607 = Build Array (concatenate)(w1073, w1072) -> (w1068:string[][])
        n608 = call-poly <vilib>:"Write Delimited Spreadsheet.vi"("file path (dialog if empty)"=w1069, "2D data"=w1068, "delimiter (\\t)"="::" ("delimiter (\\t)")) -> ()  [unwired: 11 in, 2 out]
        n609 = call-poly <vilib>:"Write Delimited Spreadsheet.vi"("file path (dialog if empty)"=w1074, "1D data"=w1077, "delimiter (\\t)"="::" ("delimiter (\\t)")) -> ()  [unwired: 11 in, 2 out]
      }
      frame "SALVA IMP ESPORTAZIONE" {
        n610 = property on="SCEGLI MODELLO" class="CmbBox"() -> ("Text.Text"=w1103:string)  [unwired: 2 in, 2 out]
        n611 = Search and Replace String(input string=w1103, search string=".", replace string="_" ("replace string (\"\")")) -> (result string=w1100:string)  [unwired: 5 in, 3 out]
        n612 = Concatenate Strings("Settings grafici\\IMPOSTAZIONI_ESPORTAZIONE_" ("name or relative path"), w1100) -> (w1104:string)
        n613 = global read "Global percorso impostazioni.vi" "Path settings"() -> (w1113:path)
        n614 = local read "Nome fogli"() -> (w1108:T13)
        n615 = local read "Nome fogli GENERICHE"() -> (w1107:T12)
        n616 = Build Path(base path=w1113, name or relative path=w1104) -> (appended path=w1114:path)
        n617 = Open/Create/Replace File(file path (use dialog)=w1114, operation (0:open)=T14."replace or create with confirmation") -> (refnum out=w1112:refnum<file>, error out=w1111:errorcluster)  [unwired: 4 in, 1 out]
        n618 = Bundle("Nome fogli"=w1108, "Nome fogli GENERICHE"=w1107) -> (w1106:T20)  [unwired: 1 in]
        n619 = Write to Binary File(file (use dialog)=w1112, data=w1106, error in=w1111) -> (refnum out=w1109:refnum<file>, error out=w1110:errorcluster)  [unwired: 3 in, 1 out]
        n620 = Close File(refnum=w1109, error in=w1110) -> ()  [unwired: 2 out]
      }
      frame "CARICA DEFAULT" {
        n621 = Enqueue Element(queue=w1158, element=cluster{"String":string, "variant":variant} {"String"="Initialize", "variant"=variant}) -> ()  [unwired: 2 in, 3 out]
        n622 = global read "Global percorso impostazioni.vi" "Path settings"() -> (w1134:path)
        n623 = Build Path(base path=w1134, name or relative path="Report\\Settings\\Default_ReportManager.txt") -> (appended path=w1137:path)
        n624 = call-poly <vilib>:"Read Delimited Spreadsheet.vi"("file path (dialog if empty)"=w1137, "delimiter (\\t)"="::" ("delimiter (\\t)")) -> ("first row"=w1143:string[], "error out"=w1135:errorcluster)  [unwired: 8 in, 4 out]
        n625 = Array Subset(array=w1143, index=2) -> (w1133:string[])  [unwired: 1 in]
        n626 = Index Array(array=w1143) -> (element #1=w1139:string, element #2=w1141:string)  [unwired: 2 in]
        n627 = for {
          tunnel: w1133 -> [w1165] mode=indexing
          tunnel: [w1164] -> w1132 mode=indexing
          n628 = call "String To Dbl.vi"("String"=w1165) -> ("Numeric"=w1164:dbl)  [unwired: 10 in]
        }
        n629 = String To Path(string=w1139) -> (path=w1140:path)
        n630 = String To Path(string=w1141) -> (path=w1142:path)
        n631 = local write "Percorso report di DEFAULT"(w1142) -> ()
        n632 = Index Array(array=w1132) -> (element #1=w1122:dbl, element #2=w1131:dbl, element #3=w1130:dbl, element #4=w1129:dbl, element #5=w1128:dbl, element #6=w1127:dbl, element #7=w1126:dbl)  [unwired: 7 in]
        n633 = local write "Percorso modelli xls"(w1140) -> ()
        n634 = flat-sequence {
          tunnel: w1135 -> [_]
          frame #0 {
            n635 = Wait (ms)(milliseconds to wait=u32 500) -> ()  [unwired: 1 out]
          }
        }
        n636 = Not Equal To 0?(x=w1131) -> (x != 0?=w1125:bool)
        n637 = Not Equal To 0?(x=w1129) -> (x != 0?=w1124:bool)
        n638 = Not Equal To 0?(x=w1127) -> (x != 0?=w1123:bool)
        n639 = local write "sep. decimale numeri esportati"(w1122) -> ()
        n640 = local write "EXCEL 2"(w1125) -> ()
        n641 = local write "Foglio attivo xls"(w1130) -> ()
        n642 = local write "PDF ITA 2"(w1124) -> ()
        n643 = local write "Foglio attivo pdf ita"(w1128) -> ()
        n644 = local write "PDF INGL 2"(w1123) -> ()
        n645 = local write "Foglio attivo pdf eng"(w1126) -> ()
        n646 = global read "Global percorso impostazioni.vi" "Path settings"() -> (w1145:path)
        n647 = Build Path(base path=w1145, name or relative path="Report\\Settings\\Criteri_Salvataggio.txt") -> (appended path=w1153:path)
        n648 = call-poly <vilib>:"Read Delimited Spreadsheet.vi"("file path (dialog if empty)"=w1153, "delimiter (\\t)"="::" ("delimiter (\\t)")) -> ("all rows"=w1152:string[][])  [unwired: 8 in, 5 out]
        n649 = Delete From Array(array=w1152, length=1, index (row)=0) -> (deleted portion=w1149:string[][], array with subset deleted=w1148:string[][])  [unwired: 1 in]
        n650 = flat-sequence {
          tunnel: [w1167] -> w1147
          tunnel: w1146 -> [w1167]
          tunnel: w1147 -> [_]
          frame #0 {
            n651 = Wait (ms)(milliseconds to wait=u32 150) -> ()  [unwired: 1 out]
          }
          frame #1 {
            n652 = control-ref of="Percorso e nome di DEFAULT"() -> (w1170:refnum<vi>)
            n653 = control-ref of="Criteri di salvataggio report"() -> (w1169:refnum<vi>)
            n654 = call "Auto width colum table.vi"("spazi"=i16 10, "Real Time tabella"=w1169) -> ()  [unwired: 9 in, 1 out]
            n655 = call "Auto width colum table.vi"("spazi"=i16 10, "Real Time tabella"=w1170) -> ()  [unwired: 9 in, 1 out]
          }
        }
        n656 = property on="Criteri di salvataggio report" class="MCListbox (strict)"("ItemNames"=w1148) -> (error out=w1146:errorcluster)  [unwired: 2 in, 1 out]
        n657 = property on="Percorso e nome di DEFAULT" class="MCListbox (strict)"("ItemNames"=w1149) -> ()  [unwired: 2 in, 2 out]
      }
      frame "Carica collaudi di confronto" {
        n658 = for {
          tunnel: "COLLAUDI DI CONFRONTO" -> [w1186] mode=indexing
          tunnel: [w1186] -> w1175 mode=indexing if=w1184
          n659 = Empty String/Path?(string/path=w1186) -> (empty?=w1185:bool)
          n660 = Not(x=w1185) -> (.not. x?=w1184:bool)
        }
        n661 = for {
          tunnel: w1175 -> [w1194] mode=indexing
          tunnel: [w1193] -> w1183 mode=indexing
          tunnel: w1179 -> [_]
          tunnel: w1178 -> [_]
          tunnel: [w1187] -> w1173 mode=indexing
          w1192 = 6  # INDICE Collegamento
          w1202 = "Bollettini" ("table")
          n662 = call "MDB Reference.vi"("Collaudi T/motori F"=TRUE ("NM?")) -> ("error out"=w1204:errorcluster, "Refnum out"=w1206:T26)  [unwired: 8 in, 1 out]
          n663 = call "load string.vi"("Array in"=string[] ["Banco = '", "' AND Anno =", " AND Numero =", " And Tipo_Prova='", "'"], "Codice"=w1194) -> ("ID bollettino"=w1195:string[], "String command"=w1207:string)  [unwired: 7 in, 1 out]
          n664 = call <vilib>:"DB Tools List Columns.vi"("error in (no error)"=w1204, "table"=w1202, "connection reference"=w1206) -> ("error out"=w1203:errorcluster, "columns"=w1201:string[], "connection reference out"=w1205:T26)  [unwired: 1 in, 1 out]
          n665 = call <vilib>:"DB Tools Select Data.vi"("condition"=w1207, "error in (no error)"=w1203, "table"=w1202, "connection reference"=w1205) -> ("error out"=w1200:errorcluster, "data"=w1209:variant[][], "connection reference out"=w1198:T26)  [unwired: 2 in]
          n666 = xnode "Database Variant To Data"("database variant"=w1209, "type"=string[][] [] ("Item Names")) -> ("data"=w1190:string[][])  [unwired: 1 in, 1 out]
          n667 = call <vilib>:"DB Tools List Columns.vi"("error in (no error)"=w1200, "table"="misure", "connection reference"=w1198) -> ("error out"=w1199:errorcluster, "connection reference out"=w1197:T26)  [unwired: 1 in, 2 out]
          n668 = Index Array(array=w1190, index (row)=0, index (col)=w1192) -> (element=w1188:string)
          n669 = Build Array (concatenate)(w1201, w1190) -> ()  [unwired: 1 out]
          n670 = call "da TIPO a ID.vi"("TIPO"=w1188) -> ("ID"=w1187:i32)  [unwired: 10 in]
          n671 = call "Leggi filtro ed etichette.vi"("ID COLLEGAMENTO"=w1187) -> ("FILTRO"=w1189:bool[])  [unwired: 5 in, 5 out]
          n672 = call "Carica misure.vi"("Filtro 3ph6ch"=w1189, "error in (no error)"=w1199, "ID bollettino"=w1195, "Refnum in"=w1197) -> ("error out"=w1211:errorcluster, "Dati prove out"=w1193:T27, "Refnum out"=w1212:T26)  [unwired: 5 in]
          n673 = call <vilib>:"DB Tools Close Connection.vi"("error in (no error)"=w1211, "connection reference"=w1212) -> ()  [unwired: 5 in, 1 out]
        }
        "ID Colleg confronti" <- w1173
      }
      frame "Carica grafici F", "Carica grafici H" {
        n674 = disable-structure shown="Disabled" {
          disable-tunnel: w1267 -> [w1375 _]
          disable-tunnel: w1266 -> [w1374 _]
          disable-tunnel: [w1336 _] -> w1264
          disable-tunnel: w1263 -> [w1304 _]
          disable-tunnel: w1261 -> [w1277 _]
          disable-tunnel: w1260 -> [w1276 _]
          disable-tunnel: w1259 -> [w1268 _]
          frame Disabled {
            w1285 = u32 1 ("Plot.Y Scale Index")
            w1286 = u32 0 ("Plot.Y Scale Index")
            w1328 = -1
            w1341 = 0 ("index")
            # "nota: se Valore di P2 assente (file di taratura non usato durante il collaudo)\ngrafica Q-p1 e Q-etagruppo"
            n675 = property on="Legenda" class="Clust (strict)"() -> ("Controls[]"=w1310:refnum<vi>[])  [unwired: 2 in, 2 out]
            n676 = Build Array (concatenate)(w1374, w1375) -> (w1308:T27[])
            n677 = for {
              tunnel: w1308 -> [w1376] mode=indexing
              tunnel: [w1382] -> w1299 mode=indexing
              tunnel: [w1381] -> w1298 mode=indexing
              tunnel: [w1380] -> w1296 mode=indexing
              tunnel: [w1379] -> w1294 mode=indexing
              tunnel: [w1378] -> w1293 mode=indexing
              tunnel: [w1377] -> w1292 mode=indexing
              w1383 = string[][] [] ("y")
              n678 = Unbundle By Name(w1376) -> ("Curva 1"=w1389, "Curva 2"=w1388, "Curva 3"=w1387)
              n679 = Unbundle By Name(w1376) -> ("Curva 1"=w1384, "Curva 2"=w1385, "Curva 3"=w1386)
              n680 = Not Equal?(x=w1389, y=w1383) -> (x != y?=w1382:bool)
              n681 = Not Equal?(x=w1388, y=w1383) -> (x != y?=w1378:bool)
              n682 = Not Equal?(x=w1387, y=w1383) -> (x != y?=w1380:bool)
              n683 = Not Equal?(x=w1384, y=w1383) -> (x != y?=w1381:bool)
              n684 = Not Equal?(x=w1385, y=w1383) -> (x != y?=w1377:bool)
              n685 = Not Equal?(x=w1386, y=w1383) -> (x != y?=w1379:bool)
            }
            n686 = local read "trifase?"() -> (w1306:bool)
            n687 = Enqueue Element(queue=w1276, element=cluster{"String":string, "variant":variant} {"String"="Grafica", "variant"=variant}) -> ()  [unwired: 2 in, 3 out]
            n688 = Boolean To (0,1)(Boolean=w1306) -> (0, 1=w1305:i16)
            n689 = for {
              N: 6 -> [_]
              tunnel: w1310 -> [w1401] mode=indexing
              tunnel: [w1399] -> w1309 mode=indexing
              n690 = property class="Ctl"(reference=w1401, "Visible"=FALSE) -> (error out=w1399:errorcluster)  [unwired: 1 in, 1 out]
            }
            n691 = for {
              tunnel: w1308 -> [w1521] mode=indexing
              tunnel: w1304 -> [w1520]
              tunnel: [w1496] -> w1355 mode=indexing
              tunnel: [w1491] -> w1348 mode=indexing if=w1461
              tunnel: [w1490] -> w1351 mode=indexing
              tunnel: w1305 -> [w1486]
              tunnel: [w1470] -> w1290 mode=indexing if=w1469
              tunnel: [w1461] -> w1280
              tunnel: w1268 -> [w1460]
              i -> [w1472]
              w1485 = 17  # rpm mono
              w1471 = T32 {"nomi plot"=[], "plot"=[], "#collaudo"=0} ("output cluster")
              w1489 = 13  # RPM tri
              n692 = case shown="\"Carica grafici H\"" w1460 {
                tunnel: w1521 -> [w1526 w1531]
                tunnel: [w1522 w1530] -> w1473
                tunnel: [w1525 w1529] -> w1468
                tunnel: [w1524 w1528] -> w1464
                tunnel: [w1523 w1527] -> w1463
                frame "Carica grafici F", Default {
                  n693 = Unbundle By Name(w1526) -> ("nome collaudo"=w1522:string, "Curva 1"=w1523, "Curva 2"=w1524, "Curva 3"=w1525)
                }
                frame "Carica grafici H" {
                  n694 = Unbundle By Name(w1531) -> ("nome collaudo"=w1530:string, "Curva 1"=w1527, "Curva 2"=w1528, "Curva 3"=w1529)
                }
              }
              n695 = Index Array(array=w1520, index=w1486) -> (element=w1519:T19)
              n696 = Build Array(w1485, w1489) -> (w1488:i32[])
              n697 = Unbundle By Name(w1519) -> ("Q"=w1467:i32, "Htot"=w1518:i32, "P2"=w1465:i32, "etap"=w1517:i32, "P1"=w1466:i32, "etaGr"=w1478:i32)
              n698 = Index Array(array=w1488, index=w1486) -> (element=w1487:i32)
              n699 = call "GRAFICA CURVA XY.vi"("Y INDEX"=w1518, "X INDEX"=w1467, "Curva 1"=w1463) -> ("Cluster"=w1515:cluster{"X":dbl[], "Y":dbl[]})  [unwired: 8 in]
              n700 = call "GRAFICA CURVA XY.vi"("Y INDEX"=w1518, "X INDEX"=w1467, "Curva 1"=w1464) -> ("Cluster"=w1514:cluster{"X":dbl[], "Y":dbl[]})  [unwired: 8 in]
              n701 = call "GRAFICA CURVA XY.vi"("Y INDEX"=w1518, "X INDEX"=w1467, "Curva 1"=w1468) -> ("Cluster"=w1513:cluster{"X":dbl[], "Y":dbl[]})  [unwired: 8 in]
              n702 = call "GRAFICA CURVA XY.vi"("Y INDEX"=w1487, "X INDEX"=w1467, "Curva 1"=w1463) -> ("Cluster"=w1511:cluster{"X":dbl[], "Y":dbl[]})  [unwired: 8 in]
              n703 = call "GRAFICA CURVA XY.vi"("Y INDEX"=w1487, "X INDEX"=w1467, "Curva 1"=w1464) -> ("Cluster"=w1510:cluster{"X":dbl[], "Y":dbl[]})  [unwired: 8 in]
              n704 = call "GRAFICA CURVA XY.vi"("Y INDEX"=w1487, "X INDEX"=w1467, "Curva 1"=w1468) -> ("Cluster"=w1509:cluster{"X":dbl[], "Y":dbl[]})  [unwired: 8 in]
              n705 = call "GRAFICA CURVA XY.vi"("Y INDEX"=w1465, "X INDEX"=w1467, "Curva 1"=w1463) -> ("Cluster"=w1506:cluster{"X":dbl[], "Y":dbl[]})  [unwired: 8 in]
              n706 = call "GRAFICA CURVA XY.vi"("Y INDEX"=w1465, "X INDEX"=w1467, "Curva 1"=w1464) -> ("Cluster"=w1505:cluster{"X":dbl[], "Y":dbl[]})  [unwired: 8 in]
              n707 = call "GRAFICA CURVA XY.vi"("Y INDEX"=w1465, "X INDEX"=w1467, "Curva 1"=w1468) -> ("Cluster"=w1504:cluster{"X":dbl[], "Y":dbl[]})  [unwired: 8 in]
              n708 = call "GRAFICA CURVA XY.vi"("Y INDEX"=w1517, "X INDEX"=w1467, "Curva 1"=w1463) -> ("Cluster"=w1503:cluster{"X":dbl[], "Y":dbl[]})  [unwired: 8 in]
              n709 = call "GRAFICA CURVA XY.vi"("Y INDEX"=w1517, "X INDEX"=w1467, "Curva 1"=w1464) -> ("Cluster"=w1502:cluster{"X":dbl[], "Y":dbl[]})  [unwired: 8 in]
              n710 = call "GRAFICA CURVA XY.vi"("Y INDEX"=w1517, "X INDEX"=w1467, "Curva 1"=w1468) -> ("Cluster"=w1501:cluster{"X":dbl[], "Y":dbl[]})  [unwired: 8 in]
              n711 = call "GRAFICA CURVA XY.vi"("Y INDEX"=w1466, "X INDEX"=w1467, "Curva 1"=w1463) -> ("Cluster"=w1479:cluster{"X":dbl[], "Y":dbl[]})  [unwired: 8 in]
              n712 = call "GRAFICA CURVA XY.vi"("Y INDEX"=w1466, "X INDEX"=w1467, "Curva 1"=w1464) -> ("Cluster"=w1480:cluster{"X":dbl[], "Y":dbl[]})  [unwired: 8 in]
              n713 = call "GRAFICA CURVA XY.vi"("Y INDEX"=w1466, "X INDEX"=w1467, "Curva 1"=w1468) -> ("Cluster"=w1481:cluster{"X":dbl[], "Y":dbl[]})  [unwired: 8 in]
              n714 = call "GRAFICA CURVA XY.vi"("Y INDEX"=w1478, "X INDEX"=w1467, "Curva 1"=w1463) -> ("Cluster"=w1482:cluster{"X":dbl[], "Y":dbl[]})  [unwired: 8 in]
              n715 = call "GRAFICA CURVA XY.vi"("Y INDEX"=w1478, "X INDEX"=w1467, "Curva 1"=w1464) -> ("Cluster"=w1483:cluster{"X":dbl[], "Y":dbl[]})  [unwired: 8 in]
              n716 = call "GRAFICA CURVA XY.vi"("Y INDEX"=w1478, "X INDEX"=w1467, "Curva 1"=w1468) -> ("Cluster"=w1484:cluster{"X":dbl[], "Y":dbl[]})  [unwired: 8 in]
              n717 = call "File taratura assente.vi"("Curva 3"=w1463, "Curva 2"=w1464, "Curva 1"=w1463, "P2"=w1465) -> ("File taratura assente"=w1462:bool)  [unwired: 7 in]
              n718 = Build Array(w1511, w1510, w1509) -> (w1507:cluster{"X":dbl[], "Y":dbl[]}[])
              n719 = Build Array(w1515, w1514, w1513) -> (w1512:cluster{"X":dbl[], "Y":dbl[]}[])
              n720 = Build Array(w1506, w1505, w1504, w1503, w1502, w1501) -> (w1500:cluster{"X":dbl[], "Y":dbl[]}[])
              n721 = Build Array(w1479, w1480, w1481, w1482, w1483, w1484) -> (w1475:cluster{"X":dbl[], "Y":dbl[]}[])
              n722 = Not(x=w1462) -> (.not. x?=w1461:bool)
              n723 = for {
                tunnel: string[] ["--Tab1--QP1", "--Tab2--QP1", "--Tab3--QP1", "--Tab1--QEtagr", "--Tab2--QEtagr", "--Tab3--QEtagr"] -> [w1537] mode=indexing
                tunnel: w1473 -> [w1536]
                tunnel: [w1535] -> w1476 mode=indexing if=w1532
                tunnel: w1475 -> [w1533] mode=indexing
                tunnel: [w1533] -> w1477 mode=indexing if=w1532
                n724 = Concatenate Strings(w1536, w1537) -> (w1535:string)
                n725 = Not Equal?(x=w1533, y=cluster{"X":dbl[], "Y":dbl[]} {"X"=[], "Y"=[]}) -> (x != y?=w1532:bool)
              }
              n726 = for {
                tunnel: string[] ["--Tab1--QH", "--Tab2--QH", "--Tab3--QH"] -> [w1555] mode=indexing
                tunnel: w1473 -> [w1554]
                tunnel: [w1553] -> w1498 mode=indexing if=w1550
                tunnel: w1512 -> [w1551] mode=indexing
                tunnel: [w1551] -> w1497 mode=indexing if=w1550
                n727 = Concatenate Strings(w1554, w1555) -> (w1553:string)
                n728 = Not Equal?(x=w1551, y=cluster{"X":dbl[], "Y":dbl[]} {"X"=[], "Y"=[]}) -> (x != y?=w1550:bool)
              }
              n729 = for {
                tunnel: string[] ["--Tab1--QRpm", "--Tab2--QRpm", "--Tab3--QRpm"] -> [w1549] mode=indexing
                tunnel: w1473 -> [w1548]
                tunnel: [w1547] -> w1495 mode=indexing if=w1544
                tunnel: w1507 -> [w1545] mode=indexing
                tunnel: [w1545] -> w1494 mode=indexing if=w1544
                n730 = Concatenate Strings(w1548, w1549) -> (w1547:string)
                n731 = Not Equal?(x=w1545, y=cluster{"X":dbl[], "Y":dbl[]} {"X"=[], "Y"=[]}) -> (x != y?=w1544:bool)
              }
              n732 = for {
                tunnel: string[] ["--Tab1--QP2", "--Tab2--QP2", "--Tab3--QP2", "--Tab1--QEtap", "--Tab2--QEtap", "--Tab3--QEtap"] -> [w1543] mode=indexing
                tunnel: w1473 -> [w1542]
                tunnel: [w1541] -> w1493 mode=indexing if=w1538
                tunnel: w1500 -> [w1539] mode=indexing
                tunnel: [w1539] -> w1492 mode=indexing if=w1538
                n733 = Concatenate Strings(w1542, w1543) -> (w1541:string)
                n734 = Not Equal?(x=w1539, y=cluster{"X":dbl[], "Y":dbl[]} {"X"=[], "Y"=[]}) -> (x != y?=w1538:bool)
              }
              n735 = Bundle By Name(cluster=w1471, "nomi plot"=w1493, "plot"=w1492, "#collaudo"=w1472) -> (w1491:T32)
              n736 = Bundle By Name(cluster=w1471, "nomi plot"=w1498, "plot"=w1497, "#collaudo"=w1472) -> (w1496:T32)
              n737 = Bundle By Name(cluster=w1471, "nomi plot"=w1495, "plot"=w1494, "#collaudo"=w1472) -> (w1490:T32)
              n738 = Bundle By Name(cluster=w1471, "nomi plot"=w1476, "plot"=w1477, "#collaudo"=w1472) -> (w1470:T32)
              n739 = Not(x=w1461) -> (.not. x?=w1469:bool)
            }
            n740 = local read "Stili grafico"() -> (w1317:T10)
            n741 = Or Array Elements(Boolean array=w1299) -> (logical OR=w1274:bool)
            n742 = Or Array Elements(Boolean array=w1293) -> (logical OR=w1273:bool)
            n743 = Or Array Elements(Boolean array=w1298) -> (logical OR=w1271:bool)
            n744 = Or Array Elements(Boolean array=w1296) -> (logical OR=w1272:bool)
            n745 = Unbundle By Name(w1317) -> ("Stile grafici Tabella 1"=w1316:T30, "Stile grafici Tabella 2"=w1315:T30, "Stile grafici Tabella 3"=w1314:T30)
            n746 = for {
              tunnel: w1310 -> [w1416] mode=indexing
              tunnel: w1317 -> [w1412]
              tunnel: w1308 -> [w1414] mode=indexing
              tunnel: w1309 -> [_] mode=indexing
              i -> [w1404]
              # "gestione legenda"
              n747 = Unbundle By Name(w1412) -> ("Colore collaudo report"=w1411:u32, "Colore collaudo confronto 1"=w1410:u32, "Colore collaudo confronto 2"=w1409:u32, "Colore collaudo confronto 3"=w1408:u32, "Colore collaudo confronto 4"=w1407:u32, "Colore collaudo confronto 5"=w1406:u32)
              n748 = Unbundle By Name(w1414) -> ("nome collaudo"=w1413:string)
              n749 = Build Array(w1411, w1410, w1409, w1408, w1407, w1406) -> (w1405:u32[])
              n750 = Index Array(array=w1405, index=w1404) -> (element=w1403:u32)
              n751 = To More Specific Class(target class=refnum<vi> refnum ("Colore collaudo report 6"), reference=w1416) -> (specific class reference=w1415:refnum<vi>)  [unwired: 1 in, 1 out]
              n752 = property class="ColBox"(reference=w1415, "Value"=w1403, "Caption.Text"=w1413, "Visible"=TRUE) -> ()  [unwired: 1 in, 2 out]
            }
            n753 = Or Array Elements(Boolean array=w1292) -> (logical OR=w1270:bool)
            n754 = Or Array Elements(Boolean array=w1294) -> (logical OR=w1269:bool)
            n755 = Or(x=w1273, y=w1270) -> (x .or. y?=w1297:bool)
            n756 = Array Subset(array=w1310, index=6) -> (w1312:refnum<vi>[])  [unwired: 1 in]
            n757 = Or(x=w1274, y=w1271) -> (x .or. y?=w1300:bool)
            n758 = Or(x=w1272, y=w1269) -> (x .or. y?=w1295:bool)
            n759 = Build Array(w1316, w1315, w1314) -> (w1311:T33)
            n760 = Build Array(w1300, w1297, w1295) -> (w1307:bool[])
            n761 = for {
              tunnel: w1312 -> [w1396] mode=indexing
              tunnel: w1311 -> [w1398] mode=indexing
              tunnel: w1307 -> [w1390] mode=indexing
              n762 = Unbundle By Name(w1398) -> ("stile linea"=w1393:u16, "stile punto"=w1392:u16)
              n763 = To More Specific Class(target class=refnum<vi> refnum ("Tabella 3"), reference=w1396) -> (specific class reference=w1395:refnum<vi>)  [unwired: 1 in, 1 out]
              n764 = Bundle By Name(cluster=cluster{"stile linea":u16, "stile punto":u16} {"stile linea"=0, "stile punto"=0} ("Value"), "stile linea"=w1393, "stile punto"=w1392) -> (w1391:cluster{"stile linea":u16, "stile punto":u16})
              n765 = property class="Clust (strict)"(reference=w1395, "Value"=w1391, "Visible"=w1390) -> ()  [unwired: 1 in, 2 out]
            }
            n766 = Build Array (concatenate)(w1348, w1290) -> (w1291:T34)
            n767 = local read "toll P2"() -> (w1363:dbl)
            n768 = local read "toll Q"() -> (w1364:dbl)
            n769 = local read item#-1() -> (w1366)
            n770 = local read item#-1() -> (w1365)
            n771 = for {
              tunnel: w1355 -> [w1454] mode=indexing
              tunnel: [w1451] -> w1353 mode=concatenating
              tunnel: [w1453] -> w1354 mode=concatenating
              tunnel: [w1449] -> w1335 mode=concatenating
              n772 = Unbundle By Name(w1454) -> ("nomi plot"=w1451:string[], "plot"=w1453:cluster{"X":dbl[], "Y":dbl[]}[], "#collaudo"=w1452:i32)
              n773 = Array Size(array=w1451) -> (size(s)=w1450:i32)
              n774 = Initialize Array(w1452, w1450) -> (w1449:i32[])
            }
            n775 = for {
              tunnel: [w1446] -> w1333 mode=concatenating
              tunnel: [w1448] -> w1342 mode=concatenating
              tunnel: [w1444] -> w1323 mode=concatenating
              tunnel: w1351 -> [w1443] mode=indexing
              n776 = Unbundle By Name(w1443) -> ("nomi plot"=w1446:string[], "plot"=w1448:cluster{"X":dbl[], "Y":dbl[]}[], "#collaudo"=w1447:i32)
              n777 = Array Size(array=w1446) -> (size(s)=w1445:i32)
              n778 = Initialize Array(w1447, w1445) -> (w1444:i32[])
            }
            n779 = for {
              tunnel: w1291 -> [w1442] mode=indexing
              tunnel: [w1439] -> w1350 mode=concatenating
              tunnel: [w1441] -> w1338 mode=concatenating
              tunnel: [w1437] -> w1330 mode=concatenating
              n780 = Unbundle By Name(w1442) -> ("nomi plot"=w1439:string[], "plot"=w1441:cluster{"X":dbl[], "Y":dbl[]}[], "#collaudo"=w1440:i32)
              n781 = Array Size(array=w1439) -> (size(s)=w1438:i32)
              n782 = Initialize Array(w1440, w1438) -> (w1437:i32[])
            }
            n783 = call "Croce.vi"("Solo toll Y positiva?"=TRUE, "TOLL Y %"=w1363, "TOLL X %"=w1364, "Grandezza Y"=w1365, "grandezza X"=w1366) -> ("element"=w1289:cluster{"X":dbl[], "Y":dbl[]})  [unwired: 6 in]
            n784 = Select(t=w1289, s=w1280, f=cluster{"X":dbl[], "Y":dbl[]} {"X"=[], "Y"=[]}) -> (s? t:f=w1288:cluster{"X":dbl[], "Y":dbl[]})
            n785 = Select(t="P2[kW]" ("Y Scale.Name Label.Text"), s=w1280, f="P1[kW]" ("Y Scale.Name Label.Text")) -> (s? t:f=w1282:string)
            n786 = Select(t="Effp[%]" ("Y Scale.Name Label.Text"), s=w1280, f="EffGr[%]" ("Y Scale.Name Label.Text")) -> (s? t:f=w1281:string)
            n787 = local read "toll Q"() -> (w1368:dbl)
            n788 = local read "toll H"() -> (w1367:dbl)
            n789 = Unbundle By Name(w1277) -> ("QH"=w1347:cluster{"X":dbl[], "Y":dbl[]}[], "QRPM"=w1344:cluster{"X":dbl[], "Y":dbl[]}[], "QP2"=w1340:cluster{"X":dbl[], "Y":dbl[]}[])
            n790 = local read item#-1() -> (w1370)
            n791 = local read item#-1() -> (w1369)
            n792 = local read item#-1() -> (w1372)
            n793 = local read item#-1() -> (w1371)
            n794 = call "Croce.vi"("Solo toll Y positiva?"=FALSE, "TOLL Y %"=w1367, "TOLL X %"=w1368, "Grandezza Y"=w1369, "grandezza X"=w1370) -> ("element"=w1356:cluster{"X":dbl[], "Y":dbl[]})  [unwired: 6 in]
            n795 = call "Croce.vi"("Solo toll Y positiva?"=FALSE, "TOLL Y %"=w1367, "TOLL X %"=w1368, "Grandezza Y"=w1371, "grandezza X"=w1372) -> ("element"=w1357:cluster{"X":dbl[], "Y":dbl[]})  [unwired: 6 in]
            n796 = Build Array (concatenate)(w1354, w1357, w1356) -> (w1346:cluster{"X":dbl[], "Y":dbl[]}[])
            n797 = Build Array (concatenate)(w1338, w1288) -> (w1337:cluster{"X":dbl[], "Y":dbl[]}[])
            n798 = Build Array (concatenate)(w1353, "CROCE Q1H1" ("string"), "CROCE Q2H2" ("string")) -> (w1352:string[])
            n799 = Build Array (concatenate)(w1335, w1328, w1328) -> (w1326:i32[])
            n800 = Build Array (concatenate)(w1330, -1) -> (w1319:i32[])
            n801 = Build Array (concatenate)(w1350, "CROCE QP2" ("string")) -> (w1332:string[])
            n802 = for {
              tunnel: w1352 -> [w1458] mode=indexing
              tunnel: [w1456] -> w1301 mode=indexing
              n803 = Bundle By Name(cluster=T3 {"nome plot"="1--18--15--H--Tab1--QH", "colore"=0, "Larghezza linea"=2, "stile linea"=0, "stile punto"=2, "Visibile?"=TRUE, "interpola?"=FALSE, "ordine"=2.0, "ScalaY"=0.0, "Etichetta?"=FALSE, "Freccia? 2"=FALSE, "nome tab?"=FALSE, "Asse Y grafico"="", "Asse X grafico"="", "Grandezza X"="", "Grandezza Y"="", "Collegamento"=0} ("Cluster"), "nome plot"=w1458, "Visibile?"=TRUE, "ScalaY"=0.0) -> (w1456:T3)
            }
            n804 = for {
              tunnel: w1333 -> [w1435] mode=indexing
              tunnel: [w1433] -> w1325 mode=indexing
              n805 = Bundle By Name(cluster=T3 {"nome plot"="1--18--15--H--Tab1--QH", "colore"=0, "Larghezza linea"=2, "stile linea"=0, "stile punto"=2, "Visibile?"=TRUE, "interpola?"=FALSE, "ordine"=2.0, "ScalaY"=0.0, "Etichetta?"=FALSE, "Freccia? 2"=FALSE, "nome tab?"=FALSE, "Asse Y grafico"="", "Asse X grafico"="", "Grandezza X"="", "Grandezza Y"="", "Collegamento"=0} ("Cluster"), "nome plot"=w1435, "Visibile?"=TRUE, "ScalaY"=0.0) -> (w1433:T3)
            }
            n806 = for {
              tunnel: w1332 -> [w1420] mode=indexing
              tunnel: [w1430] -> w1322 mode=indexing
              w1422 = "QEtag" ("search string")
              w1426 = "QEtap" ("search string")
              n807 = Search and Replace String(input string=w1420, search string=w1426, replace string=w1426) -> (number of replacements=w1427:i32)  [unwired: 5 in, 3 out]
              n808 = Search and Replace String(input string=w1420, search string=w1422, replace string=w1422) -> (number of replacements=w1421:i32)  [unwired: 5 in, 3 out]
              n809 = Not Equal To 0?(x=w1427) -> (x != 0?=w1428:bool)
              n810 = Not Equal To 0?(x=w1421) -> (x != 0?=w1418:bool)
              n811 = Or(x=w1428, y=w1418) -> (x .or. y?=w1419:bool)
              n812 = Select(t=1, s=w1419, f=0) -> (s? t:f=w1425:i32)
              n813 = Bundle By Name(cluster=T3 {"nome plot"="1--18--15--H--Tab1--QH", "colore"=0, "Larghezza linea"=2, "stile linea"=0, "stile punto"=2, "Visibile?"=TRUE, "interpola?"=FALSE, "ordine"=2.0, "ScalaY"=0.0, "Etichetta?"=FALSE, "Freccia? 2"=FALSE, "nome tab?"=FALSE, "Asse Y grafico"="", "Asse X grafico"="", "Grandezza X"="", "Grandezza Y"="", "Collegamento"=0} ("Cluster"), "nome plot"=w1420, "Visibile?"=TRUE, "ScalaY"=w1425) -> (w1430:T3)
            }
            n814 = Replace Array Subset(array=w1347, new element=w1346, index=w1341) -> (w1345:cluster{"X":dbl[], "Y":dbl[]}[])
            n815 = Replace Array Subset(array=w1344, new element=w1342, index=w1341) -> (w1343:cluster{"X":dbl[], "Y":dbl[]}[])
            n816 = Replace Array Subset(array=w1340, new element=w1337, index=w1341) -> (w1339:cluster{"X":dbl[], "Y":dbl[]}[])
            n817 = Bundle By Name(cluster=w1277, "QH"=w1345, "QRPM"=w1343, "QP2"=w1339) -> (w1336:T17)
            n818 = control-ref of="PLOT LEGEND QH-QH"() -> (w1303:refnum<vi>)
            n819 = control-ref of="PLOT LEGEND QH-QRPM"() -> (w1334:refnum<vi>)
            n820 = control-ref of="PLOT LEGEND QH-QP2"() -> (w1331:refnum<vi>)
            n821 = call "Set default graph style.vi"("numero collaudo"=w1326, "Stili default"="Stili grafico", "PLOT LEGEND in"=w1301) -> ("PLOT LEGEND out"=w1302:T3[])  [unwired: 8 in]
            n822 = call "Set default graph style.vi"("numero collaudo"=w1323, "Stili default"="Stili grafico", "PLOT LEGEND in"=w1325) -> ("PLOT LEGEND out"=w1324:T3[])  [unwired: 8 in]
            n823 = call "Set default graph style.vi"("numero collaudo"=w1319, "Stili default"="Stili grafico", "PLOT LEGEND in"=w1322) -> ("PLOT LEGEND out"=w1321:T3[])  [unwired: 8 in]
            n824 = property class="Arr (strict)"(reference=w1303, "Value"=w1302) -> ()  [unwired: 1 in, 2 out]
            n825 = property class="Arr (strict)"(reference=w1334, "Value"=w1324) -> ()  [unwired: 1 in, 2 out]
            n826 = property class="Arr (strict)"(reference=w1331, "Value"=w1321) -> ()  [unwired: 1 in, 2 out]
            "update annotation" <- TRUE
            "Case carica grafici" <- w1268
            "carica grafici" <- TRUE
          }
          frame Enabled {
          }
        }
      }
      frame "Carica grafici T" {
        n827 = disable-structure shown="Disabled" {
          disable-tunnel: w1565 -> [w1615 _]
          disable-tunnel: w1564 -> [w1614 _]
          disable-tunnel: w1562 -> [w1612 _]
          disable-tunnel: w1561 -> [w1583 _]
          disable-tunnel: [w1579 _] -> w1560
          disable-tunnel: w1558 -> [w1571 _]
          disable-tunnel: w1557 -> [w1570 _]
          frame Disabled {
            w1604 = 0 ("index")
            n828 = local read "trifase?"() -> (w1577:bool)
            n829 = Build Array (concatenate)(w1614, w1615) -> (w1589:T27[])
            n830 = for {
              tunnel: w1589 -> [w1616] mode=indexing
              tunnel: [w1619] -> w1588 mode=indexing
              tunnel: [w1618] -> w1587 mode=indexing
              tunnel: [w1617] -> w1586 mode=indexing
              w1620 = string[][] [] ("y")
              n831 = Unbundle By Name(w1616) -> ("Curva 1"=w1623, "Curva 2"=w1622, "Curva 3"=w1621)
              n832 = Not Equal?(x=w1623, y=w1620) -> (x != y?=w1619:bool)
              n833 = Not Equal?(x=w1622, y=w1620) -> (x != y?=w1618:bool)
              n834 = Not Equal?(x=w1621, y=w1620) -> (x != y?=w1617:bool)
            }
            n835 = local write "Case carica grafici"(w1570) -> ()
            n836 = Enqueue Element(queue=w1612, element=cluster{"String":string, "variant":variant} {"String"="Grafica", "variant"=variant}) -> ()  [unwired: 2 in, 3 out]
            n837 = property on="Legenda dt" class="Clust (strict)"() -> ("Controls[]"=w1572:refnum<vi>[])  [unwired: 2 in, 2 out]
            n838 = Boolean To (0,1)(Boolean=w1577) -> (0, 1=w1584:i16)
            n839 = for {
              N: 6 -> [_]
              tunnel: w1572 -> [w1635] mode=indexing
              tunnel: [w1633] -> w1590 mode=indexing
              n840 = property class="Ctl"(reference=w1635, "Visible"=FALSE) -> (error out=w1633:errorcluster)  [unwired: 1 in, 1 out]
            }
            n841 = local read "Stili grafico"() -> (w1575:T10)
            n842 = for {
              tunnel: w1589 -> [w1691] mode=indexing
              tunnel: w1583 -> [w1690]
              tunnel: [w1685] -> w1611 mode=indexing
              tunnel: [w1683] -> w1610 mode=indexing
              tunnel: w1584 -> [w1682]
              tunnel: w1577 -> [w1680]
              i -> [w1684]
              n843 = Index Array(array=w1690, index=w1682) -> (element=w1689:T19)
              n844 = Unbundle By Name(w1691) -> ("nome collaudo"=w1686:string, "Curva 1"=w1681)
              n845 = Unbundle By Name(w1689) -> ("tempo"=w1687:i32, "temperature.DT"=w1688:i32, "temperature.DTmarcia"=w1679:i32, "temperature.DTaux"=w1678:i32, "temperature.TC1"=w1677:i32, "temperature.TC2"=w1676:i32, "temperature.TC3"=w1675:i32, "temperature.TC4"=w1674:i32)
              n846 = case shown="True" w1680 {
                tunnel: w1688 -> [_ w1732]
                tunnel: w1687 -> [w1698 w1738]
                tunnel: w1686 -> [w1710 w1748]
                tunnel: [w1707 w1745] -> w1685
                tunnel: w1684 -> [w1703 w1741]
                tunnel: [w1702 w1740] -> w1683
                tunnel: w1681 -> [w1697 w1737]
                tunnel: w1679 -> [w1700 _]
                tunnel: w1678 -> [w1699 _]
                tunnel: w1677 -> [w1696 w1736]
                tunnel: w1676 -> [w1695 w1735]
                tunnel: w1675 -> [w1694 w1734]
                tunnel: w1674 -> [w1693 w1733]
                frame False {
                  w1704 = T32 {"nomi plot"=[], "plot"=[], "#collaudo"=0} ("output cluster")
                  # "monofase"
                  n847 = call "GRAFICA CURVA XY.vi"("Y INDEX"=w1700, "X INDEX"=w1698, "Curva 1"=w1697) -> ("Cluster"=w1718:cluster{"X":dbl[], "Y":dbl[]})  [unwired: 8 in]
                  n848 = call "GRAFICA CURVA XY.vi"("Y INDEX"=w1699, "X INDEX"=w1698, "Curva 1"=w1697) -> ("Cluster"=w1717:cluster{"X":dbl[], "Y":dbl[]})  [unwired: 8 in]
                  n849 = call "GRAFICA CURVA XY.vi"("Y INDEX"=w1696, "X INDEX"=w1698, "Curva 1"=w1697) -> ("Cluster"=w1715:cluster{"X":dbl[], "Y":dbl[]})  [unwired: 8 in]
                  n850 = call "GRAFICA CURVA XY.vi"("Y INDEX"=w1695, "X INDEX"=w1698, "Curva 1"=w1697) -> ("Cluster"=w1714:cluster{"X":dbl[], "Y":dbl[]})  [unwired: 8 in]
                  n851 = call "GRAFICA CURVA XY.vi"("Y INDEX"=w1694, "X INDEX"=w1698, "Curva 1"=w1697) -> ("Cluster"=w1713:cluster{"X":dbl[], "Y":dbl[]})  [unwired: 8 in]
                  n852 = call "GRAFICA CURVA XY.vi"("Y INDEX"=w1693, "X INDEX"=w1698, "Curva 1"=w1697) -> ("Cluster"=w1692:cluster{"X":dbl[], "Y":dbl[]})  [unwired: 8 in]
                  n853 = Build Array(w1715, w1714, w1713, w1692) -> (w1711:cluster{"X":dbl[], "Y":dbl[]}[])
                  n854 = Build Array(w1718, w1717) -> (w1716:cluster{"X":dbl[], "Y":dbl[]}[])
                  n855 = for {
                    tunnel: string[] ["--Tab1--TC1", "--Tab1--TC2", "--Tab1--TC3", "--Tab1--TC4"] -> [w1724] mode=indexing
                    tunnel: w1710 -> [w1723]
                    tunnel: [w1722] -> w1706 mode=indexing if=w1719
                    tunnel: w1711 -> [w1720] mode=indexing
                    tunnel: [w1720] -> w1705 mode=indexing if=w1719
                    n856 = Concatenate Strings(w1723, w1724) -> (w1722:string)
                    n857 = Not Equal?(x=w1720, y=cluster{"X":dbl[], "Y":dbl[]} {"X"=[], "Y"=[]}) -> (x != y?=w1719:bool)
                  }
                  n858 = for {
                    tunnel: string[] ["--Tab1--DTmarcia", "--Tab1--DTaux"] -> [w1730] mode=indexing
                    tunnel: w1710 -> [w1729]
                    tunnel: [w1728] -> w1709 mode=indexing if=w1725
                    tunnel: w1716 -> [w1726] mode=indexing
                    tunnel: [w1726] -> w1708 mode=indexing if=w1725
                    n859 = Concatenate Strings(w1729, w1730) -> (w1728:string)
                    n860 = Not Equal?(x=w1726, y=cluster{"X":dbl[], "Y":dbl[]} {"X"=[], "Y"=[]}) -> (x != y?=w1725:bool)
                  }
                  n861 = Bundle By Name(cluster=w1704, "nomi plot"=w1709, "plot"=w1708, "#collaudo"=w1703) -> (w1707:T32)
                  n862 = Bundle By Name(cluster=w1704, "nomi plot"=w1706, "plot"=w1705, "#collaudo"=w1703) -> (w1702:T32)
                }
                frame True {
                  w1742 = T32 {"nomi plot"=[], "plot"=[], "#collaudo"=0} ("output cluster")
                  # "trifase"
                  n863 = call "GRAFICA CURVA XY.vi"("Y INDEX"=w1732, "X INDEX"=w1738, "Curva 1"=w1737) -> ("Cluster"=w1755:cluster{"X":dbl[], "Y":dbl[]})  [unwired: 8 in]
                  n864 = call "GRAFICA CURVA XY.vi"("Y INDEX"=w1736, "X INDEX"=w1738, "Curva 1"=w1737) -> ("Cluster"=w1753:cluster{"X":dbl[], "Y":dbl[]})  [unwired: 8 in]
                  n865 = call "GRAFICA CURVA XY.vi"("Y INDEX"=w1735, "X INDEX"=w1738, "Curva 1"=w1737) -> ("Cluster"=w1752:cluster{"X":dbl[], "Y":dbl[]})  [unwired: 8 in]
                  n866 = call "GRAFICA CURVA XY.vi"("Y INDEX"=w1734, "X INDEX"=w1738, "Curva 1"=w1737) -> ("Cluster"=w1751:cluster{"X":dbl[], "Y":dbl[]})  [unwired: 8 in]
                  n867 = call "GRAFICA CURVA XY.vi"("Y INDEX"=w1733, "X INDEX"=w1738, "Curva 1"=w1737) -> ("Cluster"=w1731:cluster{"X":dbl[], "Y":dbl[]})  [unwired: 8 in]
                  n868 = Build Array(w1753, w1752, w1751, w1731) -> (w1749:cluster{"X":dbl[], "Y":dbl[]}[])
                  n869 = Build Array(w1755) -> (w1754:cluster{"X":dbl[], "Y":dbl[]}[])
                  n870 = for {
                    tunnel: string[] ["--Tab1--TC1", "--Tab1--TC2", "--Tab1--TC3", "--Tab1--TC4"] -> [w1761] mode=indexing
                    tunnel: w1748 -> [w1760]
                    tunnel: [w1759] -> w1744 mode=indexing if=w1756
                    tunnel: w1749 -> [w1757] mode=indexing
                    tunnel: [w1757] -> w1743 mode=indexing if=w1756
                    n871 = Concatenate Strings(w1760, w1761) -> (w1759:string)
                    n872 = Not Equal?(x=w1757, y=cluster{"X":dbl[], "Y":dbl[]} {"X"=[], "Y"=[]}) -> (x != y?=w1756:bool)
                  }
                  n873 = for {
                    tunnel: string[] ["--Tab1--DT"] -> [w1767] mode=indexing
                    tunnel: w1748 -> [w1766]
                    tunnel: [w1765] -> w1747 mode=indexing if=w1762
                    tunnel: w1754 -> [w1763] mode=indexing
                    tunnel: [w1763] -> w1746 mode=indexing if=w1762
                    n874 = Concatenate Strings(w1766, w1767) -> (w1765:string)
                    n875 = Not Equal?(x=w1763, y=cluster{"X":dbl[], "Y":dbl[]} {"X"=[], "Y"=[]}) -> (x != y?=w1762:bool)
                  }
                  n876 = Bundle By Name(cluster=w1742, "nomi plot"=w1747, "plot"=w1746, "#collaudo"=w1741) -> (w1745:T32)
                  n877 = Bundle By Name(cluster=w1742, "nomi plot"=w1744, "plot"=w1743, "#collaudo"=w1741) -> (w1740:T32)
                }
              }
            }
            n878 = Unbundle By Name(w1575) -> ("Stile grafici Tabella 1"=w1596:T30, "Stile grafici Tabella 2"=w1595:T30, "Stile grafici Tabella 3"=w1594:T30)
            n879 = for {
              tunnel: w1572 -> [w1650] mode=indexing
              tunnel: w1575 -> [w1646]
              tunnel: w1589 -> [w1648] mode=indexing
              tunnel: w1590 -> [_] mode=indexing
              i -> [w1638]
              # "gestione legenda"
              n880 = Unbundle By Name(w1646) -> ("Colore collaudo report"=w1645:u32, "Colore collaudo confronto 1"=w1644:u32, "Colore collaudo confronto 2"=w1643:u32, "Colore collaudo confronto 3"=w1642:u32, "Colore collaudo confronto 4"=w1641:u32, "Colore collaudo confronto 5"=w1640:u32)
              n881 = Unbundle By Name(w1648) -> ("nome collaudo"=w1647:string)
              n882 = Build Array(w1645, w1644, w1643, w1642, w1641, w1640) -> (w1639:u32[])
              n883 = Index Array(array=w1639, index=w1638) -> (element=w1637:u32)
              n884 = To More Specific Class(target class=refnum<vi> refnum ("Colore collaudo report 6"), reference=w1650) -> (specific class reference=w1649:refnum<vi>)  [unwired: 1 in, 1 out]
              n885 = property class="ColBox"(reference=w1649, "Value"=w1637, "Caption.Text"=w1647, "Visible"=TRUE) -> ()  [unwired: 1 in, 2 out]
            }
            n886 = Or Array Elements(Boolean array=w1587) -> (logical OR=w1567:bool)
            n887 = Or Array Elements(Boolean array=w1588) -> (logical OR=w1568:bool)
            n888 = Or Array Elements(Boolean array=w1586) -> (logical OR=w1566:bool)
            n889 = Array Subset(array=w1572, index=6) -> (w1592:refnum<vi>[])  [unwired: 1 in]
            n890 = Build Array(w1568, w1567, w1566) -> (w1585:bool[])
            n891 = Build Array(w1596, w1595, w1594) -> (w1591:T33)
            n892 = for {
              tunnel: w1592 -> [w1630] mode=indexing
              tunnel: w1591 -> [w1632] mode=indexing
              tunnel: w1585 -> [w1624] mode=indexing
              n893 = Unbundle By Name(w1632) -> ("stile linea"=w1627:u16, "stile punto"=w1626:u16)
              n894 = To More Specific Class(target class=refnum<vi> refnum ("Tabella 3"), reference=w1630) -> (specific class reference=w1629:refnum<vi>)  [unwired: 1 in, 1 out]
              n895 = Bundle By Name(cluster=cluster{"stile linea":u16, "stile punto":u16} {"stile linea"=0, "stile punto"=0} ("Value"), "stile linea"=w1627, "stile punto"=w1626) -> (w1625:cluster{"stile linea":u16, "stile punto":u16})
              n896 = property class="Clust (strict)"(reference=w1629, "Value"=w1625, "Visible"=w1624) -> ()  [unwired: 1 in, 2 out]
            }
            n897 = local write "carica grafici"(TRUE ("carica grafici")) -> ()
            n898 = for {
              tunnel: w1611 -> [w1668] mode=indexing
              tunnel: [w1665] -> w1580 mode=concatenating
              tunnel: [w1667] -> w1578 mode=concatenating
              tunnel: [w1663] -> w1581 mode=concatenating
              n899 = Unbundle By Name(w1668) -> ("nomi plot"=w1665:string[], "plot"=w1667:cluster{"X":dbl[], "Y":dbl[]}[], "#collaudo"=w1666:i32)
              n900 = Array Size(array=w1665) -> (size(s)=w1664:i32)
              n901 = Initialize Array(w1666, w1664) -> (w1663:i32[])
            }
            n902 = for {
              tunnel: [w1660] -> w1603 mode=concatenating
              tunnel: [w1662] -> w1605 mode=concatenating
              tunnel: [w1658] -> w1598 mode=concatenating
              tunnel: w1610 -> [w1657] mode=indexing
              n903 = Unbundle By Name(w1657) -> ("nomi plot"=w1660:string[], "plot"=w1662:cluster{"X":dbl[], "Y":dbl[]}[], "#collaudo"=w1661:i32)
              n904 = Array Size(array=w1660) -> (size(s)=w1659:i32)
              n905 = Initialize Array(w1661, w1659) -> (w1658:i32[])
            }
            n906 = local write "update annotation"(TRUE) -> ()
            n907 = Unbundle By Name(w1571) -> ("DT"=w1609:cluster{"X":dbl[], "Y":dbl[]}[], "TC"=w1607:cluster{"X":dbl[], "Y":dbl[]}[])
            n908 = control-ref of="PLOT LEGEND T-DT"() -> (w1574:refnum<vi>)
            n909 = control-ref of="PLOT LEGEND T-TC"() -> (w1573:refnum<vi>)
            n910 = Replace Array Subset(array=w1609, new element=w1578, index=w1604) -> (w1608:cluster{"X":dbl[], "Y":dbl[]}[])
            n911 = Replace Array Subset(array=w1607, new element=w1605, index=w1604) -> (w1606:cluster{"X":dbl[], "Y":dbl[]}[])
            n912 = for {
              tunnel: w1580 -> [w1672] mode=indexing
              tunnel: [w1670] -> w1602 mode=indexing
              n913 = Bundle By Name(cluster=T3 {"nome plot"="1--18--15--H--Tab1--QH", "colore"=0, "Larghezza linea"=2, "stile linea"=0, "stile punto"=2, "Visibile?"=TRUE, "interpola?"=FALSE, "ordine"=2.0, "ScalaY"=0.0, "Etichetta?"=FALSE, "Freccia? 2"=FALSE, "nome tab?"=FALSE, "Asse Y grafico"="", "Asse X grafico"="", "Grandezza X"="", "Grandezza Y"="", "Collegamento"=0} ("Cluster"), "nome plot"=w1672, "Visibile?"=TRUE, "ScalaY"=0.0) -> (w1670:T3)
            }
            n914 = for {
              tunnel: w1603 -> [w1655] mode=indexing
              tunnel: [w1653] -> w1600 mode=indexing
              n915 = Bundle By Name(cluster=T3 {"nome plot"="1--18--15--H--Tab1--QH", "colore"=0, "Larghezza linea"=2, "stile linea"=0, "stile punto"=2, "Visibile?"=TRUE, "interpola?"=FALSE, "ordine"=2.0, "ScalaY"=0.0, "Etichetta?"=FALSE, "Freccia? 2"=FALSE, "nome tab?"=FALSE, "Asse Y grafico"="", "Asse X grafico"="", "Grandezza X"="", "Grandezza Y"="", "Collegamento"=0} ("Cluster"), "nome plot"=w1655, "Visibile?"=TRUE, "ScalaY"=0.0) -> (w1653:T3)
            }
            n916 = local read "Stili grafico"() -> (w1576:T10)
            n917 = Bundle By Name(cluster=w1571, "DT"=w1608, "TC"=w1606) -> (w1579:T16)
            n918 = call "Set default graph style.vi"("numero collaudo"=w1581, "Stili default"=w1576, "PLOT LEGEND in"=w1602) -> ("PLOT LEGEND out"=w1601:T3[])  [unwired: 8 in]
            n919 = call "Set default graph style.vi"("numero collaudo"=w1598, "Stili default"=w1576, "PLOT LEGEND in"=w1600) -> ("PLOT LEGEND out"=w1599:T3[])  [unwired: 8 in]
            n920 = property class="Arr (strict)"(reference=w1573, "Value"=w1599) -> ()  [unwired: 1 in, 2 out]
            n921 = property class="Arr (strict)"(reference=w1574, "Value"=w1601) -> ()  [unwired: 1 in, 2 out]
          }
          frame Enabled {
          }
        }
      }
      frame "Carica grafici N" {
        n922 = disable-structure shown="Disabled" {
          disable-tunnel: w1777 -> [w1827 _]
          disable-tunnel: w1776 -> [w1826 _]
          disable-tunnel: w1774 -> [w1824 _]
          disable-tunnel: w1773 -> [w1795 _]
          disable-tunnel: w1771 -> [w1787 _]
          disable-tunnel: w1770 -> [w1782 _]
          disable-tunnel: [w1778 _] -> w1769
          frame Disabled {
            w1816 = 0 ("index")
            n923 = local read "trifase?"() -> (w1790:bool)
            n924 = Build Array (concatenate)(w1826, w1827) -> (w1801:T27[])
            n925 = for {
              tunnel: w1801 -> [w1828] mode=indexing
              tunnel: [w1831] -> w1800 mode=indexing
              tunnel: [w1830] -> w1799 mode=indexing
              tunnel: [w1829] -> w1798 mode=indexing
              w1832 = string[][] [] ("y")
              n926 = Unbundle By Name(w1828) -> ("Curva 1"=w1835, "Curva 2"=w1834, "Curva 3"=w1833)
              n927 = Not Equal?(x=w1835, y=w1832) -> (x != y?=w1831:bool)
              n928 = Not Equal?(x=w1834, y=w1832) -> (x != y?=w1830:bool)
              n929 = Not Equal?(x=w1833, y=w1832) -> (x != y?=w1829:bool)
            }
            n930 = local write "Case carica grafici"(w1787) -> ()
            n931 = Enqueue Element(queue=w1824, element=cluster{"String":string, "variant":variant} {"String"="Grafica", "variant"=variant}) -> ()  [unwired: 2 in, 3 out]
            n932 = Boolean To (0,1)(Boolean=w1790) -> (0, 1=w1796:i16)
            n933 = local read "Stili grafico"() -> (w1788:T10)
            n934 = for {
              tunnel: w1801 -> [w1907] mode=indexing
              tunnel: w1795 -> [w1906]
              tunnel: [w1902] -> w1823 mode=indexing
              tunnel: [w1900] -> w1822 mode=indexing
              tunnel: w1796 -> [w1899]
              tunnel: w1790 -> [w1898]
              i -> [w1901]
              n935 = Index Array(array=w1906, index=w1899) -> (element=w1890:T19)
              n936 = Unbundle By Name(w1907) -> ("nome collaudo"=w1903:string, "Curva 1"=w1891)
              n937 = Unbundle By Name(w1890) -> ("NPSH"=w1904:i32, "Htot"=w1905:i32, "Q"=w1897:i32, "temperature.DTaux"=w1896:i32, "temperature.TC1"=w1895:i32, "temperature.TC2"=w1894:i32, "temperature.TC3"=w1893:i32, "temperature.TC4"=w1892:i32)
              n938 = call "filtra per npsh.vi"("Curva 1"=w1891, "indici"=w1890) -> ("Cluster"=w1888:cluster{"index":i32, "length":i32}, "Pto npsh"=w1889:u8)  [unwired: 7 in, 1 out]
              n939 = Unbundle By Name(w1888) -> ("index"=w1887:i32, "length"=w1886:i32)
              n940 = case shown="True" w1898 {
                tunnel: w1905 -> [_ w1956]
                tunnel: w1904 -> [w1914 w1948]
                tunnel: w1903 -> [w1926 w1969]
                tunnel: [w1923 w1966] -> w1902
                tunnel: w1901 -> [w1919 w1962]
                tunnel: [w1918 w1961] -> w1900
                tunnel: w1891 -> [w1913 w1955]
                tunnel: w1897 -> [w1916 _]
                tunnel: w1896 -> [w1915 _]
                tunnel: w1895 -> [w1912 _]
                tunnel: w1894 -> [w1911 w1959]
                tunnel: w1893 -> [w1910 w1958]
                tunnel: w1892 -> [w1909 w1957]
                tunnel: w1887 -> [_ w1953]
                tunnel: w1886 -> [_ w1952]
                frame False {
                  w1920 = T32 {"nomi plot"=[], "plot"=[], "#collaudo"=0} ("output cluster")
                  # "monofase"
                  n941 = call "GRAFICA CURVA XY.vi"("Y INDEX"=w1916, "X INDEX"=w1914, "Curva 1"=w1913) -> ("Cluster"=w1934:cluster{"X":dbl[], "Y":dbl[]})  [unwired: 8 in]
                  n942 = call "GRAFICA CURVA XY.vi"("Y INDEX"=w1915, "X INDEX"=w1914, "Curva 1"=w1913) -> ("Cluster"=w1933:cluster{"X":dbl[], "Y":dbl[]})  [unwired: 8 in]
                  n943 = call "GRAFICA CURVA XY.vi"("Y INDEX"=w1912, "X INDEX"=w1914, "Curva 1"=w1913) -> ("Cluster"=w1931:cluster{"X":dbl[], "Y":dbl[]})  [unwired: 8 in]
                  n944 = call "GRAFICA CURVA XY.vi"("Y INDEX"=w1911, "X INDEX"=w1914, "Curva 1"=w1913) -> ("Cluster"=w1930:cluster{"X":dbl[], "Y":dbl[]})  [unwired: 8 in]
                  n945 = call "GRAFICA CURVA XY.vi"("Y INDEX"=w1910, "X INDEX"=w1914, "Curva 1"=w1913) -> ("Cluster"=w1929:cluster{"X":dbl[], "Y":dbl[]})  [unwired: 8 in]
                  n946 = call "GRAFICA CURVA XY.vi"("Y INDEX"=w1909, "X INDEX"=w1914, "Curva 1"=w1913) -> ("Cluster"=w1908:cluster{"X":dbl[], "Y":dbl[]})  [unwired: 8 in]
                  n947 = Build Array(w1931, w1930, w1929, w1908) -> (w1927:cluster{"X":dbl[], "Y":dbl[]}[])
                  n948 = Build Array(w1934, w1933) -> (w1932:cluster{"X":dbl[], "Y":dbl[]}[])
                  n949 = for {
                    tunnel: string[] ["--Tab1--TC1", "--Tab1--TC2", "--Tab1--TC3", "--Tab1--TC4"] -> [w1940] mode=indexing
                    tunnel: w1926 -> [w1939]
                    tunnel: [w1938] -> w1922 mode=indexing if=w1935
                    tunnel: w1927 -> [w1936] mode=indexing
                    tunnel: [w1936] -> w1921 mode=indexing if=w1935
                    n950 = Concatenate Strings(w1939, w1940) -> (w1938:string)
                    n951 = Not Equal?(x=w1936, y=cluster{"X":dbl[], "Y":dbl[]} {"X"=[], "Y"=[]}) -> (x != y?=w1935:bool)
                  }
                  n952 = for {
                    tunnel: string[] ["--Tab1--DTmarcia", "--Tab1--DTaux"] -> [w1946] mode=indexing
                    tunnel: w1926 -> [w1945]
                    tunnel: [w1944] -> w1925 mode=indexing if=w1941
                    tunnel: w1932 -> [w1942] mode=indexing
                    tunnel: [w1942] -> w1924 mode=indexing if=w1941
                    n953 = Concatenate Strings(w1945, w1946) -> (w1944:string)
                    n954 = Not Equal?(x=w1942, y=cluster{"X":dbl[], "Y":dbl[]} {"X"=[], "Y"=[]}) -> (x != y?=w1941:bool)
                  }
                  n955 = Bundle By Name(cluster=w1920, "nomi plot"=w1925, "plot"=w1924, "#collaudo"=w1919) -> (w1923:T32)
                  n956 = Bundle By Name(cluster=w1920, "nomi plot"=w1922, "plot"=w1921, "#collaudo"=w1919) -> (w1918:T32)
                }
                frame True {
                  w1963 = T32 {"nomi plot"=[], "plot"=[], "#collaudo"=0} ("output cluster")
                  # "trifase"
                  n957 = Array Subset(array=w1955, index (row)=w1953, length (row)=w1952) -> (w1954:void[][])  [unwired: 2 in]
                  n958 = call "GRAFICA CURVA XY.vi"("Y INDEX"=w1956, "X INDEX"=w1948, "Curva 1"=w1954) -> ("Cluster"=w1974:cluster{"X":dbl[], "Y":dbl[]})  [unwired: 8 in]
                  n959 = Add(x=w1948, y=2) -> (x+y=w1947:i32)
                  n960 = Add(x=w1948, y=4) -> (x+y=w1950:i32)
                  n961 = call "GRAFICA CURVA XY.vi"("Y INDEX"=w1947, "X INDEX"=w1950, "Curva 1"=w1955) -> ("Cluster"=w1972:cluster{"X":dbl[], "Y":dbl[]})  [unwired: 8 in]
                  n962 = call "GRAFICA CURVA XY.vi"("Y INDEX"=w1959, "X INDEX"=w1950, "Curva 1"=w1955) -> ()  [unwired: 8 in, 1 out]
                  n963 = call "GRAFICA CURVA XY.vi"("Y INDEX"=w1958, "X INDEX"=w1950, "Curva 1"=w1955) -> ()  [unwired: 8 in, 1 out]
                  n964 = call "GRAFICA CURVA XY.vi"("Y INDEX"=w1957, "X INDEX"=w1950, "Curva 1"=w1955) -> ()  [unwired: 8 in, 1 out]
                  n965 = Build Array(w1972) -> (w1970:cluster{"X":dbl[], "Y":dbl[]}[])
                  n966 = Build Array(w1974) -> (w1973:cluster{"X":dbl[], "Y":dbl[]}[])
                  n967 = for {
                    tunnel: string[] ["--Tab1--Q-npsh"] -> [w1980] mode=indexing
                    tunnel: w1969 -> [w1979]
                    tunnel: [w1978] -> w1965 mode=indexing if=w1975
                    tunnel: w1970 -> [w1976] mode=indexing
                    tunnel: [w1976] -> w1964 mode=indexing if=w1975
                    n968 = Concatenate Strings(w1979, w1980) -> (w1978:string)
                    n969 = Not Equal?(x=w1976, y=cluster{"X":dbl[], "Y":dbl[]} {"X"=[], "Y"=[]}) -> (x != y?=w1975:bool)
                  }
                  n970 = for {
                    tunnel: string[] ["--Tab1--npsh-H"] -> [w1986] mode=indexing
                    tunnel: w1969 -> [w1985]
                    tunnel: [w1984] -> w1968 mode=indexing if=w1981
                    tunnel: w1973 -> [w1982] mode=indexing
                    tunnel: [w1982] -> w1967 mode=indexing if=w1981
                    n971 = Concatenate Strings(w1985, w1986) -> (w1984:string)
                    n972 = Not Equal?(x=w1982, y=cluster{"X":dbl[], "Y":dbl[]} {"X"=[], "Y"=[]}) -> (x != y?=w1981:bool)
                  }
                  n973 = Bundle By Name(cluster=w1963, "nomi plot"=w1968, "plot"=w1967, "#collaudo"=w1962) -> (w1966:T32)
                  n974 = Bundle By Name(cluster=w1963, "nomi plot"=w1965, "plot"=w1964, "#collaudo"=w1962) -> (w1961:T32)
                }
              }
            }
            n975 = Unbundle By Name(w1788) -> ("Stile grafici Tabella 1"=w1808:T30, "Stile grafici Tabella 2"=w1807:T30, "Stile grafici Tabella 3"=w1806:T30)
            n976 = Or Array Elements(Boolean array=w1799) -> (logical OR=w1784:bool)
            n977 = Or Array Elements(Boolean array=w1800) -> (logical OR=w1785:bool)
            n978 = Or Array Elements(Boolean array=w1798) -> (logical OR=w1783:bool)
            n979 = Array Subset(index=6) -> (array=w1779:dbl[], w1804:void[])  [unwired: 1 in]
            n980 = for {
              N: 6 -> [_]
              tunnel: w1779 -> [w1847] mode=indexing
              tunnel: [w1845] -> w1802 mode=indexing
              n981 = property class="Ctl"(reference=w1847, "Visible"=FALSE) -> (error out=w1845:errorcluster)  [unwired: 1 in, 1 out]
            }
            n982 = for {
              tunnel: w1779 -> [w1862] mode=indexing
              tunnel: w1788 -> [w1858]
              tunnel: w1801 -> [w1860] mode=indexing
              tunnel: w1802 -> [_] mode=indexing
              i -> [w1850]
              # "gestione legenda"
              n983 = Unbundle By Name(w1858) -> ("Colore collaudo report"=w1857:u32, "Colore collaudo confronto 1"=w1856:u32, "Colore collaudo confronto 2"=w1855:u32, "Colore collaudo confronto 3"=w1854:u32, "Colore collaudo confronto 4"=w1853:u32, "Colore collaudo confronto 5"=w1852:u32)
              n984 = Unbundle By Name(w1860) -> ("nome collaudo"=w1859:string)
              n985 = Build Array(w1857, w1856, w1855, w1854, w1853, w1852) -> (w1851:u32[])
              n986 = Index Array(array=w1851, index=w1850) -> (element=w1849:u32)
              n987 = To More Specific Class(target class=refnum<vi> refnum ("Colore collaudo report 6"), reference=w1862) -> (specific class reference=w1861:refnum<vi>)  [unwired: 1 in, 1 out]
              n988 = property class="ColBox"(reference=w1861, "Value"=w1849, "Caption.Text"=w1859, "Visible"=TRUE) -> ()  [unwired: 1 in, 2 out]
            }
            n989 = Build Array(w1785, w1784, w1783) -> (w1797:bool[])
            n990 = Build Array(w1808, w1807, w1806) -> (w1803:T33)
            n991 = for {
              tunnel: w1804 -> [w1842] mode=indexing
              tunnel: w1803 -> [w1844] mode=indexing
              tunnel: w1797 -> [w1836] mode=indexing
              n992 = Unbundle By Name(w1844) -> ("stile linea"=w1839:u16, "stile punto"=w1838:u16)
              n993 = To More Specific Class(target class=refnum<vi> refnum ("Tabella 3"), reference=w1842) -> (specific class reference=w1841:refnum<vi>)  [unwired: 1 in, 1 out]
              n994 = Bundle By Name(cluster=cluster{"stile linea":u16, "stile punto":u16} {"stile linea"=0, "stile punto"=0} ("Value"), "stile linea"=w1839, "stile punto"=w1838) -> (w1837:cluster{"stile linea":u16, "stile punto":u16})
              n995 = property class="Clust (strict)"(reference=w1841, "Value"=w1837, "Visible"=w1836) -> ()  [unwired: 1 in, 2 out]
            }
            n996 = local write "carica grafici"(TRUE ("carica grafici")) -> ()
            n997 = for {
              tunnel: w1823 -> [w1880] mode=indexing
              tunnel: [w1877] -> w1792 mode=concatenating
              tunnel: [w1879] -> w1791 mode=concatenating
              tunnel: [w1875] -> w1793 mode=concatenating
              n998 = Unbundle By Name(w1880) -> ("nomi plot"=w1877:string[], "plot"=w1879:cluster{"X":dbl[], "Y":dbl[]}[], "#collaudo"=w1878:i32)
              n999 = Array Size(array=w1877) -> (size(s)=w1876:i32)
              n1000 = Initialize Array(w1878, w1876) -> (w1875:i32[])
            }
            n1001 = for {
              tunnel: [w1872] -> w1815 mode=concatenating
              tunnel: [w1874] -> w1817 mode=concatenating
              tunnel: [w1870] -> w1810 mode=concatenating
              tunnel: w1822 -> [w1869] mode=indexing
              n1002 = Unbundle By Name(w1869) -> ("nomi plot"=w1872:string[], "plot"=w1874:cluster{"X":dbl[], "Y":dbl[]}[], "#collaudo"=w1873:i32)
              n1003 = Array Size(array=w1872) -> (size(s)=w1871:i32)
              n1004 = Initialize Array(w1873, w1871) -> (w1870:i32[])
            }
            n1005 = local write "update annotation"(TRUE) -> ()
            n1006 = Unbundle By Name(w1782) -> ("NPSH-H"=w1821:cluster{"X":dbl[], "Y":dbl[]}[], "Q-NPSH"=w1819:cluster{"X":dbl[], "Y":dbl[]}[])
            n1007 = Replace Array Subset(array=w1821, new element=w1791, index=w1816) -> (w1820:cluster{"X":dbl[], "Y":dbl[]}[])
            n1008 = Replace Array Subset(array=w1819, new element=w1817, index=w1816) -> (w1818:cluster{"X":dbl[], "Y":dbl[]}[])
            n1009 = for {
              tunnel: w1792 -> [w1884] mode=indexing
              tunnel: [w1882] -> w1814 mode=indexing
              n1010 = Bundle By Name(cluster=T3 {"nome plot"="1--18--15--H--Tab1--QH", "colore"=0, "Larghezza linea"=2, "stile linea"=0, "stile punto"=2, "Visibile?"=TRUE, "interpola?"=FALSE, "ordine"=2.0, "ScalaY"=0.0, "Etichetta?"=FALSE, "Freccia? 2"=FALSE, "nome tab?"=FALSE, "Asse Y grafico"="", "Asse X grafico"="", "Grandezza X"="", "Grandezza Y"="", "Collegamento"=0} ("Cluster"), "nome plot"=w1884, "Visibile?"=TRUE, "ScalaY"=0.0) -> (w1882:T3)
            }
            n1011 = for {
              tunnel: w1815 -> [w1867] mode=indexing
              tunnel: [w1865] -> w1812 mode=indexing
              n1012 = Bundle By Name(cluster=T3 {"nome plot"="1--18--15--H--Tab1--QH", "colore"=0, "Larghezza linea"=2, "stile linea"=0, "stile punto"=2, "Visibile?"=TRUE, "interpola?"=FALSE, "ordine"=2.0, "ScalaY"=0.0, "Etichetta?"=FALSE, "Freccia? 2"=FALSE, "nome tab?"=FALSE, "Asse Y grafico"="", "Asse X grafico"="", "Grandezza X"="", "Grandezza Y"="", "Collegamento"=0} ("Cluster"), "nome plot"=w1867, "Visibile?"=TRUE, "ScalaY"=0.0) -> (w1865:T3)
            }
            n1013 = local read "Stili grafico"() -> (w1789:T10)
            n1014 = Bundle By Name(cluster=w1782, "NPSH-H"=w1820, "Q-NPSH"=w1818) -> (w1778:T15)
            n1015 = call "Set default graph style.vi"("numero collaudo"=w1793, "Stili default"=w1789, "PLOT LEGEND in"=w1814) -> ("PLOT LEGEND out"=w1813:T3[])  [unwired: 8 in]
            n1016 = call "Set default graph style.vi"("numero collaudo"=w1810, "Stili default"=w1789, "PLOT LEGEND in"=w1812) -> ("PLOT LEGEND out"=w1811:T3[])  [unwired: 8 in]
            n1017 = property class="Arr (strict)"("Value"=w1813) -> (reference=w1781:refnum<vi>)  [unwired: 1 in, 2 out]
            n1018 = property class="Arr"("Value"=w1811) -> (reference=w1780:refnum<vi>)  [unwired: 1 in, 2 out]
          }
          frame Enabled {
          }
        }
      }
      frame "Grafica" {
        n1019 = disable-structure shown="Disabled" {
          disable-tunnel: w1990 -> [w2002 _]
          disable-tunnel: w1989 -> [w1999 _]
          disable-tunnel: w1988 -> [w1998 _]
          disable-tunnel: w1987 -> [w1995 _]
          frame Disabled {
            n1020 = case shown="True" "grafica tutte" {
              tunnel: [w2127 string[] ["F", "N"]] -> w2000
              frame False {
                n1021 = local read "tipo prova"() -> (w2128:string)
                n1022 = Build Array(w2128) -> (w2127:string[])
              }
              frame True {
              }
            }
            n1023 = local read "carica grafici"() -> (w1996:bool)
            n1024 = Enqueue Element(queue=w2002, element=cluster{"String":string, "variant":variant} {"String"="Grafica", "variant"=variant}) -> (queue out=w1997:refnum<queue>)  [unwired: 2 in, 2 out]
            n1025 = case shown="True" w1996 {
              tunnel: w1997 -> [_ w2130]
              frame False {
              }
              frame True {
                n1026 = Enqueue Element(queue=w2130, element=cluster{"String":string, "variant":variant} {"String"="Set x scale", "variant"=variant}) -> ()  [unwired: 2 in, 3 out]
              }
            }
            n1027 = Wait (ms)(milliseconds to wait=u32 100) -> ()  [unwired: 1 out]
            n1028 = for {
              tunnel: w2000 -> [w2007] mode=indexing
              tunnel: w1999 -> [w2006]
              tunnel: w1998 -> [w2005]
              tunnel: w1995 -> [w2004]
              n1029 = case shown="\"F\", \"H\", Default" w2007 {
                tunnel: w2006 -> [_ w2058 _]
                tunnel: w2005 -> [w2010 _ _]
                tunnel: w2004 -> [_ _ w2084]
                frame "F", "H", Default {
                  n1030 = control-ref of="PLOT LEGEND QH-QH"() -> (w2023:refnum<vi>)
                  n1031 = control-ref of="PLOT LEGEND QH-QP2"() -> (w2021:refnum<vi>)
                  n1032 = control-ref of="PLOT LEGEND QH-QRPM"() -> (w2022:refnum<vi>)
                  n1033 = control-ref of="ProvaQH-QH"() -> (w2008:refnum<vi>)
                  n1034 = Unbundle By Name(w2010) -> ("QH"=w2031:cluster{"X":dbl[], "Y":dbl[]}[], "QRPM"=w2030:cluster{"X":dbl[], "Y":dbl[]}[], "QP2"=w2029:cluster{"X":dbl[], "Y":dbl[]}[])
                  n1035 = Build Array(w2031, w2030, w2029) -> (w2028:cluster{"X":dbl[], "Y":dbl[]}[][])
                  n1036 = Build Array(w2008) -> (w2025:refnum<vi>[], w2026:refnum<vi>, w2027:refnum<vi>)
                  n1037 = property class="Arr (strict)"(reference=w2023) -> ("Value"=w2009:T3[])  [unwired: 1 in, 2 out]
                  n1038 = property class="Arr (strict)"(reference=w2022) -> ("Value"=w2019:T3[])  [unwired: 1 in, 2 out]
                  n1039 = property class="Arr (strict)"(reference=w2021) -> ("Value"=w2016:T3[])  [unwired: 1 in, 2 out]
                  n1040 = Build Array(w2023, w2022, w2021) -> (w2024:refnum<vi>[])
                  n1041 = flat-sequence {
                    tunnel: w2012 -> [w2034]
                    tunnel: w2028 -> [w2038]
                    tunnel: w2025 -> [w2037]
                    tunnel: w2024 -> [w2036]
                    tunnel: "colori grafici" -> [w2032]
                    frame #0 {
                      n1042 = local read "update annotation"() -> (w2035:bool)
                      n1043 = Or(x=w2034, y=w2035) -> (x .or. y?=w2033:bool)
                      n1044 = for {
                        tunnel: w2037 -> [w2043] mode=indexing
                        tunnel: w2038 -> [w2042] mode=indexing
                        tunnel: w2036 -> [w2039] mode=indexing
                        tunnel: w2033 -> [w2041]
                        tunnel: w2032 -> [w2040]
                        n1045 = call "Gestione grafico.vi"("Array"=w2042, "colori grafico"=w2040, "PLOT LEGEND"=w2039, "graph ref"=w2043, "Update annotation?"=w2041) -> ("Array out"=w2044:cluster{"X":dbl[], "Y":dbl[]}[])  [unwired: 5 in]
                        n1046 = property class="XYGraph (strict)"(reference=w2043, "Value"=w2044) -> ()  [unwired: 1 in, 2 out]
                      }
                    }
                    frame #1 {
                      n1047 = local write "update annotation"(FALSE ("update annotation")) -> ()
                    }
                  }
                  n1048 = feedback #2() -> (w2020:T3[])  [unwired: 1 in]
                  n1049 = feedback-in #2(w2009) -> ()
                  n1050 = feedback #3() -> (w2018:T3[])  [unwired: 1 in]
                  n1051 = feedback-in #3(w2019) -> ()
                  n1052 = feedback #4() -> (w2017:T3[])  [unwired: 1 in]
                  n1053 = feedback-in #4(w2016) -> ()
                  n1054 = Not Equal?(x=w2009, y=w2020) -> (x != y?=w2015:bool)
                  n1055 = Not Equal?(x=w2019, y=w2018) -> (x != y?=w2014:bool)
                  n1056 = Not Equal?(x=w2016, y=w2017) -> (x != y?=w2013:bool)
                  n1057 = Compound Arithmetic op=OR(w2015, w2014, w2013) -> (w2012:bool)
                }
                frame "T" {
                  n1058 = control-ref of="ProvaT-TC"() -> (w2049:refnum<vi>)
                  n1059 = control-ref of="ProvaT-DT"() -> (w2050:refnum<vi>)
                  n1060 = control-ref of="PLOT LEGEND T-TC"() -> (w2047:refnum<vi>)
                  n1061 = control-ref of="PLOT LEGEND T-DT"() -> (w2048:refnum<vi>)
                  n1062 = Unbundle By Name(w2058) -> ("DT"=w2063:cluster{"X":dbl[], "Y":dbl[]}[], "TC"=w2062:cluster{"X":dbl[], "Y":dbl[]}[])
                  n1063 = Build Array(w2063, w2062) -> (w2061:cluster{"X":dbl[], "Y":dbl[]}[][])
                  n1064 = Build Array(w2050, w2049) -> (w2060:refnum<vi>[])
                  n1065 = local read "colori grafici"() -> (w2046:T11)
                  n1066 = property class="Arr (strict)"(reference=w2048) -> ("Value"=w2057:T3[])  [unwired: 1 in, 2 out]
                  n1067 = property class="Arr (strict)"(reference=w2047) -> ("Value"=w2055:T3[])  [unwired: 1 in, 2 out]
                  n1068 = Build Array(w2048, w2047) -> (w2059:refnum<vi>[])
                  n1069 = flat-sequence {
                    tunnel: w2051 -> [w2066]
                    tunnel: w2061 -> [w2070]
                    tunnel: w2060 -> [w2069]
                    tunnel: w2059 -> [w2068]
                    tunnel: w2046 -> [w2064]
                    frame #0 {
                      n1070 = local read "update annotation"() -> (w2067:bool)
                      n1071 = Or(x=w2066, y=w2067) -> (x .or. y?=w2065:bool)
                      n1072 = for {
                        tunnel: w2069 -> [w2075] mode=indexing
                        tunnel: w2070 -> [w2074] mode=indexing
                        tunnel: w2068 -> [w2071] mode=indexing
                        tunnel: w2065 -> [w2073]
                        tunnel: w2064 -> [w2072]
                        n1073 = call "Gestione grafico.vi"("Array"=w2074, "colori grafico"=w2072, "PLOT LEGEND"=w2071, "graph ref"=w2075, "Update annotation?"=w2073) -> ("Array out"=w2076:cluster{"X":dbl[], "Y":dbl[]}[])  [unwired: 5 in]
                        n1074 = property class="XYGraph (strict)"(reference=w2075, "Value"=w2076) -> ()  [unwired: 1 in, 2 out]
                      }
                    }
                    frame #1 {
                      n1075 = local write "update annotation"(FALSE ("update annotation")) -> ()
                    }
                  }
                  n1076 = feedback #5() -> (w2056:T3[])  [unwired: 1 in]
                  n1077 = feedback-in #5(w2057) -> ()
                  n1078 = feedback #6() -> (w2054:T3[])  [unwired: 1 in]
                  n1079 = feedback-in #6(w2055) -> ()
                  n1080 = Not Equal?(x=w2057, y=w2056) -> (x != y?=w2053:bool)
                  n1081 = Not Equal?(x=w2055, y=w2054) -> (x != y?=w2052:bool)
                  n1082 = Compound Arithmetic op=OR(w2053, w2052) -> (w2051:bool)
                }
                frame "N" {
                  n1083 = Unbundle By Name(w2084) -> ("NPSH-H"=w2096:cluster{"X":dbl[], "Y":dbl[]}[], "Q-NPSH"=w2079:cluster{"X":dbl[], "Y":dbl[]}[])
                  n1084 = for {
                    tunnel: w2079 -> [w2105] mode=indexing
                    tunnel: [w2097] -> w2078 mode=indexing
                    n1085 = Unbundle By Name(w2105) -> ("X"=w2099:dbl[], "Y"=w2098:dbl[])
                    n1086 = for {
                      tunnel: [w2111] -> w2101 mode=indexing
                      tunnel: w2099 -> [w2110] mode=indexing
                      tunnel: w2098 -> [w2109] mode=indexing
                      n1087 = Bundle(cluster=cluster{"x":dbl, "y":dbl} {"x"=0.0, "y"=0.0}, "x"=w2110, "y"=w2109) -> (w2111:cluster{"x":dbl, "y":dbl})
                    }
                    n1088 = Sort 1D Array(array=w2101) -> (sorted array=w2102:cluster{"x":dbl, "y":dbl}[])
                    n1089 = for {
                      tunnel: w2102 -> [w2108] mode=indexing
                      tunnel: [w2107] -> w2103 mode=indexing
                      tunnel: [w2106] -> w2104 mode=indexing
                      n1090 = Unbundle By Name(w2108) -> ("x"=w2107:dbl, "y"=w2106:dbl)
                    }
                    n1091 = Bundle By Name(cluster=cluster{"X":dbl[], "Y":dbl[]} {"X"=[], "Y"=[]}, "X"=w2103, "Y"=w2104) -> (w2097:cluster{"X":dbl[], "Y":dbl[]})
                  }
                  n1092 = Build Array(w2096, w2078) -> (w2095:cluster{"X":dbl[], "Y":dbl[]}[][])
                  n1093 = Build Array() -> (w2094:void[], w2083:dbl, w2082:dbl)
                  n1094 = local read "colori grafici"() -> (w2085:T11)
                  n1095 = property class="Arr"() -> (reference=w2080:refnum<vi>, "Value"=w2090:variant)  [unwired: 1 in, 2 out]
                  n1096 = Build Array(w2080) -> (w2093:void[], w2081:dbl)
                  n1097 = property class="Arr (strict)"(reference=w2081) -> ("Value"=w2092:T3[])  [unwired: 1 in, 2 out]
                  n1098 = flat-sequence {
                    tunnel: w2086 -> [w2115]
                    tunnel: w2095 -> [w2119]
                    tunnel: w2094 -> [w2118]
                    tunnel: w2093 -> [w2117]
                    tunnel: w2085 -> [w2113]
                    frame #0 {
                      n1099 = local read "update annotation"() -> (w2116:bool)
                      n1100 = Or(x=w2115, y=w2116) -> (x .or. y?=w2114:bool)
                      n1101 = for {
                        tunnel: w2118 -> [w2124] mode=indexing
                        tunnel: w2119 -> [w2123] mode=indexing
                        tunnel: w2117 -> [w2120] mode=indexing
                        tunnel: w2114 -> [w2122]
                        tunnel: w2113 -> [w2121]
                        n1102 = call "Gestione grafico.vi"("Array"=w2123, "colori grafico"=w2121, "PLOT LEGEND"=w2120, "graph ref"=w2124, "Update annotation?"=w2122) -> ("Array out"=w2125:cluster{"X":dbl[], "Y":dbl[]}[])  [unwired: 5 in]
                        n1103 = property class="XYGraph (strict)"(reference=w2124, "Value"=w2125) -> ()  [unwired: 1 in, 2 out]
                      }
                    }
                    frame #1 {
                      n1104 = local write "update annotation"(FALSE ("update annotation")) -> ()
                    }
                  }
                  n1105 = feedback #7() -> (w2091:T3[])  [unwired: 1 in]
                  n1106 = feedback-in #7(w2092) -> ()
                  n1107 = feedback #8() -> (w2089:variant)  [unwired: 1 in]
                  n1108 = feedback-in #8(w2090) -> ()
                  n1109 = Not Equal?(x=w2092, y=w2091) -> (x != y?=w2088:bool)
                  n1110 = Not Equal?(x=w2090, y=w2089) -> (x != y?=w2087:bool)
                  n1111 = Compound Arithmetic op=OR(w2088, w2087) -> (w2086:bool)
                }
              }
            }
            n1112 = control-ref of="PLOT LEGEND T-DT"() -> ()  [unwired: 1 out]
            n1113 = control-ref of="Cluster"() -> ()  [unwired: 1 out]
          }
          frame Enabled {
          }
        }
      }
      frame "Set x scale" {
        n1114 = local write "carica grafici"(FALSE ("carica grafici")) -> ()
        n1115 = property on="ProvaT-DT" class="XYGraph (strict)"() -> ("XScale.Maximum"=w2136:dbl)  [unwired: 2 in, 2 out]
        n1116 = property on="ProvaT-TC" class="XYGraph (strict)"() -> ("XScale.Maximum"=w2135:dbl)  [unwired: 2 in, 2 out]
        n1117 = Build Array(w2136, w2135) -> (w2137:dbl[])
        n1118 = Array Max & Min(array=w2137) -> (max value=w2134:dbl)  [unwired: 3 out]
        n1119 = property on="ProvaT-DT" class="XYGraph (strict)"("XScale.Maximum"=w2134) -> ()  [unwired: 2 in, 2 out]
        n1120 = property on="ProvaT-TC" class="XYGraph (strict)"("XScale.Maximum"=w2134) -> ()  [unwired: 2 in, 2 out]
      }
      frame "REPORT EXCEL" {
        n1121 = Get Date/Time In Seconds() -> (seconds since 1Jan1904=w2158:timestamp)
        n1122 = property on="SCELTA MODELLO XLS" class="LstBox (strict)"() -> ("Item Names"=w2151:string[], "Value"=w2152:i32)  [unwired: 2 in, 2 out]
        n1123 = property on="Dati collaudo principale" class="MCListbox (strict)"() -> ("ItemNames"=w2169:string[][])  [unwired: 2 in, 2 out]
        n1124 = Get Date/Time String(seconds (now)=w2158) -> (date string=w2159:string, time string=w2164:string)  [unwired: 2 in]
        n1125 = local read "trifase?"() -> (w2175:bool)
        n1126 = property on="Criteri di salvataggio report" class="MCListbox (strict)"() -> ("ItemNames"=w2171:string[][])  [unwired: 2 in, 2 out]
        n1127 = property on="Percorso e nome di DEFAULT" class="MCListbox (strict)"() -> ("ItemNames"=w2170:string[][])  [unwired: 2 in, 2 out]
        n1128 = Index Array(array=w2169, index (row)=3, index (col)=1 ("disabled index (col)")) -> (element=w2166:string)
        n1129 = Index Array(array=w2151, index=w2152) -> (element=w2143:string)
        n1130 = disable-structure shown="Disabled" {
          frame Disabled {
            n1131 = local read "COLLAUDO PRINCIPALE"() -> ()  [unwired: 1 out]
            n1132 = local read "Percorso report di DEFAULT"() -> ()  [unwired: 1 out]
          }
          frame Enabled {
          }
        }
        n1133 = Boolean To (0,1)(Boolean=w2175) -> (0, 1=w2174:i16)
        n1134 = call "Ora sotto data.vi"("Array in"=w2172) -> ("Array out"=w2178:string[][])  [unwired: 10 in]
        n1135 = Search and Replace String(replace all?=TRUE ("replace all? (F)"), input string=w2164, search string=":") -> (result string=w2155:string)  [unwired: 5 in, 3 out]
        n1136 = Index Array(array=w2176, index=w2174) -> (element=w2173:T19)
        n1137 = Search and Replace String(replace all?=TRUE ("replace all? (F)"), input string=w2159, search string="/") -> (result string=w2157:string)  [unwired: 5 in, 3 out]
        n1138 = Concatenate Strings(w2166, "_BFRN_" ("string"), w2157, "_" ("string"), w2155) -> (w2154:string)
        n1139 = call "Percorso e nome report.vi"("Default"=w2170, "Criteri"=w2171, "DT"=w2172) -> ("path gestionale"=w2146:path, "path Standard"=w2145:path, "Nome file"=w2150:string)  [unwired: 6 in]
        n1140 = Search and Replace String(input string=w2143, search string="GESTIONALE") -> (number of replacements=w2148:i32)  [unwired: 6 in, 3 out]
        n1141 = control-ref of="Slide"() -> (w2179:refnum<vi>)
        n1142 = Greater Than 0?(x=w2148) -> (x > 0?=w2147:bool)
        n1143 = Select(t=w2146, s=w2147, f=w2145) -> (s? t:f=w2144:path)
        n1144 = case shown="False" w2153 {
          tunnel: "*.xls" ("DNL") -> [w2191 _]
          tunnel: [w2190 w2193] -> w2181
          tunnel: [w2189 _] -> w2180
          tunnel: w2144 -> [w2188 w2199]
          tunnel: w2154 -> [_ w2196]
          tunnel: w2150 -> [w2187 _]
          frame False {
            n1145 = call "File Dialog3"("start path"=w2188, "default name"=w2187, "pattern (all files)"=w2191) -> ("selected path"=w2190:path, "cancelled"=w2189:bool, "error out"=w2192:errorcluster)  [unwired: 4 in, 6 out]
            n1146 = call <vilib>:"Clear Errors.vi"("error in (no error)"=w2192) -> ()  [unwired: 5 in, 2 out]
          }
          frame True {
            n1147 = Path To String(path=w2199) -> (string=w2198:string)
            n1148 = Concatenate Strings(w2198, "\\" ("string"), w2196, ".xls" ("string")) -> (w2194:string)
            n1149 = String To Path(string=w2194) -> (path=w2193:path)
          }
        }
        n1150 = case shown="False" w2180 {
          tunnel: w2184 -> [w2209 _]
          tunnel: w2178 -> [w2208 _]
          tunnel: w2181 -> [w2207 _]
          tunnel: w2179 -> [w2206 _]
          tunnel: w2173 -> [_ _]
          tunnel: w2153 -> [w2201 _]
          tunnel: w2153 -> [w2202 _]
          tunnel: w2143 -> [w2200 _]
          frame False {
            n1151 = property on="REPORT EXCEL" class="Bool (strict)"("Visible"=FALSE) -> ()  [unwired: 2 in, 2 out]
            n1152 = stacked-sequence {
              seq-local: [w2231 _ _ _] -> [_ _ w2324 w2962]
              tunnel: w2209 -> [_ _ w2372 _]
              tunnel: w2208 -> [_ _ w2363 _]
              tunnel: w2207 -> [_ _ w2333 _]
              tunnel: w2206 -> [w2232 w2320 w2390 w2964]
              tunnel: [_ _ _ w2963] -> w2205
              tunnel: w2201 -> [_ w2319 w2325 _]
              tunnel: w2201 -> [w2212 _ _ _]
              tunnel: w2200 -> [w2210 _ _ _]
              frame #0 {
                n1153 = case shown="False" w2212 {
                  tunnel: [w2234 _] -> w2231
                  frame False {
                    n1154 = control-ref of="Array Grafici A VUOTO"() -> (w2241:refnum<vi>)
                    n1155 = control-ref of="Array Grafici A CARICO"() -> (w2236:refnum<vi>)
                    n1156 = control-ref of="Array Grafici TERMICA"() -> (w2237:refnum<vi>)
                    n1157 = control-ref of="Array Grafici CMECC"() -> (w2238:refnum<vi>)
                    n1158 = control-ref of="Array Grafici ROTBLOCC"() -> (w2239:refnum<vi>)
                    n1159 = control-ref of="Array Grafici GENERICA"() -> (w2240:refnum<vi>)
                    n1160 = Build Array(w2241, w2236, w2237, w2238, w2239, w2240) -> (w2235:refnum<vi>[])
                    n1161 = for {
                      tunnel: w2235 -> [w2248] mode=indexing
                      tunnel: [w2242] -> w2234 mode=concatenating
                      i -> [w2243]
                      n1162 = property class="Arr"(reference=w2248) -> ("Value"=w2247:variant)  [unwired: 1 in, 2 out]
                      n1163 = Build Array(T8 {"2D Picture"=bytes[771184], "Aggiungi grafico"=FALSE, "Settings grafico"=FALSE, "Elimina grafico"=FALSE, "scelta grafico A VUOTO 2"=0, "Esporta xls"={"Esporta?"=TRUE, "Impostazioni esport."={"position (Excel)"={"row"=8, "column"=2}, "Nome foglio (Excel)"="", "bookmark (Word)"=""}, "Zoom "=1.0, "Ruota immagine"=enum."rotate 0°"}} ("Cluster")) -> (w2245:T8[])
                      n1164 = Variant To Data(type=w2245, Variant=w2247) -> (data=w2244:T8[])  [unwired: 1 in, 1 out]
                      n1165 = for {
                        tunnel: w2244 -> [w2273] mode=indexing
                        tunnel: w2243 -> [w2262]
                        tunnel: [w2251] -> w2242 mode=indexing if=w2250
                        i -> [w2261]
                        n1166 = Unbundle By Name(w2273) -> ("2D Picture"=w2272:picture, "Esporta xls.Esporta?"=w2250:bool, "Esporta xls.Zoom"=w2249:sgl, "Esporta xls.Ruota immagine"=w2265:T35, "Esporta xls.Impostazioni esport."=w2252:T36)
                        n1167 = Number To Decimal String(number=w2262) -> (decimal integer string=w2259:string)  [unwired: 1 in]
                        n1168 = Number To Decimal String(number=w2261) -> (decimal integer string=w2260:string)  [unwired: 1 in]
                        n1169 = Concatenate Strings("Report\\Immagini temp\\" ("name or relative path"), w2259, w2260, ".jpeg" ("string")) -> (w2255:string)
                        n1170 = call <vilib>:"Picture to Pixmap.vi"("picture"=w2272) -> ("image data"=w2264:T28)  [unwired: 9 in, 1 out]
                        n1171 = call <vilib>:"Unflatten Pixmap.vi"("image data"=w2264) -> ("24-bit pixmap"=w2269:u32[][], "colors"=w2271:u32[], "top left"=w2267:cluster{"x":i16, "y":i16}, "mask"=w2270:u8[])  [unwired: 4 in, 3 out]
                        n1172 = case shown="\"rotate 270°\"" w2265 {
                          tunnel: w2269 -> [w2283 w2286 w2288 w2297 w2310]
                          tunnel: [w2282 w2286 w2290 w2298 w2306] -> w2268
                          tunnel: w2267 -> [w2281 w2287 w2294 w2303 w2311]
                          tunnel: [w2281 w2287 w2291 w2300 w2309] -> w2266
                          frame "miror" {
                            n1173 = for {
                              tunnel: w2283 -> [w2285] mode=indexing
                              tunnel: [w2284] -> w2282 mode=indexing
                              n1174 = Reverse 1D Array(array=w2285) -> (reversed array=w2284:u32[])
                            }
                          }
                          frame "rotate 0°", Default {
                          }
                          frame "rotate 90°" {
                            n1175 = Transpose 2D Array(2D array=w2288) -> (transposed array=w2289:u32[][])
                            n1176 = Unbundle By Name(w2294) -> ("x"=w2293:i16, "y"=w2292:i16)
                            n1177 = for {
                              tunnel: w2289 -> [w2296] mode=indexing
                              tunnel: [w2295] -> w2290 mode=indexing
                              n1178 = Reverse 1D Array(array=w2296) -> (reversed array=w2295:u32[])
                            }
                            n1179 = Bundle By Name(cluster=w2294, "y"=w2293, "y"=w2292) -> (w2291:cluster{"x":i16, "y":i16})
                          }
                          frame "rotate 270°" {
                            # "90"
                            n1180 = for {
                              tunnel: w2297 -> [w2305] mode=indexing
                              tunnel: [w2304] -> w2299 mode=indexing
                              n1181 = Reverse 1D Array(array=w2305) -> (reversed array=w2304:u32[])
                            }
                            n1182 = Unbundle By Name(w2303) -> ("x"=w2302:i16, "y"=w2301:i16)
                            n1183 = Bundle By Name(cluster=w2303, "y"=w2302, "y"=w2301) -> (w2300:cluster{"x":i16, "y":i16})
                            n1184 = Transpose 2D Array(2D array=w2299) -> (transposed array=w2298:u32[][])
                          }
                          frame "rotate 180°" {
                            # "180"
                            n1185 = for {
                              tunnel: w2310 -> [w2318] mode=indexing
                              tunnel: [w2317] -> w2312 mode=indexing
                              n1186 = Reverse 1D Array(array=w2318) -> (reversed array=w2317:u32[])
                            }
                            n1187 = Unbundle By Name(w2311) -> ("x"=w2314:i16, "y"=w2313:i16)
                            n1188 = Transpose 2D Array(2D array=w2312) -> (transposed array=w2307:u32[][])
                            n1189 = Bundle By Name(cluster=w2311, "y"=w2314, "y"=w2313) -> (w2309:cluster{"x":i16, "y":i16})
                            n1190 = for {
                              tunnel: w2307 -> [w2316] mode=indexing
                              tunnel: [w2315] -> w2308 mode=indexing
                              n1191 = Reverse 1D Array(array=w2316) -> (reversed array=w2315:u32[])
                            }
                            n1192 = Transpose 2D Array(2D array=w2308) -> (transposed array=w2306:u32[][])
                          }
                        }
                        n1193 = call <vilib>:"Application Directory.vi"() -> ("Application Directory"=w2256:path)
                        n1194 = Build Path(base path=w2256, name or relative path=w2255) -> (appended path=w2254:path)
                        n1195 = call <vilib>:"Flatten Pixmap.vi"("mask"=w2270, "colors"=w2271, "top left"=w2266, "24-bit pixmap"=w2268) -> ("image data"=w2263:T28)  [unwired: 7 in]
                        n1196 = case shown="False" w2250 {
                          tunnel: w2263 -> [_ w2278]
                          tunnel: w2254 -> [_ w2277]
                          tunnel: [_ w2275] -> w2253
                          tunnel: w2249 -> [_ w2274]
                          frame False {
                          }
                          frame True {
                            n1197 = control-ref of="picture T Dt"() -> (w2279:refnum<vi>)
                            n1198 = call "Zoom immagine grafici.vi"("image data in"=w2278, "Zoom Factor"=w2274, "Picture in"=w2279) -> ("image data out"=w2280:T28)  [unwired: 8 in]
                            n1199 = call <vilib>:"Write JPEG File.vi"("quality (80)"=100, "image data"=w2280, "path to JPEG file"=w2277) -> ("path"=w2275:path)  [unwired: 7 in, 1 out]
                          }
                        }
                        n1200 = Bundle("path"=w2253, "Impostazioni esport."=w2252) -> (w2251:T37)  [unwired: 1 in]
                      }
                    }
                  }
                  frame True {
                  }
                }
                n1201 = property class="Slide (strict)"(reference=w2232, "Value"=5.0) -> ()  [unwired: 1 in, 2 out]
                n1202 = global read "Global percorso impostazioni.vi" "Path settings"() -> (w2229:path)
                n1203 = Search and Replace String(input string=w2210, search string=".", replace string="_" ("replace string (\"\")")) -> (result string=w2226:string)  [unwired: 5 in, 3 out]
                n1204 = Build Path(base path=w2229, name or relative path="Settings grafici") -> (appended path=w2222:path)
                n1205 = Concatenate Strings("IMPOSTAZIONI_ESPORTAZIONE_", w2226) -> (w2227:string)
                n1206 = Build Path(base path=w2222, name or relative path=w2227) -> (appended path=w2228:path)
                n1207 = Open/Create/Replace File(file path (use dialog)=w2228, operation (0:open)=T14."open") -> (refnum out=w2214:refnum<file>, error out=w2216:errorcluster)  [unwired: 4 in, 1 out]
                n1208 = Read from Binary File(5:T20 {"Nome fogli"=[], "Nome fogli GENERICHE"=[]} ("output cluster"), 8:w2216, 11:w2214) -> (0:w2217:errorcluster, 2:w2218:T20, 3:w2215:refnum<file>)  [unwired: 3 in, 1 out]
                n1209 = Unbundle By Name(w2218) -> ("Nome fogli"=w2220:T13, "Nome fogli GENERICHE"=w2219:T12)
                n1210 = Close File(refnum=w2215, error in=w2217) -> (error out=w2230:errorcluster)  [unwired: 1 out]
                n1211 = call <vilib>:"Clear Errors.vi"("error in (no error)"=w2230) -> ()  [unwired: 5 in, 2 out]
                n1212 = local write "Nome fogli GENERICHE"(w2219) -> ()
                n1213 = local write "Nome fogli"(w2220) -> ()
              }
              frame #1 {
                n1214 = property class="Slide (strict)"(reference=w2320, "Value"=10.0) -> ()  [unwired: 1 in, 2 out]
                n1215 = case shown="False" w2319 {
                  frame False {
                    n1216 = Wait (ms)(milliseconds to wait=u32 2000) -> ()  [unwired: 1 out]
                  }
                  frame True {
                  }
                }
              }
              frame #2 {
                n1217 = property on="SCELTA MODELLO XLS" class="LstBox (strict)"() -> ("Item Names"=w2358:string[], "Value"=w2357:i32)  [unwired: 2 in, 2 out]
                n1218 = local read "Cartella modello"() -> (w2359:path)
                n1219 = local read "sep. decimale numeri esportati"() -> (w2370:enum16{"Virgola", "Punto"})
                n1220 = Index Array(array=w2358, index=w2357) -> (element=w2356:string)
                n1221 = Build Path(base path=w2359, name or relative path=w2356) -> (appended path=w2355:path)
                n1222 = property class="Slide (strict)"(reference=w2390, "Value"=20.0) -> (reference out=w2387:refnum<vi>)  [unwired: 1 in, 1 out]
                n1223 = call <vilib>:"New Report.vi"("window state (normal)"=T23."no change", "report type"=T24."Excel", "template (empty)"=w2355) -> ("report out"=w2375:refnum<class "NI_report.lvclass">, "error out"=w2367:errorcluster)  [unwired: 11 in]
                n1224 = local read "COLLAUDI DI CONFRONTO"() -> (w2352:string[])
                n1225 = local read "Descrizione"() -> (w2351:string[])
                n1226 = local read "COLLAUDO PRINCIPALE"() -> (w2354:string)
                n1227 = local read "Descrizione princ"() -> (w2353:string)
                n1228 = for {
                  tunnel: w2352 -> [w2439] mode=indexing
                  tunnel: w2351 -> [w2438] mode=indexing
                  tunnel: [w2437] -> w2349 mode=indexing
                  tunnel: string[] ["CONFRONTO[1]", "CONFRONTO[2]", "CONFRONTO[3]", "CONFRONTO[4]", "CONFRONTO[5]"] -> [w2436] mode=indexing
                  n1229 = Build Array(w2436, w2439, w2438) -> (w2437:string[])
                }
                n1230 = local read "TABELLA GENERICA"() -> (w2360:i16)
                n1231 = property class="Slide (strict)"(reference=w2387, error in=w2367, "Value"=20.0) -> (reference out=w2385:refnum<vi>)  [unwired: 1 out]
                n1232 = Build Array("PRINCIPALE[0]" ("element"), w2354, w2353) -> (w2350:string[])
                n1233 = Build Array (concatenate)(w2350, w2349) -> (w2348:string[][])
                n1234 = for {
                  tunnel: "Nome fogli" -> [w2452] mode=indexing
                  shift-right: [w2449] -> w2374
                  shift-left: w2375 -> [w2450]
                  shift-right: [w2447] -> w2366
                  shift-left: w2367 -> [w2448]
                  tunnel: w2370 -> [w2444]
                  tunnel: w2372 -> [w2443]
                  tunnel: w2363 -> [w2442]
                  tunnel: w2348 -> [w2440]
                  n1235 = Unbundle By Name(w2452) -> ("Nome prova"=w2451:T38, "Nome foglio nascosto xls"=w2446:string, "Cella iniziale"=w2445:cluster{"row":i32, "column":i32})
                  n1236 = local read "ETICHETTE"() -> (w2441:string[])
                  n1237 = case shown="\"RES INIZIO PROVA A CARICO\"" w2451 {
                    tunnel: w2450 -> [w2459 w2476 w2509 w2542 w2575 w2608 w2641 w2674 w2707 w2742 w2775 w2808 w2841 w2874 w2907 w2932 w2943]
                    tunnel: [w2458 w2475 w2508 w2541 w2574 w2607 w2640 w2673 w2706 w2741 w2774 w2807 w2840 w2873 w2906 w2931 w2938] -> w2449
                    tunnel: w2448 -> [w2457 w2474 w2507 w2540 w2573 w2606 w2639 w2672 w2705 w2740 w2773 w2806 w2839 w2872 w2905 w2930 w2942]
                    tunnel: [w2456 w2473 w2506 w2539 w2572 w2605 w2638 w2671 w2704 w2739 w2772 w2805 w2838 w2871 w2904 w2929 w2939] -> w2447
                    tunnel: w2446 -> [w2455 w2472 w2505 w2538 w2571 w2604 w2637 w2670 w2703 w2738 w2771 w2804 w2837 w2870 w2903 w2927 w2941]
                    tunnel: w2445 -> [w2454 w2471 w2504 w2537 w2570 w2603 w2636 w2669 w2702 w2737 w2770 w2803 w2836 w2869 w2902 w2928 w2940]
                    tunnel: w2444 -> [_ w2470 w2503 w2536 w2569 w2602 w2635 w2668 w2701 w2736 w2769 w2802 w2835 w2868 w2901 _ w2935]
                    tunnel: w2441 -> [_ w2469 w2502 w2535 w2568 w2601 w2634 w2667 w2700 w2727 w2768 w2801 w2834 w2867 w2900 _ _]
                    tunnel: w2443 -> [_ w2466 w2499 w2532 w2565 w2598 w2631 w2664 w2697 w2733 w2765 w2798 w2831 w2864 w2897 _ _]
                    tunnel: w2442 -> [w2453 _ _ _ _ _ _ _ _ _ _ _ _ _ _ _ _]
                    tunnel: w2440 -> [_ _ _ _ _ _ _ _ _ _ _ _ _ _ _ w2926 _]
                    frame "DATI BOLLETTINO", Default {
                      n1238 = call <vilib>:"Excel Get Worksheet.vi"("report in"=w2459, "error in (no error)"=w2457, "name (\"\")"=w2455) -> ("report out"=w2460:refnum<class "NI_report.lvclass">, "error out"=w2461:errorcluster)  [unwired: 11 in]
                      n1239 = call-poly <vilib>:"Excel Easy Table.vi"("report in"=w2460, "start (0, 0)"=w2454, "text data"=w2453, "error in (no error)"=w2461) -> ("report out"=w2458:refnum<class "NI_report.lvclass">, "error out"=w2456:errorcluster)  [unwired: 7 in, 3 out]
                    }
                    frame "RESISTENZE FREDDO" {
                      n1240 = Unbundle By Name(w2466) -> ("Res freddo resistomat"=w2464:string[][])
                      n1241 = call <vilib>:"Excel Get Worksheet.vi"("report in"=w2476, "error in (no error)"=w2474, "name (\"\")"=w2472) -> ("report out"=w2477:refnum<class "NI_report.lvclass">, "error out"=w2478:errorcluster)  [unwired: 11 in]
                      n1242 = call "Fitra per tabella.vi"("TAB"=1, "dati in"=w2464) -> ("dati out"=w2463:string[][])  [unwired: 9 in]
                      n1243 = Build Array (concatenate)(string[] ["RES FREDDO"] ("element"), w2469, w2463) -> (w2467:string[][])
                      n1244 = case shown="\"Virgola\", Default" w2470 {
                        tunnel: w2467 -> [w2480 w2488]
                        tunnel: [w2479 w2487] -> w2468
                        frame "Virgola", Default {
                          n1245 = for {
                            tunnel: w2480 -> [w2482] mode=indexing
                            tunnel: [w2481] -> w2479 mode=indexing
                            n1246 = for {
                              tunnel: w2482 -> [w2486] mode=indexing
                              tunnel: [w2483] -> w2481 mode=indexing
                              n1247 = Search and Replace String(input string=w2486, search string=",", replace string="." ("search string")) -> (result string=w2483:string)  [unwired: 5 in, 3 out]
                            }
                          }
                        }
                        frame "Punto" {
                          n1248 = for {
                            tunnel: w2488 -> [w2490] mode=indexing
                            tunnel: [w2489] -> w2487 mode=indexing
                            n1249 = for {
                              tunnel: w2490 -> [w2494] mode=indexing
                              tunnel: [w2491] -> w2489 mode=indexing
                              n1250 = Search and Replace String(input string=w2494, search string=".", replace string="," ("search string")) -> (result string=w2491:string)  [unwired: 5 in, 3 out]
                            }
                          }
                        }
                      }
                      n1251 = call-poly <vilib>:"Excel Easy Table.vi"("report in"=w2477, "start (0, 0)"=w2471, "text data"=w2468, "error in (no error)"=w2478) -> ("report out"=w2475:refnum<class "NI_report.lvclass">, "error out"=w2473:errorcluster)  [unwired: 7 in, 3 out]
                    }
                    frame "RIGA DATI I SPUNTO" {
                      n1252 = local read "TABELLA A ROT BLOCC"() -> (w2495:i16)
                      n1253 = Unbundle By Name(w2499) -> ("Riga Ispunto"=w2497:string[][])
                      n1254 = call <vilib>:"Excel Get Worksheet.vi"("report in"=w2509, "error in (no error)"=w2507, "name (\"\")"=w2505) -> ("report out"=w2510:refnum<class "NI_report.lvclass">, "error out"=w2511:errorcluster)  [unwired: 11 in]
                      n1255 = call "Fitra per tabella.vi"("TAB"=w2495, "dati in"=w2497) -> ("dati out"=w2496:string[][])  [unwired: 9 in]
                      n1256 = Build Array (concatenate)(string[] ["I SPUNTO"] ("element"), w2502, w2496) -> (w2500:string[][])
                      n1257 = case shown="\"Virgola\", Default" w2503 {
                        tunnel: w2500 -> [w2513 w2521]
                        tunnel: [w2512 w2520] -> w2501
                        frame "Virgola", Default {
                          n1258 = for {
                            tunnel: w2513 -> [w2515] mode=indexing
                            tunnel: [w2514] -> w2512 mode=indexing
                            n1259 = for {
                              tunnel: w2515 -> [w2519] mode=indexing
                              tunnel: [w2516] -> w2514 mode=indexing
                              n1260 = Search and Replace String(input string=w2519, search string=",", replace string="." ("search string")) -> (result string=w2516:string)  [unwired: 5 in, 3 out]
                            }
                          }
                        }
                        frame "Punto" {
                          n1261 = for {
                            tunnel: w2521 -> [w2523] mode=indexing
                            tunnel: [w2522] -> w2520 mode=indexing
                            n1262 = for {
                              tunnel: w2523 -> [w2527] mode=indexing
                              tunnel: [w2524] -> w2522 mode=indexing
                              n1263 = Search and Replace String(input string=w2527, search string=".", replace string="," ("search string")) -> (result string=w2524:string)  [unwired: 5 in, 3 out]
                            }
                          }
                        }
                      }
                      n1264 = call-poly <vilib>:"Excel Easy Table.vi"("report in"=w2510, "start (0, 0)"=w2504, "text data"=w2501, "error in (no error)"=w2511) -> ("report out"=w2508:refnum<class "NI_report.lvclass">, "error out"=w2506:errorcluster)  [unwired: 7 in, 3 out]
                    }
                    frame "DATI ROTORE BLOCCATO" {
                      n1265 = local read "TABELLA A ROT BLOCC"() -> (w2528:i16)
                      n1266 = Unbundle By Name(w2532) -> ("Rbloccato"=w2530:string[][])
                      n1267 = call <vilib>:"Excel Get Worksheet.vi"("report in"=w2542, "error in (no error)"=w2540, "name (\"\")"=w2538) -> ("report out"=w2543:refnum<class "NI_report.lvclass">, "error out"=w2544:errorcluster)  [unwired: 11 in]
                      n1268 = call "Fitra per tabella.vi"("TAB"=w2528, "dati in"=w2530) -> ("dati out"=w2529:string[][])  [unwired: 9 in]
                      n1269 = Build Array (concatenate)(string[] ["ROTORE BLOCCATO"] ("element"), w2535, w2529) -> (w2533:string[][])
                      n1270 = case shown="\"Virgola\", Default" w2536 {
                        tunnel: w2533 -> [w2546 w2554]
                        tunnel: [w2545 w2553] -> w2534
                        frame "Virgola", Default {
                          n1271 = for {
                            tunnel: w2546 -> [w2548] mode=indexing
                            tunnel: [w2547] -> w2545 mode=indexing
                            n1272 = for {
                              tunnel: w2548 -> [w2552] mode=indexing
                              tunnel: [w2549] -> w2547 mode=indexing
                              n1273 = Search and Replace String(input string=w2552, search string=",", replace string="." ("search string")) -> (result string=w2549:string)  [unwired: 5 in, 3 out]
                            }
                          }
                        }
                        frame "Punto" {
                          n1274 = for {
                            tunnel: w2554 -> [w2556] mode=indexing
                            tunnel: [w2555] -> w2553 mode=indexing
                            n1275 = for {
                              tunnel: w2556 -> [w2560] mode=indexing
                              tunnel: [w2557] -> w2555 mode=indexing
                              n1276 = Search and Replace String(input string=w2560, search string=".", replace string="," ("search string")) -> (result string=w2557:string)  [unwired: 5 in, 3 out]
                            }
                          }
                        }
                      }
                      n1277 = call-poly <vilib>:"Excel Easy Table.vi"("report in"=w2543, "start (0, 0)"=w2537, "text data"=w2534, "error in (no error)"=w2544) -> ("report out"=w2541:refnum<class "NI_report.lvclass">, "error out"=w2539:errorcluster)  [unwired: 7 in, 3 out]
                    }
                    frame "RES INIZIO PROVA VUOTO" {
                      n1278 = local read "TABELLA A VUOTO"() -> (w2561:i16)
                      n1279 = Unbundle By Name(w2565) -> ("Res ini vuoto"=w2563:string[][])
                      n1280 = call <vilib>:"Excel Get Worksheet.vi"("report in"=w2575, "error in (no error)"=w2573, "name (\"\")"=w2571) -> ("report out"=w2576:refnum<class "NI_report.lvclass">, "error out"=w2577:errorcluster)  [unwired: 11 in]
                      n1281 = call "Fitra per tabella.vi"("TAB"=w2561, "dati in"=w2563) -> ("dati out"=w2562:string[][])  [unwired: 9 in]
                      n1282 = Build Array (concatenate)(string[] ["RES INIZ VUOTO"] ("element"), w2568, w2562) -> (w2566:string[][])
                      n1283 = case shown="\"Virgola\", Default" w2569 {
                        tunnel: w2566 -> [w2579 w2587]
                        tunnel: [w2578 w2586] -> w2567
                        frame "Virgola", Default {
                          n1284 = for {
                            tunnel: w2579 -> [w2581] mode=indexing
                            tunnel: [w2580] -> w2578 mode=indexing
                            n1285 = for {
                              tunnel: w2581 -> [w2585] mode=indexing
                              tunnel: [w2582] -> w2580 mode=indexing
                              n1286 = Search and Replace String(input string=w2585, search string=",", replace string="." ("search string")) -> (result string=w2582:string)  [unwired: 5 in, 3 out]
                            }
                          }
                        }
                        frame "Punto" {
                          n1287 = for {
                            tunnel: w2587 -> [w2589] mode=indexing
                            tunnel: [w2588] -> w2586 mode=indexing
                            n1288 = for {
                              tunnel: w2589 -> [w2593] mode=indexing
                              tunnel: [w2590] -> w2588 mode=indexing
                              n1289 = Search and Replace String(input string=w2593, search string=".", replace string="," ("search string")) -> (result string=w2590:string)  [unwired: 5 in, 3 out]
                            }
                          }
                        }
                      }
                      n1290 = call-poly <vilib>:"Excel Easy Table.vi"("report in"=w2576, "start (0, 0)"=w2570, "text data"=w2567, "error in (no error)"=w2577) -> ("report out"=w2574:refnum<class "NI_report.lvclass">, "error out"=w2572:errorcluster)  [unwired: 7 in, 3 out]
                    }
                    frame "RES FINE PROVA VUOTO" {
                      n1291 = local read "TABELLA A VUOTO"() -> (w2594:i16)
                      n1292 = Unbundle By Name(w2598) -> ("Res fin vuoto"=w2596:string[][])
                      n1293 = call <vilib>:"Excel Get Worksheet.vi"("report in"=w2608, "error in (no error)"=w2606, "name (\"\")"=w2604) -> ("report out"=w2609:refnum<class "NI_report.lvclass">, "error out"=w2610:errorcluster)  [unwired: 11 in]
                      n1294 = call "Fitra per tabella.vi"("TAB"=w2594, "dati in"=w2596) -> ("dati out"=w2595:string[][])  [unwired: 9 in]
                      n1295 = Build Array (concatenate)(string[] ["RES FINE VUOTO"] ("element"), w2601, w2595) -> (w2599:string[][])
                      n1296 = case shown="\"Virgola\", Default" w2602 {
                        tunnel: w2599 -> [w2612 w2620]
                        tunnel: [w2611 w2619] -> w2600
                        frame "Virgola", Default {
                          n1297 = for {
                            tunnel: w2612 -> [w2614] mode=indexing
                            tunnel: [w2613] -> w2611 mode=indexing
                            n1298 = for {
                              tunnel: w2614 -> [w2618] mode=indexing
                              tunnel: [w2615] -> w2613 mode=indexing
                              n1299 = Search and Replace String(input string=w2618, search string=",", replace string="." ("search string")) -> (result string=w2615:string)  [unwired: 5 in, 3 out]
                            }
                          }
                        }
                        frame "Punto" {
                          n1300 = for {
                            tunnel: w2620 -> [w2622] mode=indexing
                            tunnel: [w2621] -> w2619 mode=indexing
                            n1301 = for {
                              tunnel: w2622 -> [w2626] mode=indexing
                              tunnel: [w2623] -> w2621 mode=indexing
                              n1302 = Search and Replace String(input string=w2626, search string=".", replace string="," ("search string")) -> (result string=w2623:string)  [unwired: 5 in, 3 out]
                            }
                          }
                        }
                      }
                      n1303 = call-poly <vilib>:"Excel Easy Table.vi"("report in"=w2609, "start (0, 0)"=w2603, "text data"=w2600, "error in (no error)"=w2610) -> ("report out"=w2607:refnum<class "NI_report.lvclass">, "error out"=w2605:errorcluster)  [unwired: 7 in, 3 out]
                    }
                    frame "DATI PROVA A VUOTO" {
                      n1304 = Unbundle By Name(w2631) -> ("A vuoto"=w2629:string[][])
                      n1305 = local read "TABELLA A VUOTO"() -> (w2628:i16)
                      n1306 = call <vilib>:"Excel Get Worksheet.vi"("report in"=w2641, "error in (no error)"=w2639, "name (\"\")"=w2637) -> ("report out"=w2642:refnum<class "NI_report.lvclass">, "error out"=w2643:errorcluster)  [unwired: 11 in]
                      n1307 = call "Fitra per tabella.vi"("TAB"=w2628, "dati in"=w2629) -> ("dati out"=w2627:string[][])  [unwired: 9 in]
                      n1308 = Build Array (concatenate)(string[] ["PROVA VUOTO"] ("element"), w2634, w2627) -> (w2632:string[][])
                      n1309 = case shown="\"Virgola\", Default" w2635 {
                        tunnel: w2632 -> [w2645 w2653]
                        tunnel: [w2644 w2652] -> w2633
                        frame "Virgola", Default {
                          n1310 = for {
                            tunnel: w2645 -> [w2647] mode=indexing
                            tunnel: [w2646] -> w2644 mode=indexing
                            n1311 = for {
                              tunnel: w2647 -> [w2651] mode=indexing
                              tunnel: [w2648] -> w2646 mode=indexing
                              n1312 = Search and Replace String(input string=w2651, search string=",", replace string="." ("search string")) -> (result string=w2648:string)  [unwired: 5 in, 3 out]
                            }
                          }
                        }
                        frame "Punto" {
                          n1313 = for {
                            tunnel: w2653 -> [w2655] mode=indexing
                            tunnel: [w2654] -> w2652 mode=indexing
                            n1314 = for {
                              tunnel: w2655 -> [w2659] mode=indexing
                              tunnel: [w2656] -> w2654 mode=indexing
                              n1315 = Search and Replace String(input string=w2659, search string=".", replace string="," ("search string")) -> (result string=w2656:string)  [unwired: 5 in, 3 out]
                            }
                          }
                        }
                      }
                      n1316 = call-poly <vilib>:"Excel Easy Table.vi"("report in"=w2642, "start (0, 0)"=w2636, "text data"=w2633, "error in (no error)"=w2643) -> ("report out"=w2640:refnum<class "NI_report.lvclass">, "error out"=w2638:errorcluster)  [unwired: 7 in, 3 out]
                    }
                    frame "RES INIZIO PROVA A CARICO" {
                      n1317 = local read "TABELLA A CARICO"() -> (w2660:i16)
                      n1318 = Unbundle By Name(w2664) -> ("Res ini carico"=w2662:string[][])
                      n1319 = call <vilib>:"Excel Get Worksheet.vi"("report in"=w2674, "error in (no error)"=w2672, "name (\"\")"=w2670) -> ("report out"=w2675:refnum<class "NI_report.lvclass">, "error out"=w2676:errorcluster)  [unwired: 11 in]
                      n1320 = call "Fitra per tabella.vi"("TAB"=w2660, "dati in"=w2662) -> ("dati out"=w2661:string[][])  [unwired: 9 in]
                      n1321 = Build Array (concatenate)(string[] ["RES INIZ CARICO"] ("element"), w2667, w2661) -> (w2665:string[][])
                      n1322 = case shown="\"Virgola\", Default" w2668 {
                        tunnel: w2665 -> [w2678 w2686]
                        tunnel: [w2677 w2685] -> w2666
                        frame "Virgola", Default {
                          n1323 = for {
                            tunnel: w2678 -> [w2680] mode=indexing
                            tunnel: [w2679] -> w2677 mode=indexing
                            n1324 = for {
                              tunnel: w2680 -> [w2684] mode=indexing
                              tunnel: [w2681] -> w2679 mode=indexing
                              n1325 = Search and Replace String(input string=w2684, search string=",", replace string="." ("search string")) -> (result string=w2681:string)  [unwired: 5 in, 3 out]
                            }
                          }
                        }
                        frame "Punto" {
                          n1326 = for {
                            tunnel: w2686 -> [w2688] mode=indexing
                            tunnel: [w2687] -> w2685 mode=indexing
                            n1327 = for {
                              tunnel: w2688 -> [w2692] mode=indexing
                              tunnel: [w2689] -> w2687 mode=indexing
                              n1328 = Search and Replace String(input string=w2692, search string=".", replace string="," ("search string")) -> (result string=w2689:string)  [unwired: 5 in, 3 out]
                            }
                          }
                        }
                      }
                      n1329 = call-poly <vilib>:"Excel Easy Table.vi"("report in"=w2675, "start (0, 0)"=w2669, "text data"=w2666, "error in (no error)"=w2676) -> ("report out"=w2673:refnum<class "NI_report.lvclass">, "error out"=w2671:errorcluster)  [unwired: 7 in, 3 out]
                    }
                    frame "RES FINE PROVA A CARICO" {
                      n1330 = local read "TABELLA A CARICO"() -> (w2693:i16)
                      n1331 = Unbundle By Name(w2697) -> ("Res fin carico"=w2695:string[][])
                      n1332 = call <vilib>:"Excel Get Worksheet.vi"("report in"=w2707, "error in (no error)"=w2705, "name (\"\")"=w2703) -> ("report out"=w2708:refnum<class "NI_report.lvclass">, "error out"=w2709:errorcluster)  [unwired: 11 in]
                      n1333 = call "Fitra per tabella.vi"("TAB"=w2693, "dati in"=w2695) -> ("dati out"=w2694:string[][])  [unwired: 9 in]
                      n1334 = Build Array (concatenate)(string[] ["RES FINE CARICO"] ("element"), w2700, w2694) -> (w2698:string[][])
                      n1335 = case shown="\"Virgola\", Default" w2701 {
                        tunnel: w2698 -> [w2711 w2719]
                        tunnel: [w2710 w2718] -> w2699
                        frame "Virgola", Default {
                          n1336 = for {
                            tunnel: w2711 -> [w2713] mode=indexing
                            tunnel: [w2712] -> w2710 mode=indexing
                            n1337 = for {
                              tunnel: w2713 -> [w2717] mode=indexing
                              tunnel: [w2714] -> w2712 mode=indexing
                              n1338 = Search and Replace String(input string=w2717, search string=",", replace string="." ("search string")) -> (result string=w2714:string)  [unwired: 5 in, 3 out]
                            }
                          }
                        }
                        frame "Punto" {
                          n1339 = for {
                            tunnel: w2719 -> [w2721] mode=indexing
                            tunnel: [w2720] -> w2718 mode=indexing
                            n1340 = for {
                              tunnel: w2721 -> [w2725] mode=indexing
                              tunnel: [w2722] -> w2720 mode=indexing
                              n1341 = Search and Replace String(input string=w2725, search string=".", replace string="," ("search string")) -> (result string=w2722:string)  [unwired: 5 in, 3 out]
                            }
                          }
                        }
                      }
                      n1342 = call-poly <vilib>:"Excel Easy Table.vi"("report in"=w2708, "start (0, 0)"=w2702, "text data"=w2699, "error in (no error)"=w2709) -> ("report out"=w2706:refnum<class "NI_report.lvclass">, "error out"=w2704:errorcluster)  [unwired: 7 in, 3 out]
                    }
                    frame "DATI PROVA A CARICO" {
                      n1343 = local read "TABELLA A CARICO"() -> (w2731:i16)
                      n1344 = Unbundle By Name(w2733) -> ("A carico"=w2732:string[][])
                      n1345 = call "Fitra per tabella.vi"("TAB"=w2731, "dati in"=w2732) -> ("dati out"=w2729:string[][])  [unwired: 9 in]
                      n1346 = Build Array (concatenate)(string[] ["PROVA CARICO"] ("element"), w2727, w2729) -> (w2734:string[][])
                      n1347 = case shown="\"Virgola\", Default" w2736 {
                        tunnel: w2734 -> [w2746 w2754]
                        tunnel: [w2745 w2753] -> w2735
                        frame "Virgola", Default {
                          n1348 = for {
                            tunnel: w2746 -> [w2748] mode=indexing
                            tunnel: [w2747] -> w2745 mode=indexing
                            n1349 = for {
                              tunnel: w2748 -> [w2752] mode=indexing
                              tunnel: [w2749] -> w2747 mode=indexing
                              n1350 = Search and Replace String(input string=w2752, search string=",", replace string="." ("search string")) -> (result string=w2749:string)  [unwired: 5 in, 3 out]
                            }
                          }
                        }
                        frame "Punto" {
                          n1351 = for {
                            tunnel: w2754 -> [w2756] mode=indexing
                            tunnel: [w2755] -> w2753 mode=indexing
                            n1352 = for {
                              tunnel: w2756 -> [w2760] mode=indexing
                              tunnel: [w2757] -> w2755 mode=indexing
                              n1353 = Search and Replace String(input string=w2760, search string=".", replace string="," ("search string")) -> (result string=w2757:string)  [unwired: 5 in, 3 out]
                            }
                          }
                        }
                      }
                      n1354 = call <vilib>:"Excel Get Worksheet.vi"("report in"=w2742, "error in (no error)"=w2740, "name (\"\")"=w2738) -> ("report out"=w2743:refnum<class "NI_report.lvclass">, "error out"=w2744:errorcluster)  [unwired: 11 in]
                      n1355 = Matrix Size(0:w2729) -> (1:w2726:i32)  [unwired: 1 out]
                      n1356 = Decrement(x=w2726) -> (x-1=w2728:i32)
                      n1357 = call-poly <vilib>:"Excel Easy Table.vi"("report in"=w2743, "start (0, 0)"=w2737, "text data"=w2735, "error in (no error)"=w2744) -> ("report out"=w2741:refnum<class "NI_report.lvclass">, "error out"=w2739:errorcluster)  [unwired: 7 in, 3 out]
                      n1358 = Index Array(array=w2729, index (row)=w2728) -> ()  [unwired: 1 in, 1 out]
                    }
                    frame "DATI EQUILIBRIO TERMICO" {
                      n1359 = local read "TABELLA TERMICA"() -> (w2761:i16)
                      n1360 = Unbundle By Name(w2765) -> ("Riga eq termico"=w2763:string[][])
                      n1361 = call <vilib>:"Excel Get Worksheet.vi"("report in"=w2775, "error in (no error)"=w2773, "name (\"\")"=w2771) -> ("report out"=w2776:refnum<class "NI_report.lvclass">, "error out"=w2777:errorcluster)  [unwired: 11 in]
                      n1362 = call "Fitra per tabella.vi"("TAB"=w2761, "dati in"=w2763) -> ("dati out"=w2762:string[][])  [unwired: 9 in]
                      n1363 = Build Array (concatenate)(string[] ["EQUILIB TERMICO"] ("element"), w2768, w2762) -> (w2766:string[][])
                      n1364 = case shown="\"Virgola\", Default" w2769 {
                        tunnel: w2766 -> [w2779 w2787]
                        tunnel: [w2778 w2786] -> w2767
                        frame "Virgola", Default {
                          n1365 = for {
                            tunnel: w2779 -> [w2781] mode=indexing
                            tunnel: [w2780] -> w2778 mode=indexing
                            n1366 = for {
                              tunnel: w2781 -> [w2785] mode=indexing
                              tunnel: [w2782] -> w2780 mode=indexing
                              n1367 = Search and Replace String(input string=w2785, search string=",", replace string="." ("search string")) -> (result string=w2782:string)  [unwired: 5 in, 3 out]
                            }
                          }
                        }
                        frame "Punto" {
                          n1368 = for {
                            tunnel: w2787 -> [w2789] mode=indexing
                            tunnel: [w2788] -> w2786 mode=indexing
                            n1369 = for {
                              tunnel: w2789 -> [w2793] mode=indexing
                              tunnel: [w2790] -> w2788 mode=indexing
                              n1370 = Search and Replace String(input string=w2793, search string=".", replace string="," ("search string")) -> (result string=w2790:string)  [unwired: 5 in, 3 out]
                            }
                          }
                        }
                      }
                      n1371 = call-poly <vilib>:"Excel Easy Table.vi"("report in"=w2776, "start (0, 0)"=w2770, "text data"=w2767, "error in (no error)"=w2777) -> ("report out"=w2774:refnum<class "NI_report.lvclass">, "error out"=w2772:errorcluster)  [unwired: 7 in, 3 out]
                    }
                    frame "DATI PROVA TERMICA" {
                      n1372 = local read "TABELLA TERMICA"() -> (w2794:i16)
                      n1373 = Unbundle By Name(w2798) -> ("Termica"=w2796:string[][])
                      n1374 = call "Fitra per tabella.vi"("TAB"=w2794, "dati in"=w2796) -> ("dati out"=w2795:string[][])  [unwired: 9 in]
                      n1375 = Build Array (concatenate)(string[] ["PROVA TERMICA"] ("element"), w2801, w2795) -> (w2799:string[][])
                      n1376 = case shown="\"Virgola\", Default" w2802 {
                        tunnel: w2799 -> [w2812 w2820]
                        tunnel: [w2811 w2819] -> w2800
                        frame "Virgola", Default {
                          n1377 = for {
                            tunnel: w2812 -> [w2814] mode=indexing
                            tunnel: [w2813] -> w2811 mode=indexing
                            n1378 = for {
                              tunnel: w2814 -> [w2818] mode=indexing
                              tunnel: [w2815] -> w2813 mode=indexing
                              n1379 = Search and Replace String(input string=w2818, search string=",", replace string="." ("search string")) -> (result string=w2815:string)  [unwired: 5 in, 3 out]
                            }
                          }
                        }
                        frame "Punto" {
                          n1380 = for {
                            tunnel: w2820 -> [w2822] mode=indexing
                            tunnel: [w2821] -> w2819 mode=indexing
                            n1381 = for {
                              tunnel: w2822 -> [w2826] mode=indexing
                              tunnel: [w2823] -> w2821 mode=indexing
                              n1382 = Search and Replace String(input string=w2826, search string=".", replace string="," ("search string")) -> (result string=w2823:string)  [unwired: 5 in, 3 out]
                            }
                          }
                        }
                      }
                      n1383 = call <vilib>:"Excel Get Worksheet.vi"("report in"=w2808, "error in (no error)"=w2806, "name (\"\")"=w2804) -> ("report out"=w2809:refnum<class "NI_report.lvclass">, "error out"=w2810:errorcluster)  [unwired: 11 in]
                      n1384 = call-poly <vilib>:"Excel Easy Table.vi"("report in"=w2809, "start (0, 0)"=w2803, "text data"=w2800, "error in (no error)"=w2810) -> ("report out"=w2807:refnum<class "NI_report.lvclass">, "error out"=w2805:errorcluster)  [unwired: 7 in, 3 out]
                    }
                    frame "RESISTENZE PROVA TERMICA" {
                      n1385 = Unbundle By Name(w2831) -> ("Resistenze termica"=w2829:string[][])
                      n1386 = local read "TABELLA TERMICA"() -> (w2827:i16)
                      n1387 = call "Fitra per tabella.vi"("TAB"=w2827, "dati in"=w2829) -> ("dati out"=w2828:string[][])  [unwired: 9 in]
                      n1388 = Build Array (concatenate)(string[] ["RESISTENZE TERMICA"] ("element"), w2834, w2828) -> (w2832:string[][])
                      n1389 = case shown="\"Virgola\", Default" w2835 {
                        tunnel: w2832 -> [w2845 w2853]
                        tunnel: [w2844 w2852] -> w2833
                        frame "Virgola", Default {
                          n1390 = for {
                            tunnel: w2845 -> [w2847] mode=indexing
                            tunnel: [w2846] -> w2844 mode=indexing
                            n1391 = for {
                              tunnel: w2847 -> [w2851] mode=indexing
                              tunnel: [w2848] -> w2846 mode=indexing
                              n1392 = Search and Replace String(input string=w2851, search string=",", replace string="." ("search string")) -> (result string=w2848:string)  [unwired: 5 in, 3 out]
                            }
                          }
                        }
                        frame "Punto" {
                          n1393 = for {
                            tunnel: w2853 -> [w2855] mode=indexing
                            tunnel: [w2854] -> w2852 mode=indexing
                            n1394 = for {
                              tunnel: w2855 -> [w2859] mode=indexing
                              tunnel: [w2856] -> w2854 mode=indexing
                              n1395 = Search and Replace String(input string=w2859, search string=".", replace string="," ("search string")) -> (result string=w2856:string)  [unwired: 5 in, 3 out]
                            }
                          }
                        }
                      }
                      n1396 = call <vilib>:"Excel Get Worksheet.vi"("report in"=w2841, "error in (no error)"=w2839, "name (\"\")"=w2837) -> ("report out"=w2842:refnum<class "NI_report.lvclass">, "error out"=w2843:errorcluster)  [unwired: 11 in]
                      n1397 = call-poly <vilib>:"Excel Easy Table.vi"("report in"=w2842, "start (0, 0)"=w2836, "text data"=w2833, "error in (no error)"=w2843) -> ("report out"=w2840:refnum<class "NI_report.lvclass">, "error out"=w2838:errorcluster)  [unwired: 7 in, 3 out]
                    }
                    frame "RIGA DATI CMAX" {
                      n1398 = local read "TABELLA CMECC"() -> (w2860:i16)
                      n1399 = Unbundle By Name(w2864) -> ("Riga Cmax"=w2862:string[][])
                      n1400 = call <vilib>:"Excel Get Worksheet.vi"("report in"=w2874, "error in (no error)"=w2872, "name (\"\")"=w2870) -> ("report out"=w2875:refnum<class "NI_report.lvclass">, "error out"=w2876:errorcluster)  [unwired: 11 in]
                      n1401 = call "Fitra per tabella.vi"("TAB"=w2860, "dati in"=w2862) -> ("dati out"=w2861:string[][])  [unwired: 9 in]
                      n1402 = Build Array (concatenate)(string[] ["RIGA CMAX"] ("element"), w2867, w2861) -> (w2865:string[][])
                      n1403 = case shown="\"Virgola\", Default" w2868 {
                        tunnel: w2865 -> [w2878 w2886]
                        tunnel: [w2877 w2885] -> w2866
                        frame "Virgola", Default {
                          n1404 = for {
                            tunnel: w2878 -> [w2880] mode=indexing
                            tunnel: [w2879] -> w2877 mode=indexing
                            n1405 = for {
                              tunnel: w2880 -> [w2884] mode=indexing
                              tunnel: [w2881] -> w2879 mode=indexing
                              n1406 = Search and Replace String(input string=w2884, search string=",", replace string="." ("search string")) -> (result string=w2881:string)  [unwired: 5 in, 3 out]
                            }
                          }
                        }
                        frame "Punto" {
                          n1407 = for {
                            tunnel: w2886 -> [w2888] mode=indexing
                            tunnel: [w2887] -> w2885 mode=indexing
                            n1408 = for {
                              tunnel: w2888 -> [w2892] mode=indexing
                              tunnel: [w2889] -> w2887 mode=indexing
                              n1409 = Search and Replace String(input string=w2892, search string=".", replace string="," ("search string")) -> (result string=w2889:string)  [unwired: 5 in, 3 out]
                            }
                          }
                        }
                      }
                      n1410 = call-poly <vilib>:"Excel Easy Table.vi"("report in"=w2875, "start (0, 0)"=w2869, "text data"=w2866, "error in (no error)"=w2876) -> ("report out"=w2873:refnum<class "NI_report.lvclass">, "error out"=w2871:errorcluster)  [unwired: 7 in, 3 out]
                    }
                    frame "DATI CMECCANICA" {
                      n1411 = local read "TABELLA CMECC"() -> (w2893:i16)
                      n1412 = Unbundle By Name(w2897) -> ("Cmecc"=w2895:string[][])
                      n1413 = call "Fitra per tabella.vi"("TAB"=w2893, "dati in"=w2895) -> ("dati out"=w2894:string[][])  [unwired: 9 in]
                      n1414 = Build Array (concatenate)(string[] ["PROVA CMECC"] ("element"), w2900, w2894) -> (w2898:string[][])
                      n1415 = case shown="\"Virgola\", Default" w2901 {
                        tunnel: w2898 -> [w2911 w2919]
                        tunnel: [w2910 w2918] -> w2899
                        frame "Virgola", Default {
                          n1416 = for {
                            tunnel: w2911 -> [w2913] mode=indexing
                            tunnel: [w2912] -> w2910 mode=indexing
                            n1417 = for {
                              tunnel: w2913 -> [w2917] mode=indexing
                              tunnel: [w2914] -> w2912 mode=indexing
                              n1418 = Search and Replace String(input string=w2917, search string=",", replace string="." ("search string")) -> (result string=w2914:string)  [unwired: 5 in, 3 out]
                            }
                          }
                        }
                        frame "Punto" {
                          n1419 = for {
                            tunnel: w2919 -> [w2921] mode=indexing
                            tunnel: [w2920] -> w2918 mode=indexing
                            n1420 = for {
                              tunnel: w2921 -> [w2925] mode=indexing
                              tunnel: [w2922] -> w2920 mode=indexing
                              n1421 = Search and Replace String(input string=w2925, search string=".", replace string="," ("search string")) -> (result string=w2922:string)  [unwired: 5 in, 3 out]
                            }
                          }
                        }
                      }
                      n1422 = call <vilib>:"Excel Get Worksheet.vi"("report in"=w2907, "error in (no error)"=w2905, "name (\"\")"=w2903) -> ("report out"=w2908:refnum<class "NI_report.lvclass">, "error out"=w2909:errorcluster)  [unwired: 11 in]
                      n1423 = call-poly <vilib>:"Excel Easy Table.vi"("report in"=w2908, "start (0, 0)"=w2902, "text data"=w2899, "error in (no error)"=w2909) -> ("report out"=w2906:refnum<class "NI_report.lvclass">, "error out"=w2904:errorcluster)  [unwired: 7 in, 3 out]
                    }
                    frame "LEGENDA COLLAUDI CONFRONTO" {
                      n1424 = call <vilib>:"Excel Get Worksheet.vi"("report in"=w2932, "error in (no error)"=w2930, "name (\"\")"=w2927) -> ("report out"=w2933:refnum<class "NI_report.lvclass">, "error out"=w2934:errorcluster)  [unwired: 11 in]
                      n1425 = call-poly <vilib>:"Excel Easy Table.vi"("report in"=w2933, "start (0, 0)"=w2928, "text data"=w2926, "error in (no error)"=w2934) -> ("report out"=w2931:refnum<class "NI_report.lvclass">, "error out"=w2929:errorcluster)  [unwired: 7 in, 3 out]
                    }
                    frame "CALCOLI RENDIMENTO" {
                      n1426 = property on="DETERMINAZIONE DEL RENDIMENTO" class="MCListbox (strict)"() -> ("ItemNames"=w2937:string[][])  [unwired: 2 in, 2 out]
                      n1427 = case shown="\"Virgola\", Default" w2935 {
                        tunnel: w2937 -> [w2947 w2955]
                        tunnel: [w2946 w2954] -> w2936
                        frame "Virgola", Default {
                          n1428 = for {
                            tunnel: w2947 -> [w2949] mode=indexing
                            tunnel: [w2948] -> w2946 mode=indexing
                            n1429 = for {
                              tunnel: w2949 -> [w2953] mode=indexing
                              tunnel: [w2950] -> w2948 mode=indexing
                              n1430 = Search and Replace String(input string=w2953, search string=",", replace string="." ("search string")) -> (result string=w2950:string)  [unwired: 5 in, 3 out]
                            }
                          }
                        }
                        frame "Punto" {
                          n1431 = for {
                            tunnel: w2955 -> [w2957] mode=indexing
                            tunnel: [w2956] -> w2954 mode=indexing
                            n1432 = for {
                              tunnel: w2957 -> [w2961] mode=indexing
                              tunnel: [w2958] -> w2956 mode=indexing
                              n1433 = Search and Replace String(input string=w2961, search string=".", replace string="," ("search string")) -> (result string=w2958:string)  [unwired: 5 in, 3 out]
                            }
                          }
                        }
                      }
                      n1434 = call <vilib>:"Excel Get Worksheet.vi"("report in"=w2943, "error in (no error)"=w2942, "name (\"\")"=w2941) -> ("report out"=w2944:refnum<class "NI_report.lvclass">, "error out"=w2945:errorcluster)  [unwired: 11 in]
                      n1435 = call-poly <vilib>:"Excel Easy Table.vi"("report in"=w2944, "start (0, 0)"=w2940, "text data"=w2936, "error in (no error)"=w2945) -> ("report out"=w2938:refnum<class "NI_report.lvclass">, "error out"=w2939:errorcluster)  [unwired: 7 in, 3 out]
                    }
                  }
                }
                n1436 = Unbundle By Name(w2372) -> ("Generica"=w2362:string[][])
                n1437 = property class="Slide (strict)"(reference=w2385, error in=w2366, "Value"=40.0) -> (reference out=w2383:refnum<vi>)  [unwired: 1 out]
                n1438 = local read "ETICHETTE"() -> (w2373:string[])
                n1439 = call "Fitra per tabella.vi"("TAB"=w2360, "dati in"=w2362) -> ("dati out"=w2361:string[][])  [unwired: 9 in]
                n1440 = call "Esporta generiche.vi"("Array"=w2361, "Nomi colonne"=w2373, "error in (no error)"=w2366, "sep. decimale numeri esportati"=w2370, "Nome fogli"="Nome fogli GENERICHE", "NI_report in"=w2374) -> ("error out"=w2365:errorcluster, "NI_report out"=w2369:refnum<class "NI_report.lvclass">)  [unwired: 3 in, 1 out]
                n1441 = Empty Array?(array=w2324) -> (empty?=w2323:bool)
                n1442 = property class="Slide (strict)"(reference=w2383, error in=w2365, "Value"=50.0) -> (reference out=w2381:refnum<vi>)  [unwired: 1 out]
                n1443 = case shown="False" w2323 {
                  tunnel: w2369 -> [w2397 w2411]
                  tunnel: [w2396 w2411] -> w2368
                  tunnel: w2365 -> [w2395 w2410]
                  tunnel: [w2394 w2410] -> w2364
                  tunnel: w2324 -> [w2393 _]
                  frame False {
                    n1444 = for {
                      shift-right: [w2409] -> w2396
                      shift-left: w2397 -> [w2403]
                      shift-right: [w2408] -> w2394
                      shift-left: w2395 -> [w2405]
                      tunnel: w2393 -> [w2407] mode=indexing
                      n1445 = Unbundle By Name(w2407) -> ("path"=w2406:path, "Impostazioni esport..position (Excel)"=w2398:cluster{"row":i32, "column":i32}, "Impostazioni esport..Nome foglio (Excel)"=w2401:string)
                      n1446 = call <vilib>:"Excel Get Worksheet.vi"("report in"=w2403, "error in (no error)"=w2405, "name (\"\")"=w2401) -> ("report out"=w2402:refnum<class "NI_report.lvclass">, "error out"=w2404:errorcluster)  [unwired: 11 in]
                      n1447 = Bundle By Name(cluster=T25 {"position (Excel)"={"row"=0, "column"=0}, "name (Excel)"="", "bookmark (Word)"=""} ("MS Office parameters"), "position (Excel)"=w2398) -> (w2399:T25)
                      n1448 = call-poly <vilib>:"Append Image to Report.vi"("report in"=w2402, "MS Office parameters"=w2399, "path or URL of image"=w2406, "error in (no error)"=w2404) -> ("report out"=w2409:refnum<class "NI_report.lvclass">, "error out"=w2408:errorcluster)  [unwired: 8 in, 2 out]
                    }
                  }
                  frame True {
                  }
                }
                n1449 = property class="Slide (strict)"(reference=w2381, error in=w2364, "Value"=70.0) -> (reference out=w2379:refnum<vi>)  [unwired: 1 out]
                n1450 = Not(x=w2325) -> (.not. x?=w2327:bool)
                n1451 = And(x="EXCEL", y=w2327) -> (x .and. y?=w2328:bool)
                n1452 = Or(x=w2325, y="PDF") -> (x .or. y?=w2326:bool)
                n1453 = case shown="True" w2328 {
                  tunnel: w2368 -> [w2413 w2418]
                  tunnel: w2364 -> [w2412 w2417]
                  tunnel: [w2413 w2416] -> w2343
                  tunnel: [w2412 w2414] -> w2342
                  tunnel: w2333 -> [_ w2415]
                  tunnel: [w2412 w2414] -> w2331
                  frame False {
                  }
                  frame True {
                    n1454 = disable-structure shown="Enabled" {
                      disable-tunnel: w2418 -> [w2423 w2426]
                      disable-tunnel: w2417 -> [w2422 w2425]
                      disable-tunnel: [w2421 w2426] -> w2416
                      disable-tunnel: w2415 -> [w2420 _]
                      disable-tunnel: [w2419 w2425] -> w2414
                      frame Enabled {
                        n1455 = call-dynamic "Save Report to File.vi"("report in"=w2423, "report file path"=w2420, "prompt to replace? (F)"=TRUE, "error in (no error)"=w2422) -> ("report out"=w2421:refnum<class "NI_report.lvclass">, "error out"=w2419:errorcluster)  [unwired: 10 in]
                      }
                      frame Disabled {
                      }
                    }
                  }
                }
                n1456 = Path To String(path=w2333) -> (string=w2334:string)
                n1457 = property class="Slide (strict)"(reference=w2379, error in=w2342, "Value"=80.0) -> ()  [unwired: 2 out]
                n1458 = Search and Replace String(input string=w2334, search string=".xls", replace string=".pdf" ("replace string (\"\")")) -> (result string=w2339:string, error out=w2340:errorcluster)  [unwired: 5 in, 2 out]
                n1459 = Search and Replace String(input string=w2339, search string=".xlsx", replace string=".pdf" ("replace string (\"\")"), error in=w2340) -> (result string=w2341:string)  [unwired: 4 in, 3 out]
                n1460 = String To Path(string=w2341) -> (path=w2332:path)
                n1461 = case shown="True" w2326 {
                  tunnel: [w2427 w2431] -> w2345
                  tunnel: [w2428 w2432] -> w2344
                  tunnel: w2343 -> [w2428 w2434]
                  tunnel: w2331 -> [w2427 w2435]
                  tunnel: w2332 -> [_ w2429]
                  frame False {
                  }
                  frame True {
                    w2430 = 0 items=["xlTypePDF", "xlTypeXPS"] ("Type")
                    n1462 = call <vilib>:"Excel Get ActiveX References.vi"("report in"=w2434, "error in (no error)"=w2435) -> ("report out"=w2432:refnum<class "NI_report.lvclass">, "Excel._Workbook"=w2433:refnum<k7>, "error out"=w2431:errorcluster)  [unwired: 7 in, 4 out]
                    n1463 = invoke class="_Workbook" method="ExportAsFixedFormat"(reference=w2433, "Type"=w2430, "Filename"=w2429) -> ()  [unwired: 10 in, 13 out]
                  }
                }
                n1464 = disable-structure shown="Enabled" {
                  disable-tunnel: w2345 -> [w2392 _]
                  disable-tunnel: w2344 -> [w2391 _]
                  frame Enabled {
                    n1465 = call-dynamic "Dispose Report.vi"("report in"=w2391, "error in (no error)"=w2392) -> ()  [unwired: 13 in, 1 out]
                  }
                  frame Disabled {
                  }
                }
              }
              frame #3 {
                n1466 = flat-sequence {
                  tunnel: w2964 -> [w2969]
                  tunnel: [w2968] -> w2967
                  tunnel: [w2971] -> w2966
                  tunnel: w2967 -> [w2971]
                  tunnel: w2966 -> [w2974]
                  tunnel: [w2974] -> w2965
                  tunnel: w2962 -> [w2973]
                  tunnel: w2965 -> [w2978]
                  tunnel: [w2977] -> w2963
                  frame #0 {
                    n1467 = property class="Slide (strict)"(reference=w2969, "Value"=90.0) -> (reference out=w2968:refnum<vi>)  [unwired: 1 in, 1 out]
                  }
                  frame #1 {
                    n1468 = Wait (ms)(milliseconds to wait=u32 1000) -> ()  [unwired: 1 out]
                  }
                  frame #2 {
                    n1469 = for {
                      tunnel: w2973 -> [w2976] mode=indexing
                      n1470 = Unbundle By Name(w2976) -> ("path"=w2975:path)
                      n1471 = Delete(path (use dialog)=w2975) -> ()  [unwired: 4 in, 3 out]
                    }
                  }
                  frame #3 {
                    n1472 = property class="Slide (strict)"(reference=w2978, "Value"=100.0) -> (reference out=w2977:refnum<vi>)  [unwired: 1 in, 1 out]
                  }
                }
              }
            }
            n1473 = flat-sequence {
              tunnel: w2205 -> [w2981]
              tunnel: [w2981] -> w2204
              tunnel: w2204 -> [w2984]
              tunnel: w2202 -> [w2985]
              frame #0 {
                n1474 = Wait (ms)(milliseconds to wait=u32 1000) -> ()  [unwired: 1 out]
              }
              frame #1 {
                n1475 = property class="Slide (strict)"(reference=w2984, "Value"=0.0) -> ()  [unwired: 1 in, 2 out]
                n1476 = property on="REPORT EXCEL" class="Bool (strict)"("Visible"=TRUE) -> ()  [unwired: 2 in, 2 out]
              }
              frame #2 {
                n1477 = case shown="True" w2985 {
                  frame False {
                  }
                  frame True {
                    n1478 = property on="exit" class="Bool (strict)"("Val(Sgnl)"=TRUE ("Value (Signaling)")) -> ()  [unwired: 2 in, 2 out]
                  }
                }
              }
            }
          }
          frame True {
            n1479 = One Button Dialog(message="Creazione report annullata dall'utente.") -> ()  [unwired: 1 in, 1 out]
          }
        }
      }
      frame "exit" {
      }
    }
    "Numeric" <- w327
  }
